vi "BAES RI Retrieval from PAS with LABVIEW.vi"() -> ()   [LabVIEW 2013]
uses:
  BaesDataTypeDefinition.ctl
  ReadBaesDataTypeDefinition.ctl
  ParticleDistributionData.ctl
  GeneralDataForRIRetrieval.ctl
  <vilib>/Native 3D Graph/xcontrol/3DPC_SurfacePlot.xctl
  <vilib>/Native 3D Graph/classes/Surface/Surface.lvclass
  RIandRIMCResults.ctl
  <vilib>/gmath/NumericalOptimization/stopping criteria.ctl
  <vilib>/Analysis/1siggen.llb/Ramp Pattern by Samples.vi
  <vilib>/gmath/NumericalOptimization/Conjugate Gradient.vi
  <vilib>/Utility/file.llb/Write To Spreadsheet File (string).vi
  <vilib>/Analysis/Matrix/Numeric/Conversions/Matrix To Array - RM.vi
  <vilib>/gmath/statdist.llb/Normal Inverse CDF.vi
  <vilib>/imath/engines/lvmath2/RunTimeEngine/ErrorHandling/NIMS_Finalize Error.vi
  <vilib>/imath/engines/lvmath2/RunTimeEngine/RangeToken/NIMS_Range_R2 - Float.vi
  <instcachedir>/0/NIMS_Range_R2 - Float_E19924E36A3948A4B33043226480F83C.lvgen/NIMS_Range_R2 - Float_E19924E36A3948A4B33043226480F83C_000.vi
  <vilib>/imath/engines/lvmath2/RunTimeEngine/NodeEndStatement/NIMS_NodeEndStatement_Output.vi
  <instcachedir>/0/NIMS_NodeEndStatement_Output_53EC0D466D134D7ABD903AC30B43404B.lvgen/NIMS_NodeEndStatement_Output_53EC0D466D134D7ABD903AC30B43404B_002.vi
  <vilib>/imath/engines/lvmath2/RunTimeEngine/CommandStatement/MC_CommandStatement_break.vi
  <vilib>/imath/engines/lvmath2/RunTimeSupport/NIMS_Error if Not Equal.vi
  <instcachedir>/0/NIMS_Error if Not Equal_902F5D2649E64F5087A1EF57C55C58AB.lvgen/NIMS_Error if Not Equal_902F5D2649E64F5087A1EF57C55C58AB_000.vi
  <vilib>/imath/engines/lvmath2/RunTimeEngine/IndexRead/NIMS M($,S).vi
  <instcachedir>/0/NIMS M($,S)_3E5749BBB62E49528D4765A77F1F6D98.lvgen/NIMS M($,S)_3E5749BBB62E49528D4765A77F1F6D98_000.vi
  <vilib>/imath/engines/lvmath2/RunTimeEngine/RowToken/NIMS_RowToken_M_CV.vi
  <instcachedir>/0/NIMS_RowToken_M_CV_4FFFB80A1A2C4A06BEF1E2564C6BAFA4.lvgen/NIMS_RowToken_M_CV_4FFFB80A1A2C4A06BEF1E2564C6BAFA4_000.vi
  <vilib>/imath/engines/lvmath2/RunTimeEngine/ErrorHandling/NIMS_Create Error From Enums.vi
  <vilib>/gmath/NI_Gmath.lvlib
  <vilib>/Analysis/Matrix/NI_Matrix.lvlib
  <vilib>/Analysis/NI_AALBase.lvlib
panel:
  out "Array":dbl[][](array[numeric])
  out "Global Min":T1
  out "GlobalMinimumStruct":T2(array[cluster])
  out "n-k matrix":cluster{dbl[], dbl[]}(graph)
  in  "k_samples":dbl=1.0 caption="Samples"
  in  "k_finish":dbl=5.0 caption="Finish"
  in  "k_start":dbl=-5.0 caption="Start"
  in  "n_samples":dbl=0.1 caption="Samples"
  in  "n_finish":dbl=1.2 caption="Finish"
  in  "n_start":dbl=0.8 caption="Start"
  in  "Find Global Minima":bool
  in  "Starting Guess - Imag":dbl=0.1
  in  "Starting Guess -Real":dbl=1.5
  in  "autoscale":bool
  in  "Correct SMPS sizes to selected Sizes":bool
  out "Peak Center":dbl[](array[numeric])=[215.23700286959917, 239.46777469280113, 266.53712087613405, 296.56972011152817, 329.9933867048781, 354.3213922159785, 380.24064147372457, 407.9273850466716, 436.86507564817134]
  in  "method":i32(ring)=3 items=["nearest", "linear", "spline", "cubic Hermite", "Lagrange"]
  out "yi out":dbl[][](array[numeric])=[[0.0, 0.0, 0.0, 0.0, 0.0, 0.0, 0.0, 0.0, 0.0], [0.0, 0.0, 0.0, 0.0, 0.0, 0.0, 0.0, 0.0, 0.0], [0.0, 0.0, 0.0, 0.0, 0.0, 0.0, 0.0, 0.0, 0.0], [0.0, 0.0, 0.0, 0.0, 0.0, 0.0, 0.0, 0.0, 0.0], [0.0, 0.0, 0.0, 0.0, 0.0, 0.0, 0.0, 0.0, 0.0], [0.0, 0.0, 0.0, 0.0, 0.0, 0.0, 0.0, 0.0, 0.0], [0.0, 0.0, 0.0, 0.0, 0.0, 0.0, 0.0, 0.0, 0.0], [0.0, 0.0, 0.0, 0.0, 0.0, 0.0, 0.0, 0.0, 0.0], [0.0, 0.0, 0.0, 0.0, 0.0, 0.0, 0.0, 0.0, 0.0], [0.0, 0.0, 0.0, 0.0, 0.0, 0.0, 0.0, 0.0, 0.0], [0.0, 0.0, 0.0, 0.0, 0.0, 0.0, 0.0, 0.0, 0.0], [0.0, 0.0, 0.0, 0.0, 0.0, 0.0, 0.0, 0.0, 0.0], [0.0, 0.0, 0.0, 0.0, 0.0, 0.0, 0.0, 0.0, 0.0], [0.0, 0.0, 0.0, 0.0, 0.0, 0.0, 0.0, 0.0, 0.0], [0.0, 0.0, 0.0, 0.0, 0.0, 0.0, 0.0, 0.0, 0.0], [0.0, 0.0, 0.0, 0.0, 0.0, 0.0, 0.0, 0.0, 0.0], [0.002995533043634161, 0.0, 0.0, 0.0, 0.0, 0.0, 0.0, 0.0, 0.0], [0.025840856539342556, 0.0, 0.0, 0.0, 0.0, 0.0, 0.0, 0.0, 0.0], [0.09627433030958367, 0.0, 0.0, 0.0, 0.0, 0.0, 0.0, 0.0, 0.0], [0.20114413818462407, 0.003679405258454903, 0.0, 0.0, 0.0, 0.0, 0.0, 0.0, 0.0], [0.24542760207823705, 0.030110785948579594, 0.0, 0.0, 0.0, 0.0, 0.0, 0.0, 0.0], [0.19935011876678227, 0.10676097365384078, 0.0, 0.0, 0.0, 0.0, 0.0, 0.0, 0.0], [0.10027077337218139, 0.21292413302969826, 0.0033748243651170722, 0.0, 0.0, 0.0, 0.0, 0.0, 0.0], [0.02900603131815543, 0.252436330373865, 0.02890039600275283, 0.0, 0.0, 0.0, 0.0, 0.0, 0.0], [0.0039798778324419744, 0.1962993842174311, 0.10425475468568692, 0.0, 0.0, 0.0, 0.0, 0.0, 0.0], [0.0, 0.09510810120556674, 0.2127509720448336, 0.003204303022032701, 0.0, 0.0, 0.0, 0.0, 0.0], [0.0, 0.026788275767934952, 0.25443516550640577, 0.028222420464123123, 0.0, 0.0, 0.0, 0.0, 0.0], [0.0, 0.0036138798422305257, 0.20572070395413536, 0.10336691645150534, 0.0, 0.0, 0.0, 0.0, 0.0], [0.0, 0.0, 0.10385751888143922, 0.21356874773842194, 0.003345015757771727, 0.0, 0.0, 0.0, 0.0], [0.0, 0.0, 0.03184137129301377, 0.25514474611865134, 0.02938228217938827, 0.0, 0.0, 0.0, 0.0], [0.0014956304497509467, 0.0, 0.005324689051489316, 0.21179320089555217, 0.10705199934528585, 0.003308736710887511, 0.0, 0.0, 0.0], [0.006181204689297098, 0.0, 0.0, 0.10947088728935564, 0.21880478513266646, 0.029404152563977024, 0.0, 0.0, 0.0], [0.014779079751943505, 0.0, 0.0, 0.0351443521735081, 0.2573967125709004, 0.10811744003531051, 0.004055473967709127, 0.0, 0.0], [0.021873123606276416, 0.0, 0.0, 0.00645421284142625, 0.21311979554910082, 0.21949012820871305, 0.03249660231234976, 0.0, 0.0], [0.020938671287516166, 0.002941447778294588, 0.0, 0.0005784696243201418, 0.11000745576713801, 0.2570127905092043, 0.11420156491259865, 0.004251138588627886, 0.0], [0.014150903231161319, 0.00918486371676828, 0.0, 0.0, 0.036185400505208645, 0.21598258772382448, 0.22683349675845424, 0.03241034304426709, 0.0], [0.005998151011193356, 0.016563944732687075, 0.0, 0.0, 0.007021566470141746, 0.11238428494392888, 0.25641274621663857, 0.11266793086437756, 0.004147715999403451], [0.0015120995486811858, 0.017797923247623602, 0.001492807625783663, 0.0, 0.0007094205616598339, 0.037396339870968194, 0.21111602466052512, 0.22428037538775147, 0.031085439808444255], [0.0, 0.01329593538708705, 0.005201029958243257, 0.0, 0.0, 0.007536234728094553, 0.10787117985635983, 0.25568882442612334, 0.11065902188610582], [0.0, 0.00635541490586478, 0.010415971194231972, 0.0, 0.0, 0.0008190951722994508, 0.03536648135652447, 0.21469636352155314, 0.2221123992215679], [0.0010729774499575713, 0.0019363898629268694, 0.01277891881575932, 0.0006807013617405569, 0.0, 0.0, 0.007025068509258474, 0.10969810395513567, 0.25508407775997943], [0.002057300309839938, 0.0, 0.010740838502774176, 0.002649342768284491, 0.0, 0.0, 0.0007440549395453882, 0.03615143628832095, 0.216785934587122], [0.002474950875894475, 0.0, 0.006120821318984597, 0.006052131853820764, 0.0, 0.0, 0.0, 0.007394514918229318, 0.11122539130067338], [0.002060729815382503, 0.0, 0.002286068305636173, 0.008519468407529212, 0.0, 0.0, 0.0, 0.0008550654797584019, 0.03853326504170029], [0.0011159165281229126, 0.0009250356514019637, 0.0005031484937129974, 0.007827186354841077, 0.0010483084611445424, 0.0, 0.0, 0.0, 0.008221211137071305], [0.0, 0.0013182032160797494, 0.0, 0.0048751624944381525, 0.002846930380238516, 0.0, 0.0, 0.0, 0.0009934611660537788], [0.0, 0.0011832812074649155, 0.0, 0.0019419202748162476, 0.004454066932151218, 0.0, 0.0, 0.0, 0.0], [0.0, 0.0007762909961994142, 0.0, 0.0005058298656327597, 0.004488441198541657, 0.001576949269729668, 0.0, 0.0, 0.0], [0.0, 0.0, 0.0, 0.0, 0.0029347814148206284, 0.002346089545272472, 0.0, 0.0, 0.0], [0.0, 0.0, 0.0, 0.0, 0.0012030377738417415, 0.00231674366991226, 0.0007291026037730795, 0.0, 0.0], [0.0, 0.0, 0.0, 0.0, 0.0, 0.0015886617028698508, 0.0011333656105798114, 0.0, 0.0], [0.0, 0.0, 0.0, 0.0, 0.0, 0.0007197653450079487, 0.0011589853888717718, 0.0, 0.0], [0.0, 0.0, 0.0, 0.0, 0.0, 0.0, 0.0008558529068117928, 0.0005237679257223164, 0.0], [0.0, 0.0, 0.0, 0.0, 0.0, 0.0, 0.0, 0.0007042968505584731, 0.0], [0.0, 0.0, 0.0, 0.0, 0.0, 0.0, 0.0, 0.000677838749574469, 0.0], [0.0, 0.0, 0.0, 0.0, 0.0, 0.0, 0.0, 0.0, 0.000518938219565122], [0.0, 0.0, 0.0, 0.0, 0.0, 0.0, 0.0, 0.0, 0.0006331438723132111]]
  out "SMPS":T3(graph)=[{"Ramp Pattern"=[105.5, 109.4, 113.4, 117.6, 121.9, 126.3, 131.0, 135.8, 140.7, 145.9, 151.2, 156.8, 162.5, 168.5, 174.7, 181.1, 187.7, 194.6, 201.7, 209.1, 216.7, 224.7, 232.9, 241.4, 250.3, 259.5, 269.0, 278.8, 289.0, 299.6, 310.6, 322.0, 333.8, 346.0, 358.7, 371.8, 385.4, 399.5, 414.2, 429.4, 445.1, 461.4, 478.3, 495.8, 514.0, 532.8, 552.3, 572.5, 593.5, 615.3, 637.8, 661.2, 685.4, 710.5, 736.5, 763.5, 791.5], "Extinction"=[0.0, 0.0, 0.0, 0.0, 0.0, 0.0, 0.0, 0.0, 0.0, 0.0, 0.0, 0.0, 0.0, 0.0, 0.0, 0.0, 0.0, 0.0, 0.0, 0.0, 0.0, 0.0, 0.0, 0.0, 0.0, 0.0, 0.0, 0.0, 0.0, 0.0, 0.0, 0.0, 0.0, 0.0, 0.0, 0.0, 0.004147715999403451, 0.031085439808444255, 0.11065902188610582, 0.2221123992215679, 0.25508407775997943, 0.216785934587122, 0.11122539130067338, 0.03853326504170029, 0.008221211137071305, 0.0009934611660537788, 0.0, 0.0, 0.0, 0.0, 0.0, 0.0, 0.0, 0.0, 0.0, 0.000518938219565122, 0.0006331438723132111]}, {"Ramp Pattern"=[105.5, 109.4, 113.4, 117.6, 121.9, 126.3, 131.0, 135.8, 140.7, 145.9, 151.2, 156.8, 162.5, 168.5, 174.7, 181.1, 187.7, 194.6, 201.7, 209.1, 216.7, 224.7, 232.9, 241.4, 250.3, 259.5, 269.0, 278.8, 289.0, 299.6, 310.6, 322.0, 333.8, 346.0, 358.7, 371.8, 385.4, 399.5, 414.2, 429.4, 445.1, 461.4, 478.3, 495.8, 514.0, 532.8, 552.3, 572.5, 593.5, 615.3, 637.8, 661.2, 685.4, 710.5, 736.5, 763.5, 791.5], "Extinction"=[0.0, 0.0, 0.0, 0.0, 0.0, 0.0, 0.0, 0.0, 0.0, 0.0, 0.0, 0.0, 0.0, 0.0, 0.0, 0.0, 0.0, 0.0, 0.0, 0.0, 0.0, 0.0, 0.0, 0.0, 0.0, 0.0, 0.0, 0.0, 0.0, 0.0, 0.0, 0.0, 0.0, 0.0, 0.0, 0.000717254, 0.0123831, 0.0638696, 0.166954, 0.256206, 0.250783, 0.158589, 0.0675111, 0.0180047, 0.00271755, 0.000182617, 0.0, 0.0, 0.0, 0.0, 0.0, 1.197e-05, 6.86901e-05, 0.000249565, 0.000468067, 0.00056712, 0.000716313]}]
  in  "ShiftSMPStoSizes":bool
  out "Size Distribution":T3(graph)=[{"Ramp Pattern"=[105.5, 109.4, 113.4, 117.6, 121.9, 126.3, 131.0, 135.8, 140.7, 145.9, 151.2, 156.8, 162.5, 168.5, 174.7, 181.1, 187.7, 194.6, 201.7, 209.1, 216.7, 224.7, 232.9, 241.4, 250.3, 259.5, 269.0, 278.8, 289.0, 299.6, 310.6, 322.0, 333.8, 346.0, 358.7, 371.8, 385.4, 399.5, 414.2, 429.4, 445.1, 461.4, 478.3, 495.8, 514.0, 532.8, 552.3, 572.5, 593.5, 615.3, 637.8, 661.2, 685.4, 710.5, 736.5, 763.5, 791.5], "Extinction"=[0.0, 0.0, 0.0, 0.0, 0.0, 0.0, 0.0, 0.0, 0.0, 0.0, 0.00602144, 0.0440621, 0.137641, 0.242033, 0.26037, 0.1769, 0.0750014, 0.0175727, 0.00179137, 0.0, 0.0, 0.0, 0.0, 0.000380957, 0.00237282, 0.00642719, 0.0101183, 0.00943116, 0.0057312, 0.00222174, 0.000458212, 6.03629e-05, 0.000103363, 0.000252222, 0.000379412, 0.000345309, 0.000218451, 8.10505e-05, 2.25477e-05, 2.37179e-06, 2.10622e-07, 0.0, 0.0, 0.0, 0.0, 0.0, 0.0, 0.0, 0.0, 0.0, 0.0, 0.0, 0.0, 0.0, 0.0, 0.0, 0.0]}, {"Ramp Pattern"=[105.5, 109.4, 113.4, 117.6, 121.9, 126.3, 131.0, 135.8, 140.7, 145.9, 151.2, 156.8, 162.5, 168.5, 174.7, 181.1, 187.7, 194.6, 201.7, 209.1, 216.7, 224.7, 232.9, 241.4, 250.3, 259.5, 269.0, 278.8, 289.0, 299.6, 310.6, 322.0, 333.8, 346.0, 358.7, 371.8, 385.4, 399.5, 414.2, 429.4, 445.1, 461.4, 478.3, 495.8, 514.0, 532.8, 552.3, 572.5, 593.5, 615.3, 637.8, 661.2, 685.4, 710.5, 736.5, 763.5, 791.5], "Extinction"=[0.0, 0.0, 0.0, 0.0, 0.0, 0.0, 0.0, 0.0, 0.0, 0.0, 0.0, 0.0, 0.0, 0.0, 0.00687402, 0.0480765, 0.147169, 0.249643, 0.264176, 0.173705, 0.0710016, 0.0162594, 0.00162783, 0.0, 0.0, 0.0, 0.0, 0.000166187, 0.00111154, 0.00332619, 0.00527313, 0.0051977, 0.00371407, 0.00163836, 0.000493174, 8.35816e-05, 1.90248e-05, 4.61745e-05, 0.000101968, 8.69849e-05, 8.92941e-05, 7.65637e-05, 3.07908e-05, 1.04858e-05, 1.81277e-06, 1.23923e-07, 0.0, 0.0, 0.0, 0.0, 0.0, 0.0, 0.0, 0.0, 0.0, 0.0, 0.0]}, {"Ramp Pattern"=[105.5, 109.4, 113.4, 117.6, 121.9, 126.3, 131.0, 135.8, 140.7, 145.9, 151.2, 156.8, 162.5, 168.5, 174.7, 181.1, 187.7, 194.6, 201.7, 209.1, 216.7, 224.7, 232.9, 241.4, 250.3, 259.5, 269.0, 278.8, 289.0, 299.6, 310.6, 322.0, 333.8, 346.0, 358.7, 371.8, 385.4, 399.5, 414.2, 429.4, 445.1, 461.4, 478.3, 495.8, 514.0, 532.8, 552.3, 572.5, 593.5, 615.3, 637.8, 661.2, 685.4, 710.5, 736.5, 763.5, 791.5], "Extinction"=[0.0, 0.0, 0.0, 0.0, 0.0, 0.0, 0.0, 0.0, 0.0, 0.0, 0.0, 0.0, 0.0, 0.0, 0.0, 0.0, 0.0, 0.00757534, 0.0522276, 0.153098, 0.255401, 0.261513, 0.171607, 0.06944, 0.0155384, 0.00150183, 0.0, 0.0, 0.0, 0.0, 5.24662e-05, 0.000401124, 0.00141094, 0.00259007, 0.00315663, 0.00238755, 0.00124251, 0.000361362, 7.04175e-05, 5.42399e-06, 1.1079e-05, 4.48726e-05, 7.59732e-05, 0.000110823, 9.47056e-05, 4.77246e-05, 2.73822e-05, 6.3375e-06, 7.95987e-07, 0.0, 0.0, 0.0, 0.0, 0.0, 0.0, 0.0, 0.0]}, {"Ramp Pattern"=[105.5, 109.4, 113.4, 117.6, 121.9, 126.3, 131.0, 135.8, 140.7, 145.9, 151.2, 156.8, 162.5, 168.5, 174.7, 181.1, 187.7, 194.6, 201.7, 209.1, 216.7, 224.7, 232.9, 241.4, 250.3, 259.5, 269.0, 278.8, 289.0, 299.6, 310.6, 322.0, 333.8, 346.0, 358.7, 371.8, 385.4, 399.5, 414.2, 429.4, 445.1, 461.4, 478.3, 495.8, 514.0, 532.8, 552.3, 572.5, 593.5, 615.3, 637.8, 661.2, 685.4, 710.5, 736.5, 763.5, 791.5], "Extinction"=[0.0, 0.0, 0.0, 0.0, 0.0, 0.0, 0.0, 0.0, 0.0, 0.0, 0.0, 0.0, 0.0, 0.0, 0.0, 0.0, 0.0, 0.0, 0.0, 0.0, 0.00835948, 0.0552173, 0.160029, 0.262073, 0.260519, 0.164631, 0.0664069, 0.0147714, 0.0015952, 3.75221e-05, 0.0, 0.0, 0.0, 0.0, 9.40175e-05, 0.00050349, 0.0012377, 0.00154137, 0.00141565, 0.000550918, 0.000265905, 0.000104568, 1.73682e-05, 5.50028e-06, 2.23782e-05, 5.44419e-05, 0.000136903, 0.00015264, 0.000138959, 7.38674e-05, 3.82305e-05, 5.70634e-06, 3.65588e-07, 0.0, 0.0, 0.0, 0.0]}, {"Ramp Pattern"=[105.5, 109.4, 113.4, 117.6, 121.9, 126.3, 131.0, 135.8, 140.7, 145.9, 151.2, 156.8, 162.5, 168.5, 174.7, 181.1, 187.7, 194.6, 201.7, 209.1, 216.7, 224.7, 232.9, 241.4, 250.3, 259.5, 269.0, 278.8, 289.0, 299.6, 310.6, 322.0, 333.8, 346.0, 358.7, 371.8, 385.4, 399.5, 414.2, 429.4, 445.1, 461.4, 478.3, 495.8, 514.0, 532.8, 552.3, 572.5, 593.5, 615.3, 637.8, 661.2, 685.4, 710.5, 736.5, 763.5, 791.5], "Extinction"=[0.0, 0.0, 0.0, 0.0, 0.0, 0.0, 0.0, 0.0, 0.0, 0.0, 0.0, 0.0, 0.0, 0.0, 0.0, 0.0, 0.0, 0.0, 0.0, 0.0, 0.0, 0.0, 0.0, 0.00767848, 0.0517681, 0.150308, 0.253087, 0.259137, 0.171174, 0.0730947, 0.018553, 0.00239402, 0.00010448, 0.0, 0.0, 0.0, 0.0, 0.000119673, 0.000697988, 0.00199477, 0.0030044, 0.00318935, 0.00203459, 0.000774649, 0.000254696, 4.51771e-05, 6.98448e-06, 1.47059e-05, 4.08995e-05, 9.96706e-05, 0.000130666, 0.000118646, 0.000112016, 4.31269e-05, 1.63916e-05, 2.2522e-06, 5.24186e-07]}, {"Ramp Pattern"=[105.5, 109.4, 113.4, 117.6, 121.9, 126.3, 131.0, 135.8, 140.7, 145.9, 151.2, 156.8, 162.5, 168.5, 174.7, 181.1, 187.7, 194.6, 201.7, 209.1, 216.7, 224.7, 232.9, 241.4, 250.3, 259.5, 269.0, 278.8, 289.0, 299.6, 310.6, 322.0, 333.8, 346.0, 358.7, 371.8, 385.4, 399.5, 414.2, 429.4, 445.1, 461.4, 478.3, 495.8, 514.0, 532.8, 552.3, 572.5, 593.5, 615.3, 637.8, 661.2, 685.4, 710.5, 736.5, 763.5, 791.5], "Extinction"=[0.0, 0.0, 0.0, 0.0, 0.0, 0.0, 0.0, 0.0, 0.0, 0.0, 0.0, 0.0, 0.0, 0.0, 0.0, 0.0, 0.0, 0.0, 0.0, 0.0, 0.0, 0.0, 0.0, 0.0, 0.0, 0.00802862, 0.0539198, 0.153628, 0.250466, 0.260125, 0.172954, 0.0721136, 0.0180011, 0.00240611, 0.000123353, 0.0, 0.0, 0.0, 0.0, 6.04674e-05, 0.000376547, 0.00114026, 0.00180722, 0.00163893, 0.00132501, 0.00066091, 0.000279576, 6.083e-05, 7.52492e-06, 8.24359e-06, 3.3625e-05, 8.24983e-05, 0.000193618, 0.000183914, 0.000186577, 8.98053e-05, 9.87749e-05]}, {"Ramp Pattern"=[105.5, 109.4, 113.4, 117.6, 121.9, 126.3, 131.0, 135.8, 140.7, 145.9, 151.2, 156.8, 162.5, 168.5, 174.7, 181.1, 187.7, 194.6, 201.7, 209.1, 216.7, 224.7, 232.9, 241.4, 250.3, 259.5, 269.0, 278.8, 289.0, 299.6, 310.6, 322.0, 333.8, 346.0, 358.7, 371.8, 385.4, 399.5, 414.2, 429.4, 445.1, 461.4, 478.3, 495.8, 514.0, 532.8, 552.3, 572.5, 593.5, 615.3, 637.8, 661.2, 685.4, 710.5, 736.5, 763.5, 791.5], "Extinction"=[0.0, 0.0, 0.0, 0.0, 0.0, 0.0, 0.0, 0.0, 0.0, 0.0, 0.0, 0.0, 0.0, 0.0, 0.0, 0.0, 0.0, 0.0, 0.0, 0.0, 0.0, 0.0, 0.0, 0.0, 0.0, 0.0, 0.0, 0.00848305, 0.0549652, 0.15814, 0.257902, 0.258945, 0.166212, 0.0688298, 0.0176995, 0.00246799, 0.000136758, 0.0, 0.0, 0.0, 0.0, 2.1648e-05, 0.000163604, 0.00046293, 0.000978937, 0.00118969, 0.00123218, 0.000718642, 0.000276316, 0.000101712, 1.82822e-05, 4.68561e-06, 3.19059e-05, 8.78095e-05, 0.000226048, 0.000257225, 0.00044707]}, {"Ramp Pattern"=[105.5, 109.4, 113.4, 117.6, 121.9, 126.3, 131.0, 135.8, 140.7, 145.9, 151.2, 156.8, 162.5, 168.5, 174.7, 181.1, 187.7, 194.6, 201.7, 209.1, 216.7, 224.7, 232.9, 241.4, 250.3, 259.5, 269.0, 278.8, 289.0, 299.6, 310.6, 322.0, 333.8, 346.0, 358.7, 371.8, 385.4, 399.5, 414.2, 429.4, 445.1, 461.4, 478.3, 495.8, 514.0, 532.8, 552.3, 572.5, 593.5, 615.3, 637.8, 661.2, 685.4, 710.5, 736.5, 763.5, 791.5], "Extinction"=[0.0, 0.0, 0.0, 0.0, 0.0, 0.0, 0.0, 0.0, 0.0, 0.0, 0.0, 0.0, 0.0, 0.0, 0.0, 0.0, 0.0, 0.0, 0.0, 0.0, 0.0, 0.0, 0.0, 0.0, 0.0, 0.0, 0.0, 0.0, 0.0, 0.0092548, 0.0597518, 0.165281, 0.258006, 0.253644, 0.163443, 0.0670374, 0.0164945, 0.00236907, 0.000132584, 0.0, 0.0, 0.0, 0.0, 0.0, 4.48073e-05, 0.000235896, 0.00070573, 0.00102449, 0.000940377, 0.000855458, 0.000432721, 0.000146615, 4.53709e-05, 7.09402e-06, 2.21239e-05, 4.11624e-05, 8.35608e-05]}, {"Ramp Pattern"=[105.5, 109.4, 113.4, 117.6, 121.9, 126.3, 131.0, 135.8, 140.7, 145.9, 151.2, 156.8, 162.5, 168.5, 174.7, 181.1, 187.7, 194.6, 201.7, 209.1, 216.7, 224.7, 232.9, 241.4, 250.3, 259.5, 269.0, 278.8, 289.0, 299.6, 310.6, 322.0, 333.8, 346.0, 358.7, 371.8, 385.4, 399.5, 414.2, 429.4, 445.1, 461.4, 478.3, 495.8, 514.0, 532.8, 552.3, 572.5, 593.5, 615.3, 637.8, 661.2, 685.4, 710.5, 736.5, 763.5, 791.5], "Extinction"=[0.0, 0.0, 0.0, 0.0, 0.0, 0.0, 0.0, 0.0, 0.0, 0.0, 0.0, 0.0, 0.0, 0.0, 0.0, 0.0, 0.0, 0.0, 0.0, 0.0, 0.0, 0.0, 0.0, 0.0, 0.0, 0.0, 0.0, 0.0, 0.0, 0.0, 0.0, 0.00772542, 0.0512686, 0.147448, 0.246257, 0.259558, 0.17471, 0.077618, 0.0214873, 0.00339646, 0.000233358, 0.0, 0.0, 0.0, 0.0, 0.0, 0.000122868, 0.000666115, 0.00177206, 0.00283796, 0.00236991, 0.00152854, 0.000757217, 0.000197087, 4.12075e-05, 3.97597e-06, 0.0]}, {"Ramp Pattern"=[105.5, 109.4, 113.4, 117.6, 121.9, 126.3, 131.0, 135.8, 140.7, 145.9, 151.2, 156.8, 162.5, 168.5, 174.7, 181.1, 187.7, 194.6, 201.7, 209.1, 216.7, 224.7, 232.9, 241.4, 250.3, 259.5, 269.0, 278.8, 289.0, 299.6, 310.6, 322.0, 333.8, 346.0, 358.7, 371.8, 385.4, 399.5, 414.2, 429.4, 445.1, 461.4, 478.3, 495.8, 514.0, 532.8, 552.3, 572.5, 593.5, 615.3, 637.8, 661.2, 685.4, 710.5, 736.5, 763.5, 791.5], "Extinction"=[0.0, 0.0, 0.0, 0.0, 0.0, 0.0, 0.0, 0.0, 0.0, 0.0, 0.0, 0.0, 0.0, 0.0, 0.0, 0.0, 0.0, 0.0, 0.0, 0.0, 0.0, 0.0, 0.0, 0.0, 0.0, 0.0, 0.0, 0.0, 0.0, 0.0, 0.0, 0.0, 0.000249452, 0.0092546, 0.0554075, 0.155262, 0.248347, 0.255494, 0.170831, 0.0745962, 0.0203161, 0.00332439, 0.00023658, 0.0, 0.0, 0.0, 0.0, 0.0, 6.91964e-05, 0.000434111, 0.000981635, 0.00149811, 0.00169063, 0.00103972, 0.000591012, 0.000238787, 0.00013861]}, {"Ramp Pattern"=[105.5, 109.4, 113.4, 117.6, 121.9, 126.3, 131.0, 135.8, 140.7, 145.9, 151.2, 156.8, 162.5, 168.5, 174.7, 181.1, 187.7, 194.6, 201.7, 209.1, 216.7, 224.7, 232.9, 241.4, 250.3, 259.5, 269.0, 278.8, 289.0, 299.6, 310.6, 322.0, 333.8, 346.0, 358.7, 371.8, 385.4, 399.5, 414.2, 429.4, 445.1, 461.4, 478.3, 495.8, 514.0, 532.8, 552.3, 572.5, 593.5, 615.3, 637.8, 661.2, 685.4, 710.5, 736.5, 763.5, 791.5], "Extinction"=[0.0, 0.0, 0.0, 0.0, 0.0, 0.0, 0.0, 0.0, 0.0, 0.0, 0.0, 0.0, 0.0, 0.0, 0.0, 0.0, 0.0, 0.0, 0.0, 0.0, 0.0, 0.0, 0.0, 0.0, 0.0, 0.0, 0.0, 0.0, 0.0, 0.0, 0.0, 0.0, 0.0, 0.0, 0.00047746, 0.0109443, 0.0594236, 0.159472, 0.250859, 0.251764, 0.164306, 0.0735026, 0.0204329, 0.00317896, 0.000231652, 0.0, 0.0, 0.0, 0.0, 0.0, 3.3009e-05, 0.000198918, 0.000613343, 0.00089841, 0.00119029, 0.00119749, 0.00127579]}, {"Ramp Pattern"=[105.5, 109.4, 113.4, 117.6, 121.9, 126.3, 131.0, 135.8, 140.7, 145.9, 151.2, 156.8, 162.5, 168.5, 174.7, 181.1, 187.7, 194.6, 201.7, 209.1, 216.7, 224.7, 232.9, 241.4, 250.3, 259.5, 269.0, 278.8, 289.0, 299.6, 310.6, 322.0, 333.8, 346.0, 358.7, 371.8, 385.4, 399.5, 414.2, 429.4, 445.1, 461.4, 478.3, 495.8, 514.0, 532.8, 552.3, 572.5, 593.5, 615.3, 637.8, 661.2, 685.4, 710.5, 736.5, 763.5, 791.5], "Extinction"=[0.0, 0.0, 0.0, 0.0, 0.0, 0.0, 0.0, 0.0, 0.0, 0.0, 0.0, 0.0, 0.0, 0.0, 0.0, 0.0, 0.0, 0.0, 0.0, 0.0, 0.0, 0.0, 0.0, 0.0, 0.0, 0.0, 0.0, 0.0, 0.0, 0.0, 0.0, 0.0, 0.0, 0.0, 0.0, 0.0, 0.000894806, 0.0133626, 0.0654787, 0.165378, 0.248596, 0.251094, 0.163896, 0.0678348, 0.0186113, 0.00296553, 0.000216825, 0.0, 0.0, 0.0, 0.0, 0.0, 1.64374e-05, 9.91911e-05, 0.000315671, 0.000542635, 0.000697866]}, {"Ramp Pattern"=[105.5, 109.4, 113.4, 117.6, 121.9, 126.3, 131.0, 135.8, 140.7, 145.9, 151.2, 156.8, 162.5, 168.5, 174.7, 181.1, 187.7, 194.6, 201.7, 209.1, 216.7, 224.7, 232.9, 241.4, 250.3, 259.5, 269.0, 278.8, 289.0, 299.6, 310.6, 322.0, 333.8, 346.0, 358.7, 371.8, 385.4, 399.5, 414.2, 429.4, 445.1, 461.4, 478.3, 495.8, 514.0, 532.8, 552.3, 572.5, 593.5, 615.3, 637.8, 661.2, 685.4, 710.5, 736.5, 763.5, 791.5], "Extinction"=[0.0, 0.0, 0.0, 0.0, 0.0, 0.0, 0.0, 0.0, 0.0, 0.0, 0.0, 0.0, 0.0, 0.0, 0.0, 0.0, 0.0, 0.0, 0.0, 0.0, 0.0, 0.0, 0.0, 0.0, 0.0, 0.0, 0.0, 0.0, 0.0, 0.0, 0.0, 0.0, 0.0, 0.0, 0.0, 0.0, 0.0, 0.0, 0.00125744, 0.0155736, 0.0701833, 0.175204, 0.260282, 0.240605, 0.153081, 0.0638767, 0.017253, 0.00250006, 0.000183834, 0.0, 0.0, 0.0, 0.0, 0.0, 0.0, 0.0, 0.0]}]
  out "Extinction Data per size":T3(graph)=[{"Ramp Pattern"=[404.0], "Extinction"=[0.0002939]}, {"Ramp Pattern"=[404.0, 404.0, 404.0], "Extinction"=[nan, 0.00029775799999999996, 0.000290042]}, {"Ramp Pattern"=[404.0], "Extinction"=[0.0002526]}, {"Ramp Pattern"=[404.0, 404.0, 404.0], "Extinction"=[nan, 0.00025647100000000003, 0.000248729]}, {"Ramp Pattern"=[404.0], "Extinction"=[0.000213]}, {"Ramp Pattern"=[404.0, 404.0, 404.0], "Extinction"=[nan, 0.000216884, 0.000209116]}, {"Ramp Pattern"=[404.0], "Extinction"=[0.0001739]}, {"Ramp Pattern"=[404.0, 404.0, 404.0], "Extinction"=[nan, 0.00017775699999999999, 0.000170043]}, {"Ramp Pattern"=[404.0], "Extinction"=[0.0003827]}, {"Ramp Pattern"=[404.0, 404.0, 404.0], "Extinction"=[nan, 0.00038661999999999995, 0.00037878]}, {"Ramp Pattern"=[404.0], "Extinction"=[0.0003375]}, {"Ramp Pattern"=[404.0, 404.0, 404.0], "Extinction"=[nan, 0.000341367, 0.000333633]}, {"Ramp Pattern"=[404.0], "Extinction"=[0.0002773]}, {"Ramp Pattern"=[404.0, 404.0, 404.0], "Extinction"=[nan, 0.00028117100000000004, 0.000273429]}, {"Ramp Pattern"=[404.0], "Extinction"=[0.0002286]}, {"Ramp Pattern"=[404.0, 404.0, 404.0], "Extinction"=[nan, 0.000232492, 0.000224708]}, {"Ramp Pattern"=[404.0], "Extinction"=[0.0007247]}, {"Ramp Pattern"=[404.0, 404.0, 404.0], "Extinction"=[nan, 0.000728578, 0.000720822]}, {"Ramp Pattern"=[404.0], "Extinction"=[0.0006]}, {"Ramp Pattern"=[404.0, 404.0, 404.0], "Extinction"=[nan, 0.0006038599999999999, 0.00059614]}, {"Ramp Pattern"=[404.0], "Extinction"=[0.0004691]}, {"Ramp Pattern"=[404.0, 404.0, 404.0], "Extinction"=[nan, 0.000472931, 0.00046526900000000003]}, {"Ramp Pattern"=[404.0], "Extinction"=[0.0003841]}, {"Ramp Pattern"=[404.0, 404.0, 404.0], "Extinction"=[nan, 0.000387956, 0.000380244]}, {"Ramp Pattern"=[404.0], "Extinction"=[0.000303]}, {"Ramp Pattern"=[404.0, 404.0, 404.0], "Extinction"=[nan, 0.00030685099999999997, 0.000299149]}]
  out "Wavelength":string="WL=404.000nm"
  out "Imaginary Part":string="k=0.048±0.003"
  out "Real Part":string="n=1.612±0.017"
  in  "Quick Fit":bool=TRUE
  in  "Diameters to fit":i32[](listbox)=[11]
  out "Residue":dbl=nan
  in  "ExtinctionOrAbsorptionOrScattering":i8(knob)=1 scale=0.0..2.0
  in  "Plot RI":bool
  in  "k":dbl=0.042
  in  "n":dbl=1.668
  out "Residue (CDMRI)":dbl=8.570278477447328
  out "Wavelength":dbl=404.0 format="%.3g"
  out "Imaginary Uncertainty":dbl=0.0031250000000000028 caption="±" format="%.3g"
  out "Imaginary Part":dbl=0.047890347587708715 format="%.3g"
  out "Real Uncertainty":dbl=0.01718749999999991 caption="±" format="%.3g"
  out "Real part":dbl=1.6120396036585403 format="%.3g"
  out "Diameter Offset":dbl
  out "Diameter Factor":dbl=1.0
  out "Extinction Factor":dbl=1.0
  out "Residue (MDBF)":dbl=6.760282502809872
  out "Time Left (min)":dbl=22.74556666666667 format="%#.1f"
  out "Progress bar for Extinction search":u8(slide)=12 max=5 scale=-1.0..55.0
  in  "Diameter Factor Radio Button":bool
  in  "Diamter Offset Radio Button":bool=TRUE
  in  "Diameter FO Interval":dbl=1.0 caption="Interval"
  in  "Diameter FO Finish":dbl=5.0 caption="Finish"
  in  "Diameter FO start":dbl=-5.0 caption="Start"
  in  "Diameter Offset":dbl
  in  "Diameter Factor":dbl=1.0
  in  "Extinction Factor":dbl=1.2
  in  "Extinction Factor Interval":dbl=0.1 caption="Interval"
  in  "Extinction Factor Finish":dbl=1.2 caption="Finish"
  in  "Extinction Factor Start":dbl=0.8 caption="Start"
  in  "Find Extinction Factor Graph":bool
  out "3D Graph":refnum<class "Base Datatype.lvclass">[](xcontrol)
  in  "Use Factors":bool
  in  "Min Wavelength":string(combo)="0"
  in  "Max Wavelength":string(combo)="0"
  in  "Restrict to Positive Imaginary Part":bool
  in  "Calculate Errors":bool=TRUE
  in  "Approximate Errors":bool
  in  "Save RI":bool
  in  "Retrieve RI":bool
  in  "Mutiple Charge Data File":path=path "20141007 MCD Catechol+HNO3 CRD&PAS.txt"
  in  "Extinction Cross Section File":path=path "20141007 Catechol+HNO3 PAS data file without zero.txt"
  in  "Diameter Factor or Offset 2":bool=TRUE caption="Offset - True, Factor - OFF"
  out "Simplex":T4(graph)=[{"Size parameters"=[1.6120089713403827, 1.6118316452568249, 1.6120396036585403, 1.6120089713403827], "Normalized Residuals"=[0.04786302549244287, 0.04780448724122838, 0.047890347587708715, 0.04786302549244287]}]
  in  "Diameter Factor or Offset":bool=TRUE caption="Offset - True, Factor - OFF"
  in  "Minimization method":u16(ring)=1 items=["LM method", "Simplex Method"]
  in  "Extinction Factor in Data":dbl=1.0
  out "Residue Graph Matrix":dbl[][](array[numeric])=[[0.8817748876641518, 0.7943260267120898, 0.7221799384952265, 0.6683504995926692, 0.6311277469517097, 0.6088767086158524], [0.7307518731289654, 0.673042958848353, 0.6345421279928648, 0.6122901406297341, 0.6040701363961388, 0.6079500250191767], [0.6456146353159482, 0.6217239264490524, 0.6132715417472164, 0.6175167400813633, 0.6328117960393451, 0.6563665043893292], [0.6273068413741216, 0.6311010869376654, 0.6464620791865137, 0.671082182122829, 0.7034305368703453, 0.741845745993439], [0.6631237737749567, 0.6880232407171314, 0.7208560286150587, 0.7602689432195936, 0.8046376766720158, 0.8530494481747876]]
  out "Extinction Factor Results":cluster{dbl[], dbl[]}[](graph)=[{[0.8, 0.9, 1.0, 1.1, 1.2], [1.539671374334097, 1.5976213646223005, 1.5606320545412844, 1.5516397914476685, 1.5319499648100456]}, {[0.8, 0.9, 1.0, 1.1, 1.2], [-0.11096660801067405, -0.0653657766346238, -0.05966999471633491, -0.017727862931787984, 0.01906205546692944]}, {[0.8, 0.9, 1.0, 1.1, 1.2], [13.260187371616055, 8.444315776530917, 1.2615157523101117, 0.7276563123626676, 0.6329059597830448]}]
  in  "General Data for RI Retrieval VI":T5={"Min WaveLength Index"=0, "Max WaveLength Index"=0, "Extinction Factor"=FALSE, "Size Parameter Factor"=FALSE, "Size Paramter Offset"=FALSE, "Extinction Factor"=1.0, "Diameter Factor"=1.0, "Diameter Offset"=0.0, "ExtinctionOrAbsorptionOrScattering"=0} {"ExtinctionOrAbsorptionOrScattering" scale=0.0..2.0; "Max WaveLength Index" max=200 step=1; "Min WaveLength Index" max=200 step=1}
  in  "Graph Refs 2":T6
  in  "Size Parameter Offset":bool
  in  "Size Parameter Factor":bool
  in  "Extinction Factor":bool
  out "Minimized Size Parameter Factor":dbl
  out "Minimized Extinction Factor":dbl
  in  "Data for RIRetrieval VI":T9={"Approximate Errors"=FALSE, "Extinction ExtinctionUncertainity Size parameter and Number ofS sizes"={"Extinction"=[], "Extinction Uncertainty"=[], "Size parameters"=[], "Number ofSizes"=0.0, "GeometricCrossSection"=[], "WaveLength"=[], "Sizes"=[], "Concentration (#/cc)"=[]}, "Minimization method"=0, "Graph Ref"={"Real Part vs wavelength"=refnum, "Imaginary Part vs wavelength"=refnum, "Normalized Residuals vs Size parameter"=refnum, "Not Corrected for Multiple charge particles"=refnum, "Simplex 2"=refnum}, "Particle Distribution Data"={"SMPS Sizes"=[], "Concentration"=[], "Double Charge Correction Flag"=FALSE}, "Calculate Errors"=FALSE, "Restrict to Positive Imaginary Part"=FALSE, "MinMaxWavelength"={0, 0, "Extinction Factor"=FALSE, "Size Parameter Factor"=FALSE, "Size Parameter Offset"=TRUE, "Extinction Factor"=1.0, "Diameter Factor"=1.0, "Diameter Offset"=0.0, "ExtinctionOrAbsorptionOrScattering"=0}} {"MinMaxWavelength"."ExtinctionOrAbsorptionOrScattering" scale=0.0..2.0}
  in  "Graph Refs":T6
  in  "Factor Ext Uncertainty in Data":dbl=1.0
  in  "Save RI expanded Edition":bool
  out "Saved RI to this filename and path 2":path=path "Z:/Dropbox/Lior Segev/Lior Segev Projects/RI retrieval in Labview/Data/Ammonium Sulfate/20130724ForMatlabRetrival-RIresult.xls"
  out "index of element":i32
  out "Corrected for multiple charge particles":cluster{"Size parameters":dbl[], dbl[]}[](graph)=[{"Size parameters"=[1.3608384019262716, 1.5707963267948966, 1.7496493739052066, 1.9440548598946739, 2.169565223642456, 2.3328658318736086, 2.50394265954434, 2.6905719260942287, 2.8927536315232745, 3.1104877758314786, 3.3359981395792606, 3.584837161645779, 3.8570048420310328], [5.3875310220428614e-11, 9.625312389074256e-11, 1.4035340951398373e-10, 1.8444247381091288e-10, 2.5132005122927893e-10, 3.2845815503971793e-10, 4.2283407505353175e-10, 5.091912677743789e-10, 6.155250099337052e-10, 7.743388049575035e-10, 9.61353009684407e-10, 1.140559497937602e-09, 1.3954255339616367e-09]}, {"Size parameters"=[1.3608384019262716, 1.5707963267948966, 1.7496493739052066, 1.9440548598946739, 2.169565223642456, 2.3328658318736086, 2.50394265954434, 2.6905719260942287, 2.8927536315232745, 3.1104877758314786, 3.3359981395792606, 3.584837161645779, 3.8570048420310328], [6.178792893996032e-11, 1.0360347996174468e-10, 1.4599048359098532e-10, 1.894070733587938e-10, 2.6375374106990535e-10, 3.3972105684121345e-10, 4.3435802177249627e-10, 5.178882878098534e-10, 6.3749344691999e-10, 7.915454958151713e-10, 9.785475763024465e-10, 1.1461003257551283e-09, 1.3954254418635514e-09]}, {"Size parameters"=[1.0886707215410174, 1.1240680724299796, 1.1594654233189419, 1.194862774207904, 1.2302601250968663, 1.2656574759858286, 1.3010548268747906, 1.3364521777637528, 1.371849528652715, 1.4072468795416773, 1.4426442304306395, 1.4780415813196017, 1.513438932208564, 1.5488362830975262, 1.5842336339864884, 1.6196309848754507, 1.6550283357644129, 1.690425686653375, 1.7258230375423371, 1.7612203884312994, 1.7966177393202616, 1.8320150902092238, 1.867412441098186, 1.9028097919871483, 1.9382071428761105, 1.9736044937650727, 2.0090018446540348, 2.044399195542997, 2.079796546431959, 2.1151938973209217, 2.1505912482098837, 2.185988599098846, 2.221385949987808, 2.25678330087677, 2.2921806517657326, 2.3275780026546946, 2.362975353543657, 2.398372704432619, 2.4337700553215815, 2.4691674062105435, 2.504564757099506, 2.539962107988468, 2.5753594588774305, 2.6107568097663925, 2.6461541606553545, 2.681551511544317, 2.716948862433279, 2.7523462133222414, 2.7877435642112034, 2.823140915100166, 2.858538265989128, 2.8939356168780903, 2.9293329677670523, 2.9647303186560148, 3.000127669544977, 3.035525020433939, 3.0709223713229012, 3.1063197222118633, 3.1417170731008257, 3.1771144239897877, 3.21251177487875, 3.247909125767712, 3.2833064766566746, 3.3187038275456366, 3.3541011784345987, 3.389498529323561, 3.424895880212523, 3.4602932311014856, 3.4956905819904476, 3.53108793287941, 3.566485283768372, 3.6018826346573345, 3.6372799855462965, 3.672677336435259, 3.708074687324221, 3.743472038213183, 3.7788693891021454, 3.8142667399911074, 3.84966409088007, 3.885061441769032, 3.9204587926579944, 3.9558561435469564, 3.991253494435919, 4.026650845324881, 4.062048196213843, 4.097445547102805, 4.132842897991767, 4.168240248880729, 4.203637599769692, 4.239034950658654, 4.274432301547616, 4.309829652436578, 4.345227003325541, 4.380624354214503, 4.416021705103465, 4.451419055992427, 4.48681640688139, 4.522213757770352, 4.557611108659314, 4.593008459548276, 4.628405810437238], [2.3913425740088315e-11, 2.6829886031579392e-11, 3.002503712184464e-11, 3.352952089568505e-11, 3.737981549253529e-11, 4.1618583994047587e-11, 4.629364063704539e-11, 5.145714692392898e-11, 5.716147447491567e-11, 6.345463044980462e-11, 7.037277148988969e-11, 7.793096858404069e-11, 8.611192012634598e-11, 9.485584723206434e-11, 1.0405291719248494e-10, 1.1354389327199639e-10, 1.2312942694612925e-10, 1.3259445286045676e-10, 1.4173823215893589e-10, 1.5041170038549943e-10, 1.585441018301519e-10, 1.6616003951448163e-10, 1.7337786092253459e-10, 1.8039192269920282e-10, 1.874538112384035e-10, 1.9484366981105459e-10, 2.0285266382853755e-10, 2.117669093938486e-10, 2.218563345496154e-10, 2.3336791295262294e-10, 2.4651398435328815e-10, 2.6145978275022897e-10, 2.7829983722113706e-10, 2.970307495656506e-10, 3.175158671533888e-10, 3.3945442818949136e-10, 3.623686457154453e-10, 3.856151759668091e-10, 4.08455151173622e-10, 4.3015460482731994e-10, 4.5011282408151977e-10, 4.679789244938326e-10, 4.837029780247578e-10, 4.975344464073288e-10, 5.099522832388844e-10, 5.215802252771343e-10, 5.331004122496418e-10, 5.451984898213091e-10, 5.585272512076205e-10, 5.736962610366084e-10, 5.912661433459611e-10, 6.117409004912502e-10, 6.355496608745013e-10, 6.629970164027755e-10, 6.942008429850157e-10, 7.289971532821784e-10, 7.668404568534155e-10, 8.067331297673133e-10, 8.4723743038103e-10, 8.866180376330135e-10, 9.231310519238935e-10, 9.553801956826387e-10, 9.82641038118135e-10, 1.0049872946046262e-09, 1.0232116869882117e-09, 1.0385877205993815e-09, 1.0525947787943596e-09, 1.0666974818016422e-09, 1.0822158203577552e-09, 1.1002904426480051e-09, 1.1218824803147914e-09, 1.1478145917479424e-09, 1.178796036859687e-09, 1.215411782529824e-09, 1.258083519100677e-09, 1.3069437186887538e-09, 1.361661472758671e-09, 1.4212163938157042e-09, 1.483712349587316e-09, 1.5463411487231663e-09, 1.6056901842347923e-09, 1.6583847400158457e-09, 1.7019450500730398e-09, 1.7354157004228695e-09, 1.7595366894274368e-09, 1.776363265313721e-09, 1.7886191248371576e-09, 1.7991110155311867e-09, 1.8103511506147908e-09, 1.8244404671949277e-09, 1.843088280656811e-09, 1.8677148580552306e-09, 1.8995507604588807e-09, 1.9396910783592796e-09, 1.989093007310216e-09, 2.048476690249633e-09, 2.1181010007912023e-09, 2.1974232808531464e-09, 2.2846512102746423e-09, 2.376368871004218e-09, 2.4675201105853585e-09]}, {"Size parameters"=[1.3608384019262716, 1.3608384019262716, 1.3608384019262716, 1.5707963267948966, 1.5707963267948966, 1.5707963267948966, 1.7496493739052066, 1.7496493739052066, 1.7496493739052066, 1.9440548598946739, 1.9440548598946739, 1.9440548598946739, 2.169565223642456, 2.169565223642456, 2.169565223642456, 2.3328658318736086, 2.3328658318736086, 2.3328658318736086, 2.50394265954434, 2.50394265954434, 2.50394265954434, 2.6905719260942287, 2.6905719260942287, 2.6905719260942287, 2.8927536315232745, 2.8927536315232745, 2.8927536315232745, 3.1104877758314786, 3.1104877758314786, 3.1104877758314786, 3.3359981395792606, 3.3359981395792606, 3.3359981395792606, 3.584837161645779, 3.584837161645779, 3.584837161645779, 3.8570048420310328, 3.8570048420310328, 3.8570048420310328], [nan, 5.5024259055033474e-11, 5.2726361385823754e-11, nan, 9.87142010581738e-11, 9.379204672331131e-11, nan, 1.449801770345698e-10, 1.3572664199339764e-10, nan, 1.9357400915738067e-10, 1.7531093846444508e-10, nan, 2.5505420062025844e-10, 2.475859018382994e-10, nan, 3.3384755239745214e-10, 3.230687576819837e-10, nan, 4.318851439750764e-10, 4.137830061319871e-10, nan, 5.231295036973271e-10, 4.952530318514307e-10, nan, 6.194294931091818e-10, 6.116205267582287e-10, nan, 7.804227449620609e-10, 7.682548649529461e-10, nan, 9.709447139378434e-10, 9.517613054309706e-10, nan, 1.15721500259304e-09, 1.1239039932821642e-09, nan, 1.4199919592169381e-09, 1.3708591087063354e-09]}, {"Size parameters"=[1.3608384019262716, 1.5707963267948966, 1.7496493739052066, 1.9440548598946739, 2.169565223642456, 2.3328658318736086, 2.50394265954434, 2.6905719260942287, 2.8927536315232745, 3.1104877758314786, 3.3359981395792606, 3.584837161645779, 3.8570048420310328], [5.229386931230306e-11, 9.502694327010901e-11, 1.3904614563822324e-10, 1.9008289779595017e-10, 2.651062953023996e-10, 3.315677916154744e-10, 4.228373184045294e-10, 4.820590204280071e-10, 6.155250099337052e-10, 7.84284060522772e-10, 9.279484202646198e-10, 1.2583729882380478e-09, 1.3490131265208746e-09]}]
  out "Multiple charge correction term":cluster{"Size parameters":dbl[], dbl[]}(graph)={"Size parameters"=[1.3608384019262716, 1.5707963267948966, 1.7496493739052066, 1.9440548598946739, 2.169565223642456, 2.3328658318736086, 2.50394265954434, 2.6905719260942287, 2.8927536315232745, 3.1104877758314786, 3.3359981395792606, 3.584837161645779, 3.8570048420310328], [9.992581969119865e-12, 9.41668406349618e-12, 7.33504600450774e-12, 6.137690315289009e-12, 1.562576072992927e-11, 1.3967562889835254e-11, 1.415342569160354e-11, 1.1032092342172384e-11, 2.830702862739528e-11, 2.2380186802793915e-11, 2.2393109654854668e-11, 7.44720309477825e-12, 0.0]}
  in  "Baes data type definition":T10={"PAS amplitude"=[], "PAS amp Uncertainty"=[], "Size parameters"=[], "Number ofSizes"=0.0, "GeometricCrossSection"=[], "Wave Length"=0.0, "SMPS Sizes"=[], "Concentration"=[], "Double Charge Correction"=FALSE, "Extincation Factor"=1.0, "Diameter Factor"=1.0, "Diameter Offset"=0.0, "Extinction Factor Flag"=FALSE, "Diameter Factor Flag"=FALSE, "Diameter Offset Flag"=FALSE, "Sizes"=[], "ExtinctionOrAbsorptionOrScattering"=0, "Concentration(#/cc)"=[]} {"ExtinctionOrAbsorptionOrScattering" scale=0.0..2.0}
  in  "Retrieve RI without taking the mean (MC)":bool
  out "Loop index (MC) 2":i32=4
  in  "Retrieve RI Calculate lines seperately":bool
  out "MC progress":u8(slide)=5 max=5 scale=-1.0..5.0
  in  "Save RI MC":bool
  out "Saved RI (MC) to this filename and path":path=path "Z:/Dropbox/Lior Segev/Lior Segev Projects/RI retrieval in Labview/Data/SyntheticData/SRFA_Spectrafit1-RI-MC-result.xls"
  out "Saved RI to this filename and path":path=path "Z:/Dropbox/Lior Segev/Lior Segev Projects/RI retrieval in Labview/Data/SyntheticData/PahokeeSynthetic/data/PahokeeFake4nd-ApproxError-Error-Restricted_RIresult.txt"
  out "Time Left (min) (MC)":dbl=0.0242 format="%#.1f"
  out "Loop index (MC)":i32=4
  out "Imaginary Part MC":cluster{dbl[], dbl[]}[](graph)=[{[414.59], [0.0008685207556328173]}, {[414.59, 414.59, 414.59], [nan, 0.004360832212642005, -0.0026237907013763706]}]
  out "Real Part MC":cluster{dbl[], dbl[]}[](graph)=[{[414.59], [1.5002369861550031]}, {[414.59, 414.59, 414.59], [nan, 1.5023737313826764, 1.4981002409273299]}]
  in  "Size of statistics":i32=5 min=0 max=150 step=1
  in  "Retrieve RI (MC)":bool
  out "Not Corrected for Multiple charge Best fit result":T3(graph)=[{"Ramp Pattern"=[1.3608384019262716, 1.5707963267948966, 1.7496493739052066, 1.9440548598946739, 2.169565223642456, 2.3328658318736086, 2.50394265954434, 2.6905719260942287, 2.8927536315232745, 3.1104877758314786, 3.3359981395792606, 3.584837161645779, 3.8570048420310328], "Extinction"=[6.178792893996032e-11, 1.0360347996174468e-10, 1.4599048359098532e-10, 1.894070733587938e-10, 2.6375374106990535e-10, 3.3972105684121345e-10, 4.3435802177249627e-10, 5.178882878098534e-10, 6.3749344691999e-10, 7.915454958151713e-10, 9.785475763024465e-10, 1.1461003257551283e-09, 1.3954254418635514e-09]}, {"Ramp Pattern"=[1.3608384019262716, 1.3608384019262716, 1.3608384019262716, 1.5707963267948966, 1.5707963267948966, 1.5707963267948966, 1.7496493739052066, 1.7496493739052066, 1.7496493739052066, 1.9440548598946739, 1.9440548598946739, 1.9440548598946739, 2.169565223642456, 2.169565223642456, 2.169565223642456, 2.3328658318736086, 2.3328658318736086, 2.3328658318736086, 2.50394265954434, 2.50394265954434, 2.50394265954434, 2.6905719260942287, 2.6905719260942287, 2.6905719260942287, 2.8927536315232745, 2.8927536315232745, 2.8927536315232745, 3.1104877758314786, 3.1104877758314786, 3.1104877758314786, 3.3359981395792606, 3.3359981395792606, 3.3359981395792606, 3.584837161645779, 3.584837161645779, 3.584837161645779, 3.8570048420310328, 3.8570048420310328, 3.8570048420310328], "Extinction"=[nan, 6.293687777456518e-11, 6.063898010535546e-11, nan, 1.0606455712917593e-10, 1.0114240279431343e-10, nan, 1.506172511115714e-10, 1.4136371607039924e-10, nan, 1.985386087052616e-10, 1.8027553801232602e-10, nan, 2.6748789046088486e-10, 2.6001959167892583e-10, nan, 3.4511045419894767e-10, 3.3433165948347924e-10, nan, 4.4340909069404093e-10, 4.253069528509516e-10, nan, 5.318265237328016e-10, 5.039500518869052e-10, nan, 6.413979300954665e-10, 6.335889637445135e-10, nan, 7.976294358197287e-10, 7.854615558106139e-10, nan, 9.88139280555883e-10, 9.6895587204901e-10, nan, 1.1627558304105662e-09, 1.1294448210996905e-09, nan, 1.4199918671188528e-09, 1.37085901660825e-09]}, {"Ramp Pattern"=[1.3608384019262716, 1.5707963267948966, 1.7496493739052066, 1.9440548598946739, 2.169565223642456, 2.3328658318736086, 2.50394265954434, 2.6905719260942287, 2.8927536315232745, 3.1104877758314786, 3.3359981395792606, 3.584837161645779, 3.8570048420310328], "Extinction"=[6.178792561956062e-11, 1.0360347900399653e-10, 1.4599047798203778e-10, 1.8940707759756924e-10, 2.637537530154407e-10, 3.397210621054649e-10, 4.3435802156538446e-10, 5.178883010654784e-10, 6.374934275556076e-10, 7.915454988899862e-10, 9.785475494436064e-10, 1.1461002853002994e-09, 1.395425458367e-09]}]
  out "Normalized Residuals vs Size parameter":T4(graph)=[{"Size parameters"=[1.3608384019262716, 1.5707963267948966, 1.7496493739052066, 1.9440548598946739, 2.169565223642456, 2.3328658318736086, 2.50394265954434, 2.6905719260942287, 2.8927536315232745, 3.1104877758314786, 3.3359981395792606, 3.584837161645779, 3.8570048420310328], "Normalized Residuals"=[0.11611698626140751, -0.00782281527933284, -0.39724759167122026, -0.05829577642327765, 0.5102944282210912]}]
  out "Imaginary Part vs wavelength":cluster{dbl[], dbl[]}[](graph)=[{[404.0], [0.047890347587708715]}, {[404.0, 404.0, 404.0], [nan, 0.05101534758770872, 0.04476534758770871]}, {[], []}]
  out "Real Part vs wavelength":cluster{dbl[], dbl[]}[](graph)=[{[404.0], [1.6120396036585403]}, {[404.0, 404.0, 404.0], [nan, 1.6292271036585402, 1.5948521036585404]}, {[], []}]
  in  "OK":bool
  # "Finding Factors is performed on only a single wavelength"
  # "n"
  # "k"
  # "Developed by Lior Segev\nsegev.lior@gmail.com\nYinon Rudich's Group\nDepartment of Earth and Planetary Sciences\n09 Dec 2013\nVer 1.0"
  # "Factors that minimize \nthe residue"
  # "Extinction Factor"
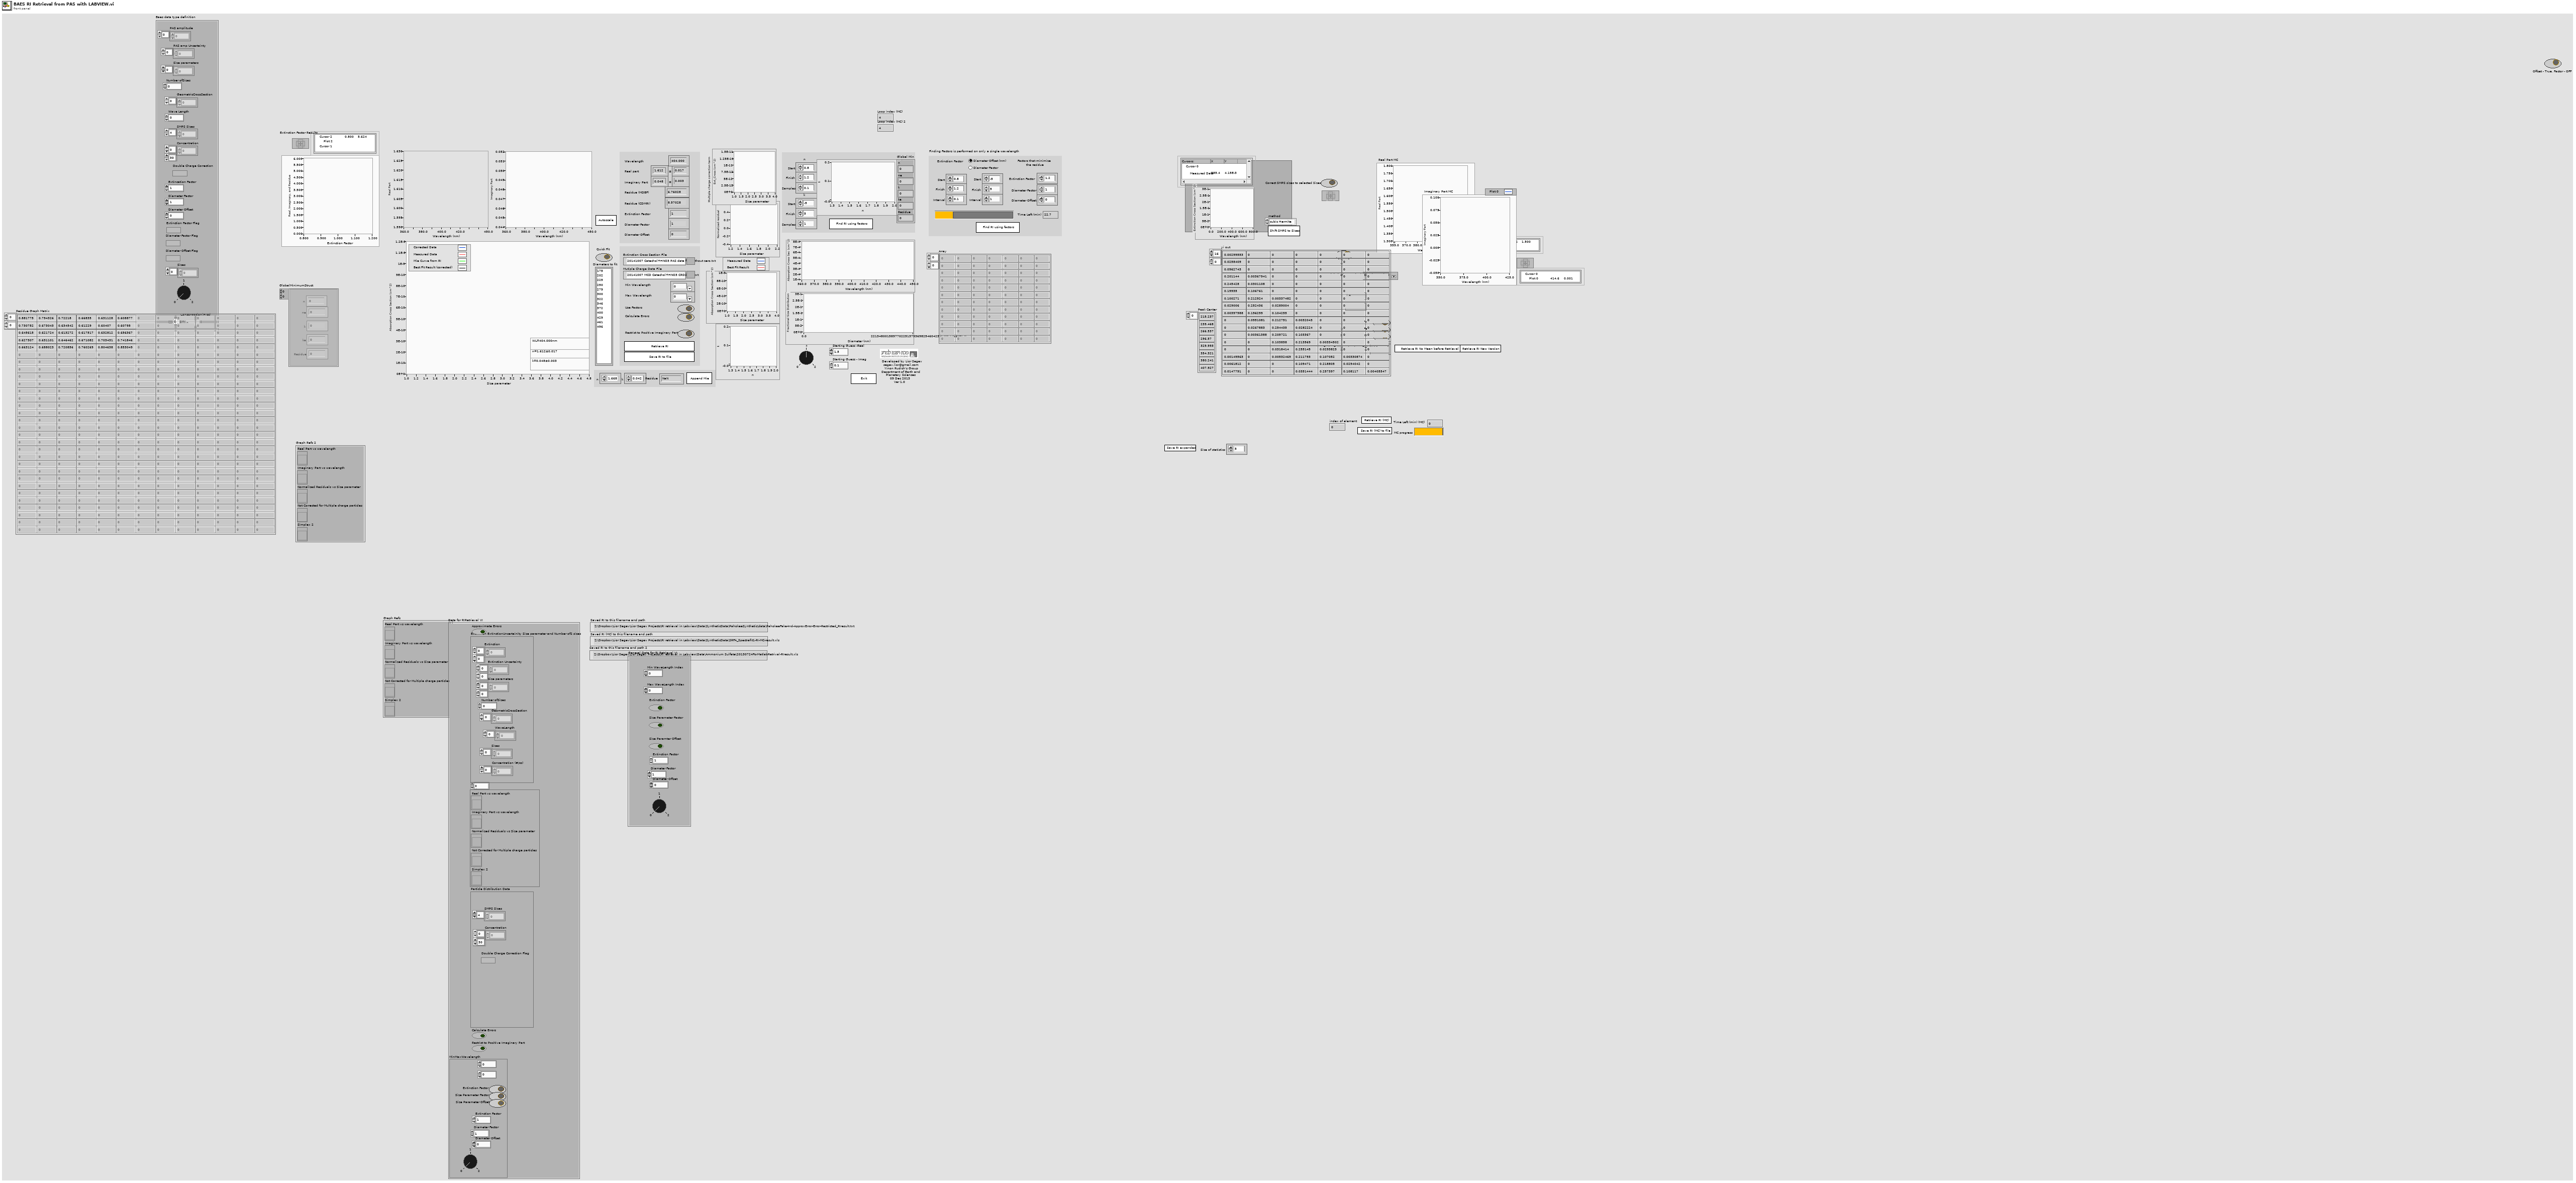
[diagram p1: front panel]
types:
  T1 = cluster{"n":dbl, "ne":dbl, "k":dbl, "ke":dbl, "Residue":dbl}
  T2 = cluster{"n":dbl, "ne":dbl, "k":dbl, "ke":dbl, "Residue":dbl}[][]
  T3 = cluster{"Ramp Pattern":dbl[], "Extinction":dbl[]}[]
  T4 = cluster{"Size parameters":dbl[], "Normalized Residuals":dbl[]}[]
  T5 = typedef "GeneralDataForRIRetrieval.ctl" = cluster{"Min WaveLength Index":u16, "Max WaveLength Index":u16, "Extinction Factor":bool, "Size Parameter Factor":bool, "Size Paramter Offset":bool, "Extinction Factor":dbl, "Diameter Factor":dbl, "Diameter Offset":dbl, "ExtinctionOrAbsorptionOrScattering":i8}
  T6 = cluster{"Real Part vs wavelength":refnum<vi>, "Imaginary Part vs wavelength":refnum<vi>, "Normalized Residuals vs Size parameter":refnum<vi>, "Not Corrected for Multiple charge particles":refnum<vi>, "Simplex 2":refnum<vi>}
  T7 = typedef "ReadBaesDataTypeDefinition.ctl" = cluster{"Extinction":dbl[][], "Extinction Uncertainty":dbl[][], "Size parameters":dbl[][], "Number ofSizes":dbl, "GeometricCrossSection":dbl[], "WaveLength":dbl[], "Sizes":dbl[], "Concentration (#/cc)":dbl[]}
  T8 = typedef "ParticleDistributionData.ctl" = cluster{"SMPS Sizes":dbl[], "Concentration":dbl[][], "Double Charge Correction Flag":bool}
  T9 = cluster{"Approximate Errors":bool, "Extinction ExtinctionUncertainity Size parameter and Number ofS sizes":T7, "Minimization method":u16, "Graph Ref":cluster{"Real Part vs wavelength":refnum<vi>, "Imaginary Part vs wavelength":refnum<vi>, "Normalized Residuals vs Size parameter":refnum<vi>, "Not Corrected for Multiple charge particles":refnum<vi>, "Simplex 2":refnum<vi>}, "Particle Distribution Data":T8, "Calculate Errors":bool, "Restrict to Positive Imaginary Part":bool, "MinMaxWavelength":cluster{i32, i32, "Extinction Factor":bool, "Size Parameter Factor":bool, "Size Parameter Offset":bool, "Extinction Factor":dbl, "Diameter Factor":dbl, "Diameter Offset":dbl, "ExtinctionOrAbsorptionOrScattering":i8}}
  T10 = typedef "BaesDataTypeDefinition.ctl" = cluster{"PAS amplitude":dbl[], "PAS amp Uncertainty":dbl[], "Size parameters":dbl[], "Number ofSizes":dbl, "GeometricCrossSection":dbl[], "Wave Length":dbl, "SMPS Sizes":dbl[], "Concentration":dbl[][], "Double Charge Correction":bool, "Extincation Factor":dbl, "Diameter Factor":dbl, "Diameter Offset":dbl, "Extinction Factor Flag":bool, "Diameter Factor Flag":bool, "Diameter Offset Flag":bool, "Sizes":dbl[], "ExtinctionOrAbsorptionOrScattering":i8, "Concentration(#/cc)":dbl[]}
  T11 = enum32{"invalid app kind", "Development System", "Run Time System", "Student Edition", "Embedded LabVIEW", "Evaluation", "Custom"}
  T12 = enum32{"Invalid", "Standard", "Closed", "Hidden", "Minimized", "Maximized"}
  T13 = cluster{"SMPS Sizes":dbl[], "Concentration":dbl[]}[]
  T14 = typedef "NI_Gmath.lvlib/stopping criteria.ctl" = cluster{"function tolerance":dbl, "parameter tolerance":dbl, "max iterations":i32, "max function calls":i32, "gradient tolerance":dbl, "max time (sec)":dbl}
  T15 = typedef "LVPoint32TypeDef.ctl" = cluster{"Horizontal":i32, "Vertical":i32}
  T16 = typedef "RIandRIMCResults.ctl" = cluster{"Real RI":dbl[], "Imaginary RI":dbl[], "Std Imaginary RI":dbl[], "Std Real RI":dbl[], "Wavelength":dbl[], "Residue":dbl[], "Extinction Factor":dbl[], "Diameter Factor":dbl[], "Diameter Offset":dbl[], "Best fit result":dbl[][], "Normalized Residuals":dbl[][]}
  T17 = cluster{"Core":cluster{"Current VI Reference":refnum<vi>, "Close Panel on Exit?":bool}, "Extinction ExtinctionUncertainity Size parameter and Number ofS sizes":T7, "Particle Distribution Data":T8, "RI results":T16, "RI MC results":T16, "Extinction Cross section Path":path, "Multiple charge correction file Path":path, "FullExtinctionData":dbl[][], "NumberOfMeasurementsperSize":i32, "Baes data type definition":T10}
  T18 = cluster{"Current VI Reference":refnum<vi>, "Close Panel on Exit?":bool}
  T19 = cluster{"WaveLengths":dbl[], "Extinction":dbl[]}[]
  T20 = cluster{"SMPS Sizes":dbl[], "Concentration":dbl[]}
  T21 = cluster{"\nSMPS sizes":dbl[], "Shifted Concentration":dbl[]}
  T22 = cluster{"Size parameters":dbl[], "Extinction Crosssections":dbl[]}
  T23 = cluster{"Size parameters":dbl[], "Extinction Crosssections":dbl[]}[]
  T24 = cluster{"Real Part vs wavelength":refnum<vi>, "Imaginary Part vs wavelength":refnum<vi>, "Normalized Residuals vs Size parameter":refnum<vi>, "Not Corrected for Multiple charge Best fit result":refnum<vi>, "Simplex":refnum<vi>}
  T25 = typedef "NI_Matrix.lvlib/RealMatrix.ctl" = dbl[][]
  T26 = cluster{"Size parameters":dbl[], "Expected Extinction/Absorption Cross Section":dbl[]}
  T27 = cluster{"Size parameters":dbl[], "Normalized Residuals":dbl[]}
  T28 = cluster{"Size parameters":dbl[], "Best fit result":dbl[]}
  T29 = cluster{"Size parameters":dbl[], "Best fit result":dbl[]}[]
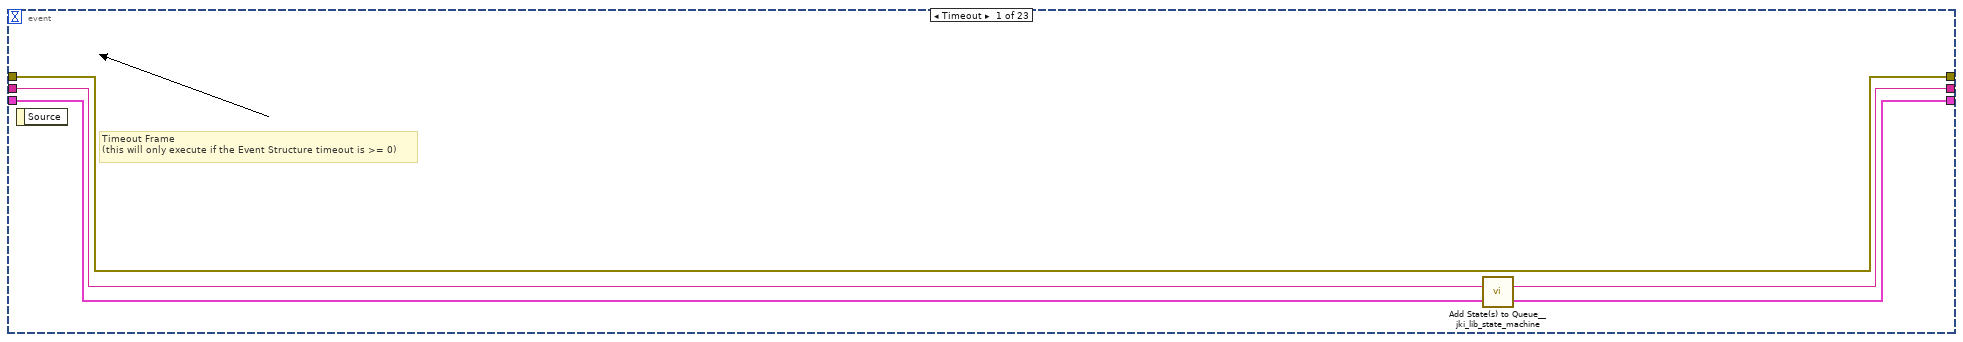
[diagram p3: hidden frame]
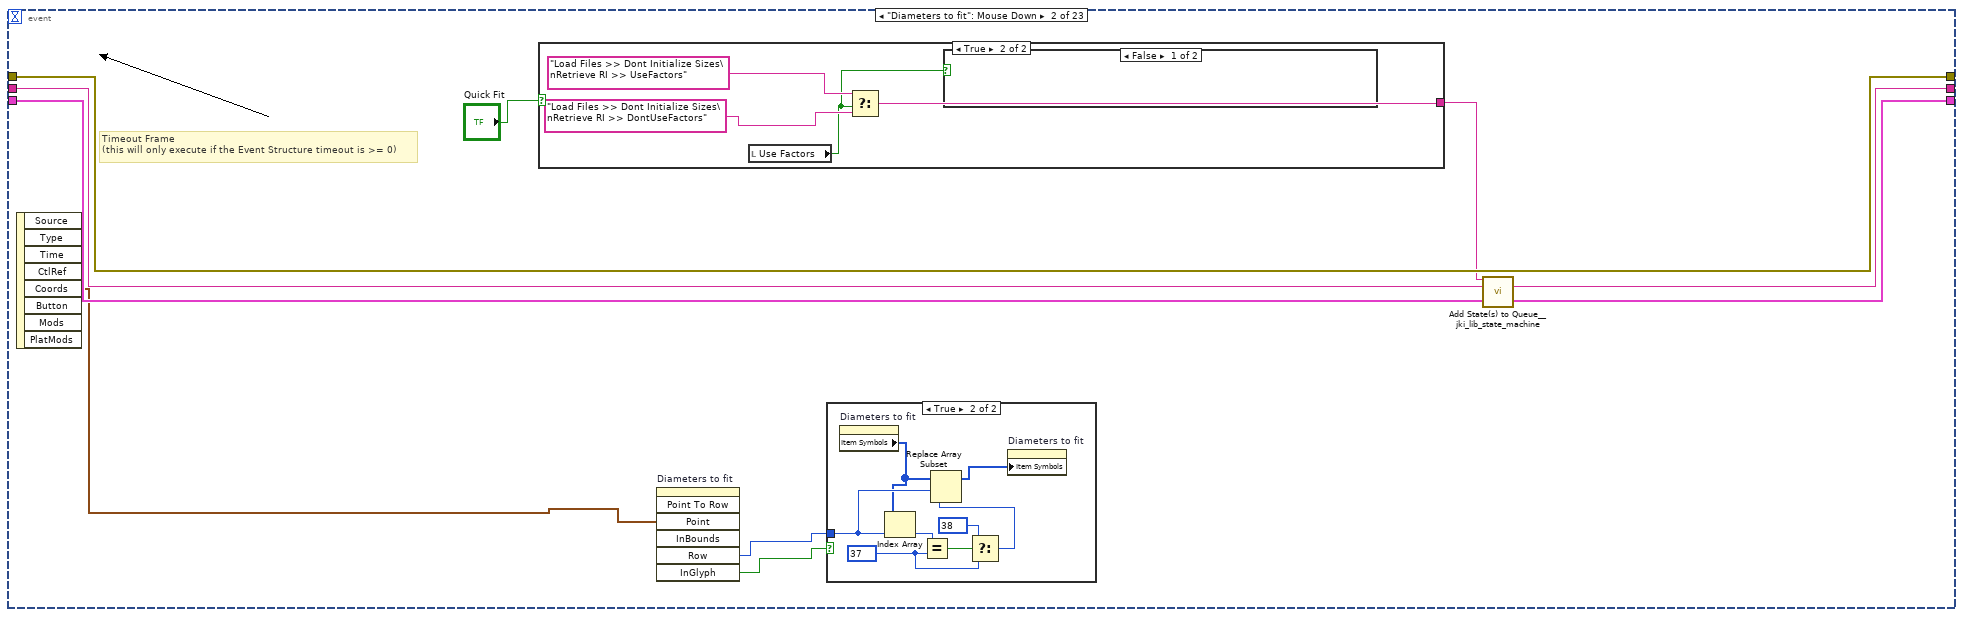
[diagram p4: hidden frame]
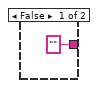
[diagram p5: hidden frame]
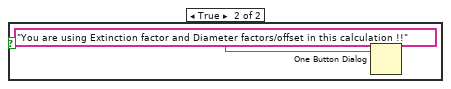
[diagram p6: hidden frame]
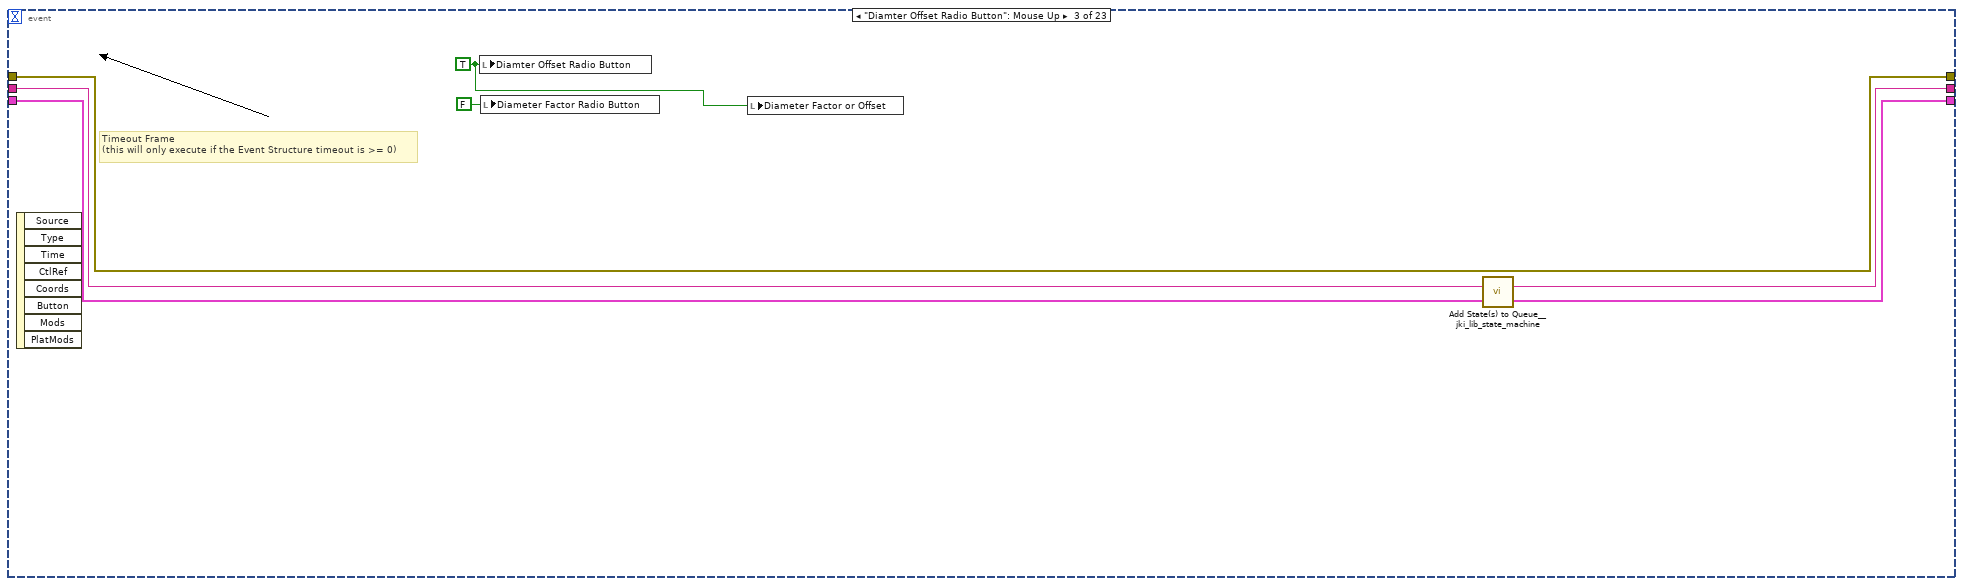
[diagram p8: hidden frame]
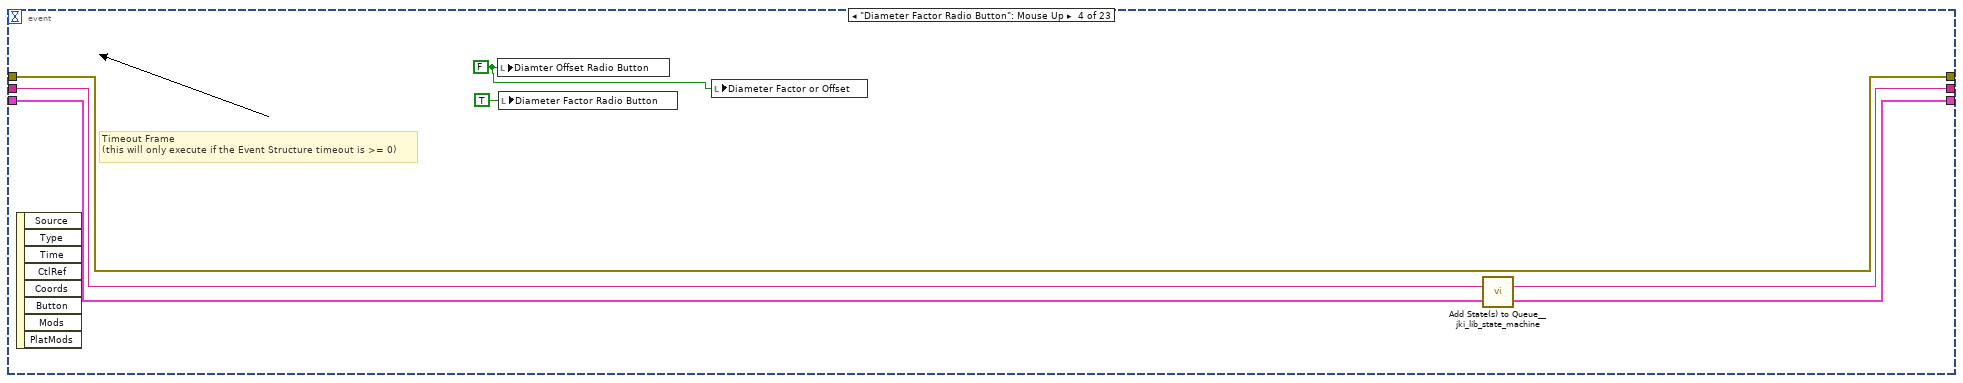
[diagram p9: hidden frame]
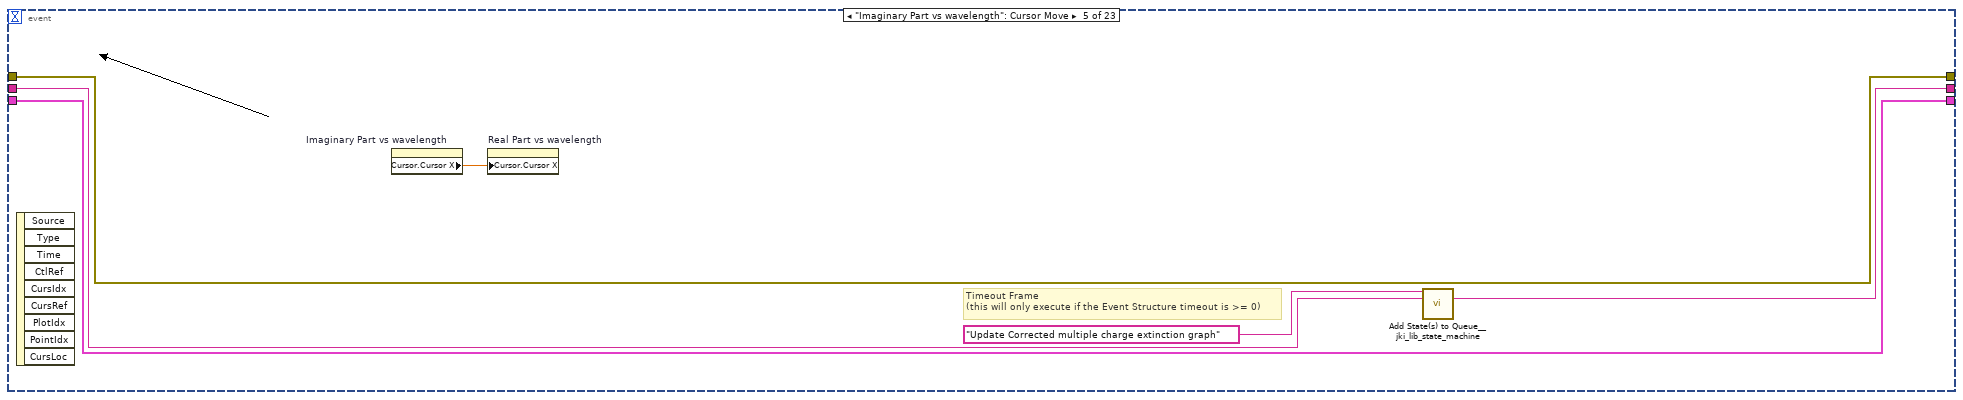
[diagram p10: hidden frame]
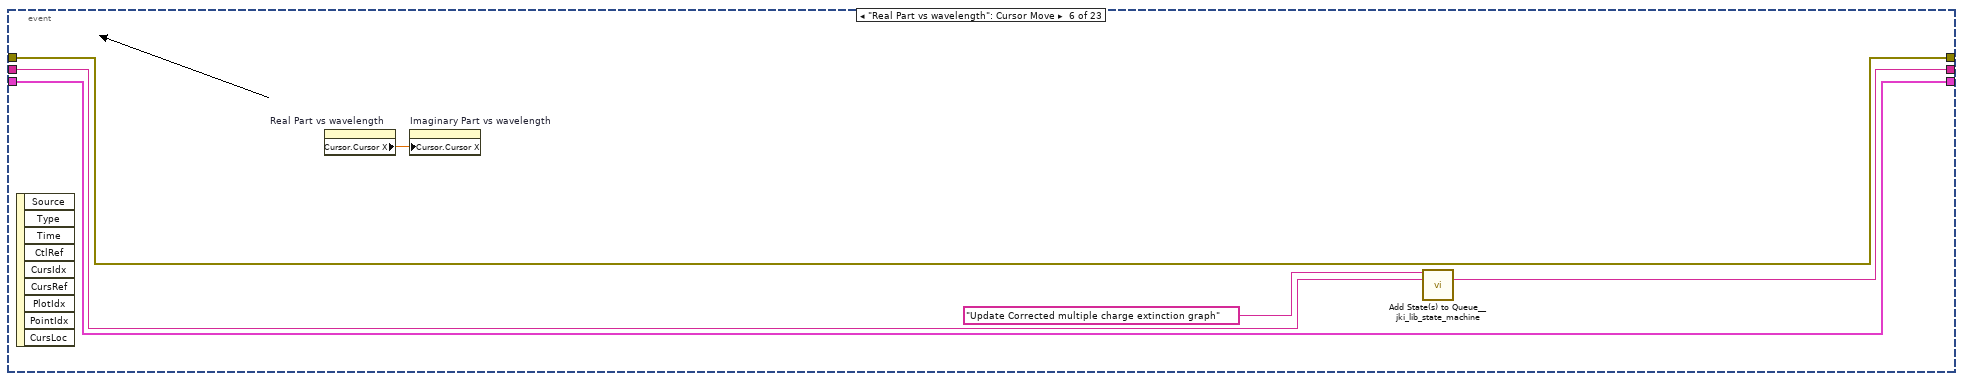
[diagram p11: hidden frame]
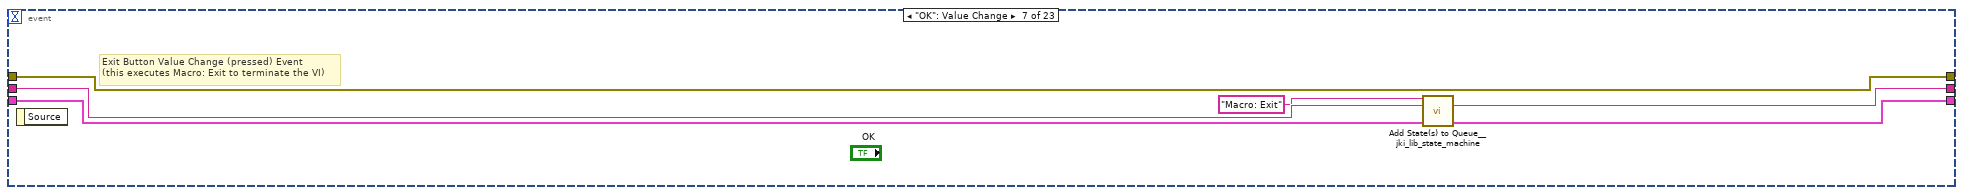
[diagram p12: hidden frame]
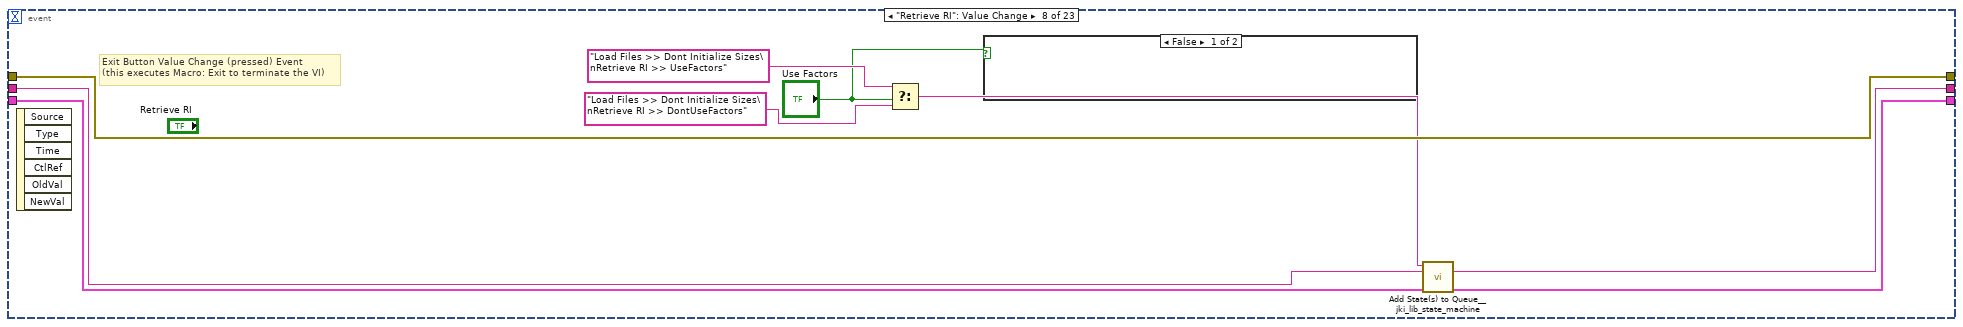
[diagram p13: hidden frame]
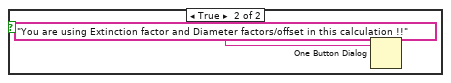
[diagram p14: hidden frame]
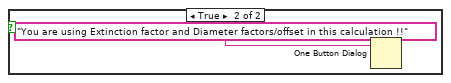
[diagram p15: hidden frame]
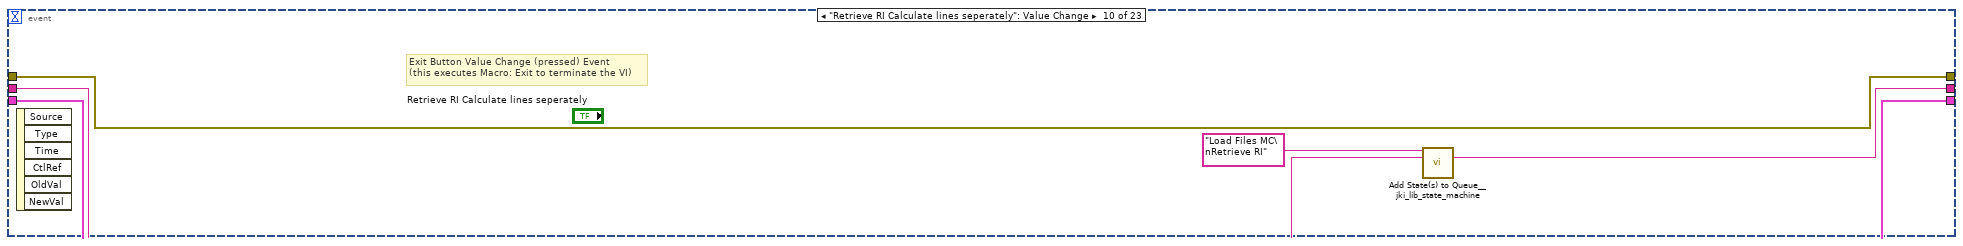
[diagram p16: hidden frame]
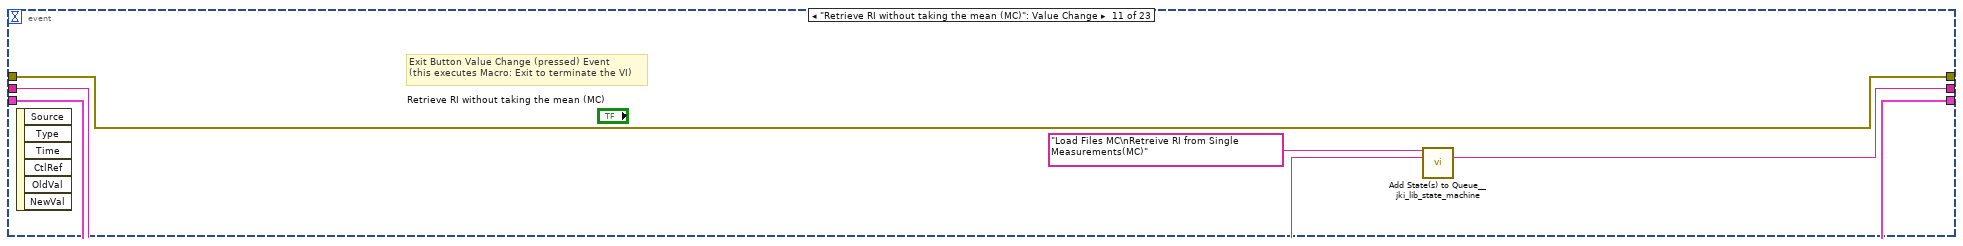
[diagram p17: hidden frame]
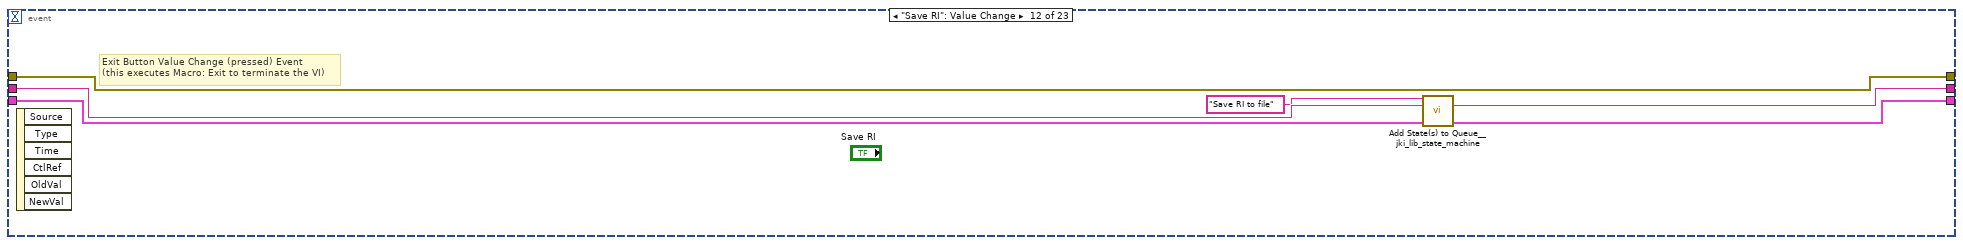
[diagram p18: hidden frame]
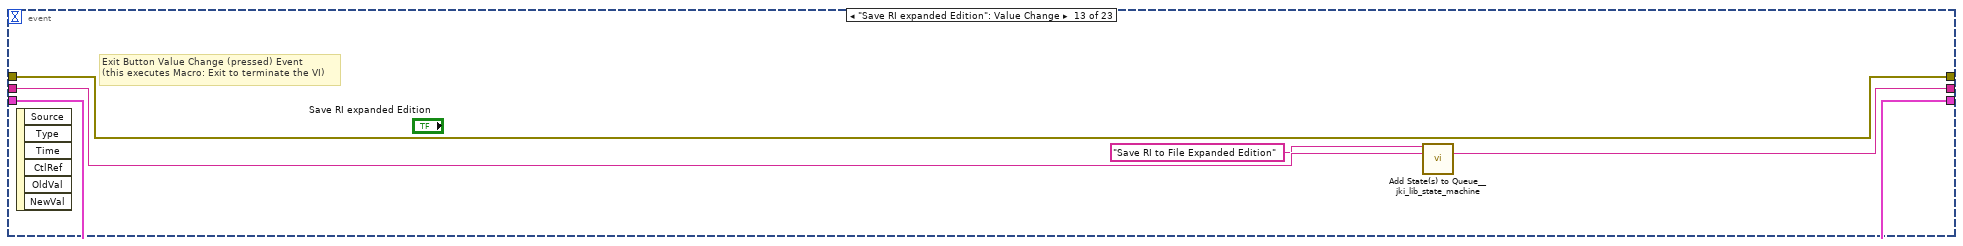
[diagram p19: hidden frame]
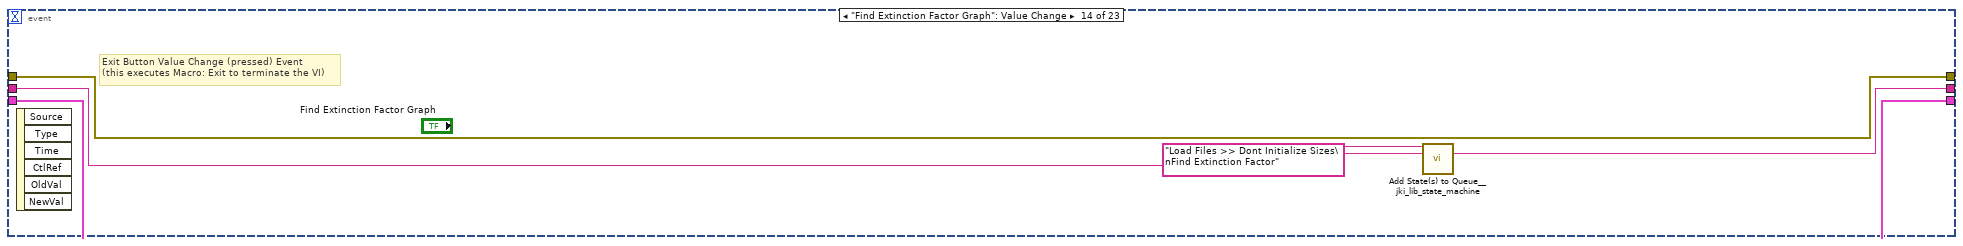
[diagram p20: hidden frame]
diagram:
  (unwired) cluster{dbl[], dbl[]}[] [{[353.79999, 354.37, 354.94, 355.51001, 356.07999, 356.64999, 357.22, 357.78, 358.35001, 358.91, 359.47, 360.03, 360.59, 361.14999, 361.70001, 362.26001, 362.81, 363.35999, 363.91, 364.45999, 365.01001, 365.56, 366.10001, 366.64999, 367.19, 367.73001, 368.26999, 368.81, 369.35001, 369.89001, 370.42001, 370.95999, 371.48999, 372.03, 372.56, 373.09, 373.62, 374.14999, 374.67999, 375.20999, 375.73001, 376.26001, 376.78, 377.31, 377.82999, 378.35001, 378.87, 379.39001, 379.91, 380.42999, 380.95001, 381.47, 381.98001, 382.5, 383.01001, 383.53, 384.04001, 384.54999, 385.07001, 385.57999, 386.09, 386.60001, 387.10999, 387.62, 388.13, 388.63, 389.14001, 389.64999, 390.14999, 388.63, 389.14001, 389.64999, 390.14999, 390.66, 391.16, 391.67001, 392.17001, 392.67999, 393.17999, 393.67999, 394.17999, 394.67999, 395.19, 395.69, 396.19, 396.69, 397.19, 397.69, 398.19, 398.69, 399.19, 399.67999, 400.17999, 400.67999, 401.17999, 401.67999, 402.17001, 402.67001, 403.17001, 403.66, 404.16, 404.66, 405.14999, 405.64999, 406.14999, 406.64001, 407.14001, 407.64001, 408.13, 408.63, 409.13, 409.62, 410.12, 410.62, 411.10999, 411.60999, 412.10001, 412.60001, 413.10001, 413.60001, 414.09, 414.59, 415.09, 415.59, 416.07999, 416.57999, 417.07999, 417.57999, 418.07999, 418.57999], [-0.006880589406937364, -0.005591015240643177, -0.0008128900086740067, 0.0059132125129690355, 0.004727233671001155, 0.005285323022981176, 0.012079702376504426, 0.013295932917972094, 0.009723681324539938, 0.01340675951578305, 0.014300736755976685, 0.017412400216708195, 0.016082847953221062, 0.019541949361009746, 0.016681812204333245, 0.021839119627984467, 0.01917857630542129, 0.01659316249089897, 0.017920546232635386, 0.02331211752971285, 0.018736628440528875, 0.02278859303667559, 0.020160162589600072, 0.01944517701034782, 0.01722059774576336, 0.014545686876081154, 0.017064244530774875, 0.014871257634513302, 0.015814167710632307, 0.012323804928601011, 0.017001137568295226, 0.01761462364709586, 0.011094176200131175, 0.013484050217230092, 0.015463713328499572, 0.017445979654003158, 0.017890194826904918, 0.012171772373985729, 0.0090971027467458, 0.010861800449201833, 0.009486644105636509, 0.009660218265489668, 0.011543706295196892, 0.009241826302022669, 0.0043825353242573275, 0.006012733183160885, 0.016684276899031823, 0.004574877464619924, 0.004680287507653695, 0.005436664247245053, 0.005769621008366801, 0.007016844481986471, 0.005292591657780566, 0.0023362286578048827, 0.001404106784902966, 0.006018627453886426, 0.005868676603131451, 0.004574542292684771, 0.00013407550315604303, 0.005111191491887428, 0.006244050999230227, 0.008470422941900313, 0.0019502929036388976, 0.00693045579799217, 0.00729891092487377, 0.006591697414114595, -0.00464719874347794, -0.0028833235584898023, 0.0030601034901337606, -0.019172722466464624, 0.00349415319418767, -0.019612863241454764, 0.006230360324734642, -0.007644525136092856, -0.0024464061374237676, -0.015743142364772214, -0.01362771525815333, 0.0023827303007783484, 0.004434076127836306, 0.0015447059453072153, -0.0012530544220862782, 0.013970670419985256, 0.005734164261953947, 0.008763635301725982, 0.006956973905904259, 0.0058963200240359104, 0.004165371933482626, 0.009600835719607804, 0.0037134970421865933, 0.01607998543651406, 0.007081749858913052, 0.014576117182728877, 0.010330077196118458, 0.013431346724388227, 0.009247446675431951, 0.013068538923394903, 0.009279456157815679, 0.013932752616816237, 0.013225407198184207, 0.014934507206195071, 0.017106424708032086, 0.01564773346122451, 0.017710188001506998, 0.011882676676028447, 0.014042275741809086, 0.014230648119115306, 0.011795090172377915, 0.01414643231400618, 0.01678394258342081, 0.006007592633110041, 0.012137073369673021, 0.015868997327494014, 0.008004974625515329, 0.012176508619891986, 0.011391254549822344, 0.01562344561258754, 0.005349593450524416, 0.012534566898108031, 0.015731735948216675, 0.012454435731493445, 0.016355219901748506, 0.007853560039517043, 0.0044201289692190875, 0.009950585420452563, 0.0011992242078176175, -0.0040610702724316675, 0.005166605821146673, 0.00788498225462348, -0.004714349788695529, 0.007145714404910847]}, ...(3 in all)] ("Imaginary Part vs wavelength")
  (unwired) cluster{dbl[], dbl[]}[] [{[353.79999, 354.37, 354.94, 355.51001, 356.07999, 356.64999, 357.22, 357.78, 358.35001, 358.91, 359.47, 360.03, 360.59, 361.14999, 361.70001, 362.26001, 362.81, 363.35999, 363.91, 364.45999, 365.01001, 365.56, 366.10001, 366.64999, 367.19, 367.73001, 368.26999, 368.81, 369.35001, 369.89001, 370.42001, 370.95999, 371.48999, 372.03, 372.56, 373.09, 373.62, 374.14999, 374.67999, 375.20999, 375.73001, 376.26001, 376.78, 377.31, 377.82999, 378.35001, 378.87, 379.39001, 379.91, 380.42999, 380.95001, 381.47, 381.98001, 382.5, 383.01001, 383.53, 384.04001, 384.54999, 385.07001, 385.57999, 386.09, 386.60001, 387.10999, 387.62, 388.13, 388.63, 389.14001, 389.64999, 390.14999, 388.63, 389.14001, 389.64999, 390.14999, 390.66, 391.16, 391.67001, 392.17001, 392.67999, 393.17999, 393.67999, 394.17999, 394.67999, 395.19, 395.69, 396.19, 396.69, 397.19, 397.69, 398.19, 398.69, 399.19, 399.67999, 400.17999, 400.67999, 401.17999, 401.67999, 402.17001, 402.67001, 403.17001, 403.66, 404.16, 404.66, 405.14999, 405.64999, 406.14999, 406.64001, 407.14001, 407.64001, 408.13, 408.63, 409.13, 409.62, 410.12, 410.62, 411.10999, 411.60999, 412.10001, 412.60001, 413.10001, 413.60001, 414.09, 414.59, 415.09, 415.59, 416.07999, 416.57999, 417.07999, 417.57999, 418.07999, 418.57999], [1.6483722836524246, 1.6546363395359365, 1.647298907653894, 1.6533287796168583, 1.6513909602141936, 1.6441728100483295, 1.6485630092327472, 1.6465913680498476, 1.644326968253007, 1.6458723273169005, 1.6423749873362237, 1.6435071871004756, 1.6412154858600103, 1.6396834087598822, 1.6391132715105765, 1.6382846511661762, 1.6358307684719318, 1.6354408519662669, 1.6334428509272396, 1.6328074965992703, 1.630211530333035, 1.629597879928187, 1.6276773015694914, 1.6248549924331006, 1.6221911228582016, 1.619860370624227, 1.6186660879658288, 1.6177483954461045, 1.618059125989092, 1.616294733806861, 1.6164932554209357, 1.6163255198620012, 1.615138021497404, 1.6164105257665495, 1.617235077199874, 1.6147912416880703, 1.6164196882297972, 1.6150368907017385, 1.6144850551191468, 1.6133228562399728, 1.6128153905854543, 1.6139403869979996, 1.6131967111234533, 1.6143159173824806, 1.6121220874076225, 1.6114366661699004, 1.6094507790415067, 1.6108839833096118, 1.6122492163476982, 1.6122322997299472, 1.6077321043459216, 1.6138723793940135, 1.6118005408009028, 1.6157486465235684, 1.6147077896853421, 1.6142964675684908, 1.614804272990439, 1.6117647309822476, 1.6161328124848642, 1.6101356911507883, 1.612094662439775, 1.6118531546799915, 1.614236269971587, 1.6062328837497617, 1.6105586500151539, 1.6108228692284308, 1.6178782024106462, 1.6087987962691102, 1.6074587087659151, 1.6187364188290658, 1.6209092605148896, 1.6151493452793495, 1.6182798966697, 1.6109338276299237, 1.6085077651242317, 1.613655399235577, 1.612511934789509, 1.607851046633587, 1.6057532268507935, 1.6024870719133475, 1.6038884748636346, 1.605523559015856, 1.5960101592112506, 1.5997312604952778, 1.598377877440321, 1.597392154092918, 1.600589807386528, 1.5995684913350448, 1.5979434008328421, 1.5961998900762004, 1.5970150338732805, 1.5939307380342091, 1.596156816544494, 1.5962182334684933, 1.597512896681686, 1.595101996088882, 1.5933960300930927, 1.592688229676817, 1.5913322143224218, 1.5917530088094214, 1.591614538502429, 1.5914637114820218, 1.5878221602705458, 1.5928834293750267, 1.5915729711917386, 1.587309104722474, 1.5918112038963161, 1.5881066262119135, 1.584965267353939, 1.5914289179893895, 1.586911737372422, 1.581731065142223, 1.5886590769172397, 1.5849680475176062, 1.586099454232746, 1.581195601241917, 1.5854707251659343, 1.5865012245981702, 1.5838978086861526, 1.584800751487047, 1.5848505559733816, 1.5857486239152707, 1.585591816537336, 1.5810404634087085, 1.5851743649291072, 1.5859104770394237, 1.5823664432736304, 1.5792071958230995, 1.590530467368216, 1.5870072549949592]}, {[353.79999, 353.79999, 353.79999, 354.37, 354.37, 354.37, 354.94, 354.94, 354.94, 355.51001, 355.51001, 355.51001, 356.07999, 356.07999, 356.07999, 356.64999, 356.64999, 356.64999, 357.22, 357.22, 357.22, 357.78, 357.78, 357.78, 358.35001, 358.35001, 358.35001, 358.91, 358.91, 358.91, 359.47, 359.47, 359.47, 360.03, 360.03, 360.03, 360.59, 360.59, 360.59, 361.14999, 361.14999, 361.14999, 361.70001, 361.70001, 361.70001, 362.26001, 362.26001, 362.26001, 362.81, 362.81, 362.81, 363.35999, 363.35999, 363.35999, 363.91, 363.91, 363.91, 364.45999, 364.45999, 364.45999, 365.01001, 365.01001, 365.01001, 365.56, 365.56, 365.56, 366.10001, 366.10001, 366.10001, 366.64999, 366.64999, 366.64999, 367.19, 367.19, 367.19, 367.73001, 367.73001, 367.73001, 368.26999, 368.26999, 368.26999, 368.81, 368.81, 368.81, 369.35001, 369.35001, 369.35001, 369.89001, 369.89001, 369.89001, 370.42001, 370.42001, 370.42001, 370.95999, 370.95999, 370.95999, 371.48999, 371.48999, 371.48999, 372.03, 372.03, 372.03, 372.56, 372.56, 372.56, 373.09, 373.09, 373.09, 373.62, 373.62, 373.62, 374.14999, 374.14999, 374.14999, 374.67999, 374.67999, 374.67999, 375.20999, 375.20999, 375.20999, 375.73001, 375.73001, 375.73001, 376.26001, 376.26001, 376.26001, 376.78, 376.78, 376.78, 377.31, 377.31, 377.31, 377.82999, 377.82999, 377.82999, 378.35001, 378.35001, 378.35001, 378.87, 378.87, 378.87, 379.39001, 379.39001, 379.39001, 379.91, 379.91, 379.91, 380.42999, 380.42999, 380.42999, 380.95001, 380.95001, 380.95001, 381.47, 381.47, 381.47, 381.98001, 381.98001, 381.98001, 382.5, 382.5, 382.5, 383.01001, 383.01001, 383.01001, 383.53, 383.53, 383.53, 384.04001, 384.04001, 384.04001, 384.54999, 384.54999, 384.54999, 385.07001, 385.07001, 385.07001, 385.57999, 385.57999, 385.57999, 386.09, 386.09, 386.09, 386.60001, 386.60001, 386.60001, 387.10999, 387.10999, 387.10999, 387.62, 387.62, 387.62, 388.13, 388.13, 388.13, 388.63, 388.63, 388.63, 389.14001, 389.14001, 389.14001, 389.64999, 389.64999, 389.64999, 390.14999, 390.14999, 390.14999, 388.63, 388.63, 388.63, 389.14001, 389.14001, 389.14001, 389.64999, 389.64999, 389.64999, 390.14999, 390.14999, 390.14999, 390.66, 390.66, 390.66, 391.16, 391.16, 391.16, 391.67001, 391.67001, 391.67001, 392.17001, 392.17001, 392.17001, 392.67999, 392.67999, 392.67999, 393.17999, 393.17999, 393.17999, 393.67999, 393.67999, 393.67999, 394.17999, 394.17999, 394.17999, 394.67999, 394.67999, 394.67999, 395.19, 395.19, 395.19, 395.69, 395.69, 395.69, 396.19, 396.19, 396.19, 396.69, 396.69, 396.69, 397.19, 397.19, 397.19, 397.69, 397.69, 397.69, 398.19, 398.19, 398.19, 398.69, 398.69, 398.69, 399.19, 399.19, 399.19, 399.67999, 399.67999, 399.67999, 400.17999, 400.17999, 400.17999, 400.67999, 400.67999, 400.67999, 401.17999, 401.17999, 401.17999, 401.67999, 401.67999, 401.67999, 402.17001, 402.17001, 402.17001, 402.67001, 402.67001, 402.67001, 403.17001, 403.17001, 403.17001, 403.66, 403.66, 403.66, 404.16, 404.16, 404.16, 404.66, 404.66, 404.66, 405.14999, 405.14999, 405.14999, 405.64999, 405.64999, 405.64999, 406.14999, 406.14999, 406.14999, 406.64001, 406.64001, 406.64001, 407.14001, 407.14001, 407.14001, 407.64001, 407.64001, 407.64001, 408.13, 408.13, 408.13, 408.63, 408.63, 408.63, 409.13, 409.13, 409.13, 409.62, 409.62, 409.62, 410.12, 410.12, 410.12, 410.62, 410.62, 410.62, 411.10999, 411.10999, 411.10999, 411.60999, 411.60999, 411.60999, 412.10001, 412.10001, 412.10001, 412.60001, 412.60001, 412.60001, 413.10001, 413.10001, 413.10001, 413.60001, 413.60001, 413.60001, 414.09, 414.09, 414.09, 414.59, 414.59, 414.59, 415.09, 415.09, 415.09, 415.59, 415.59, 415.59, 416.07999, 416.07999, 416.07999, 416.57999, 416.57999, 416.57999, 417.07999, 417.07999, 417.07999, 417.57999, 417.57999, 417.57999, 418.07999, 418.07999, 418.07999, 418.57999, 418.57999, 418.57999], [nan, 1.6563722836524246, 1.6403722836524246, nan, 1.6616363395359364, 1.6476363395359366, nan, 1.6542989076538939, 1.640298907653894, nan, 1.6603287796168582, 1.6463287796168584, nan, 1.6573909602141936, 1.6453909602141936, nan, 1.6501728100483295, 1.6381728100483295, nan, 1.6535630092327471, 1.6435630092327473, nan, 1.6515913680498475, 1.6415913680498477, nan, 1.649326968253007, 1.6393269682530072, nan, 1.6508723273169004, 1.6408723273169006, nan, 1.6473749873362236, 1.6373749873362238, nan, 1.6485071871004755, 1.6385071871004757, nan, 1.6462154858600102, 1.6362154858600104, nan, 1.6436834087598822, 1.6356834087598822, nan, 1.6431132715105765, 1.6351132715105765, nan, 1.6422846511661762, 1.6342846511661762, nan, 1.6398307684719318, 1.6318307684719318, nan, 1.6394408519662669, 1.6314408519662669, nan, 1.6374428509272396, 1.6294428509272396, nan, 1.6368074965992703, 1.6288074965992703, nan, 1.634211530333035, 1.626211530333035, nan, 1.633597879928187, 1.625597879928187, nan, 1.6316773015694914, 1.6236773015694914, nan, 1.6288549924331006, 1.6208549924331006, nan, 1.6261911228582016, 1.6181911228582015, nan, 1.623860370624227, 1.615860370624227, nan, 1.6226660879658288, 1.6146660879658288, nan, 1.6217483954461045, 1.6137483954461045, nan, 1.622059125989092, 1.614059125989092, nan, 1.620294733806861, 1.612294733806861, nan, 1.6204932554209357, 1.6124932554209357, nan, 1.6203255198620012, 1.6123255198620012, nan, 1.619138021497404, 1.611138021497404, nan, 1.6204105257665495, 1.6124105257665495, nan, 1.621235077199874, 1.613235077199874, nan, 1.6187912416880703, 1.6107912416880703, nan, 1.6204196882297972, 1.6124196882297972, nan, 1.6190368907017385, 1.6110368907017385, nan, 1.6184850551191468, 1.6104850551191467, nan, 1.6173228562399729, 1.6093228562399728, nan, 1.6168153905854543, 1.6088153905854543, nan, 1.6179403869979996, 1.6099403869979996, nan, 1.6171967111234533, 1.6091967111234533, nan, 1.6183159173824806, 1.6103159173824806, nan, 1.6161220874076225, 1.6081220874076225, nan, 1.6154366661699004, 1.6074366661699004, nan, 1.6134507790415067, 1.6054507790415067, nan, 1.6148839833096118, 1.6068839833096118, nan, 1.6172492163476981, 1.6072492163476984, nan, 1.617232299729947, 1.6072322997299473, nan, 1.6127321043459215, 1.6027321043459217, nan, 1.6188723793940134, 1.6088723793940136, nan, 1.6168005408009027, 1.606800540800903, nan, 1.6207486465235683, 1.6107486465235685, nan, 1.619707789685342, 1.6097077896853422, nan, 1.6192964675684907, 1.6092964675684909, nan, 1.619804272990439, 1.6098042729904392, nan, 1.6167647309822475, 1.6067647309822477, nan, 1.621132812484864, 1.6111328124848643, nan, 1.6161356911507883, 1.6041356911507882, nan, 1.618094662439775, 1.606094662439775, nan, 1.6178531546799915, 1.6058531546799915, nan, 1.620236269971587, 1.608236269971587, nan, 1.6122328837497617, 1.6002328837497617, nan, 1.6175586500151538, 1.603558650015154, nan, 1.6168228692284308, 1.6048228692284308, nan, 1.624878202410646, 1.6108782024106463, nan, 1.61579879626911, 1.6017987962691103, nan, 1.614458708765915, 1.6004587087659152, nan, 1.6347364188290658, 1.6027364188290658, nan, 1.6349092605148896, 1.6069092605148896, nan, 1.6281493452793494, 1.6021493452793496, nan, 1.6302798966697, 1.6062798966697, nan, 1.6219338276299236, 1.5999338276299238, nan, 1.6185077651242317, 1.5985077651242316, nan, 1.622655399235577, 1.6046553992355772, nan, 1.6215119347895088, 1.603511934789509, nan, 1.6168510466335868, 1.598851046633587, nan, 1.6137532268507935, 1.5977532268507935, nan, 1.6104870719133475, 1.5944870719133475, nan, 1.6108884748636345, 1.5968884748636347, nan, 1.613523559015856, 1.597523559015856, nan, 1.6030101592112505, 1.5890101592112507, nan, 1.6067312604952777, 1.592731260495278, nan, 1.605377877440321, 1.591377877440321, nan, 1.6043921540929178, 1.590392154092918, nan, 1.606589807386528, 1.594589807386528, nan, 1.6055684913350448, 1.5935684913350447, nan, 1.604943400832842, 1.5909434008328422, nan, 1.6031998900762003, 1.5891998900762005, nan, 1.6030150338732805, 1.5910150338732805, nan, 1.598930738034209, 1.5889307380342093, nan, 1.602156816544494, 1.590156816544494, nan, 1.6022182334684933, 1.5902182334684933, nan, 1.603512896681686, 1.591512896681686, nan, 1.601101996088882, 1.589101996088882, nan, 1.5993960300930927, 1.5873960300930927, nan, 1.598688229676817, 1.586688229676817, nan, 1.5963322143224217, 1.5863322143224219, nan, 1.5967530088094213, 1.5867530088094215, nan, 1.5966145385024288, 1.586614538502429, nan, 1.5964637114820217, 1.586463711482022, nan, 1.5928221602705457, 1.582822160270546, nan, 1.5978834293750266, 1.5878834293750268, nan, 1.5965729711917385, 1.5865729711917387, nan, 1.592309104722474, 1.5823091047224742, nan, 1.596811203896316, 1.5868112038963162, nan, 1.5931066262119133, 1.5831066262119136, nan, 1.590965267353939, 1.578965267353939, nan, 1.5964289179893894, 1.5864289179893896, nan, 1.5919117373724219, 1.581911737372422, nan, 1.5867310651422228, 1.576731065142223, nan, 1.5946590769172397, 1.5826590769172397, nan, 1.5899680475176061, 1.5799680475176063, nan, 1.592099454232746, 1.580099454232746, nan, 1.587195601241917, 1.575195601241917, nan, 1.5914707251659344, 1.5794707251659343, nan, 1.5925012245981702, 1.5805012245981702, nan, 1.5898978086861526, 1.5778978086861526, nan, 1.591800751487047, 1.5778007514870471, nan, 1.5918505559733815, 1.5778505559733818, nan, 1.5927486239152706, 1.5787486239152708, nan, 1.5925918165373358, 1.578591816537336, nan, 1.5880404634087084, 1.5740404634087086, nan, 1.5931743649291072, 1.5771743649291072, nan, 1.5939104770394237, 1.5779104770394237, nan, 1.5903664432736304, 1.5743664432736304, nan, 1.5882071958230994, 1.5702071958230996, nan, 1.5995304673682158, 1.581530467368216, nan, 1.5970072549949592, 1.5770072549949592]}, {[353.79999, 354.37, 354.94, 355.51001, 356.07999, 356.64999, 357.22, 357.78, 358.35001, 358.91, 359.47, 360.03, 360.59, 361.14999, 361.70001, 362.26001, 362.81, 363.35999, 363.91, 364.45999, 365.01001, 365.56, 366.10001, 366.64999, 367.19, 376.78, 378.87, 379.39001, 379.91, 380.42999, 380.95001, 381.47, 381.98001, 382.5, 383.01001, 383.53, 384.04001, 384.54999, 385.07001, 385.57999, 386.09, 386.60001, 387.10999, 387.62, 388.13, 388.63, 389.14001, 389.64999, 390.14999, 388.63, 389.14001, 389.64999, 390.14999, 390.66, 391.16, 391.67001, 392.17001, 392.67999, 393.17999, 393.67999, 394.17999, 394.67999, 395.19, 395.69, 396.19, 396.69, 397.19, 397.69, 398.19, 398.69, 399.19, 399.67999, 400.17999, 400.67999, 401.17999, 401.67999, 402.17001, 402.67001, 403.17001, 403.66, 404.16, 404.66, 405.14999, 405.64999, 406.14999, 406.64001, 407.14001, 407.64001, 408.13, 408.63, 409.13, 409.62, 410.12, 410.62, 411.10999, 411.60999, 412.10001, 412.60001, 413.10001, 413.60001, 414.09, 414.59, 415.09, 415.59, 416.07999, 416.57999, 417.07999, 417.57999, 418.07999, 418.57999], [1.6483722836524246, 1.6546363395359365, 1.647298907653894, 1.6533287796168583, 1.6513909602141936, 1.6441728100483295, 1.6485630092327472, 1.6465913680498476, 1.644326968253007, 1.6458723273169005, 1.6423749873362237, 1.6435071871004756, 1.6412154858600103, 1.6396834087598822, 1.6391132715105765, 1.6382846511661762, 1.6358307684719318, 1.6354408519662669, 1.6334428509272396, 1.6328074965992703, 1.630211530333035, 1.629597879928187, 1.6276773015694914, 1.6248549924331006, 1.6221911228582016, 1.6131967111234533, 1.6094507790415067, 1.6108839833096118, 1.6122492163476982, 1.6122322997299472, 1.6077321043459216, 1.6138723793940135, 1.6118005408009028, 1.6157486465235684, 1.6147077896853421, 1.6142964675684908, 1.614804272990439, 1.6117647309822476, 1.6161328124848642, 1.6101356911507883, 1.612094662439775, 1.6118531546799915, 1.614236269971587, 1.6062328837497617, 1.6105586500151539, 1.6108228692284308, 1.6178782024106462, 1.6087987962691102, 1.6074587087659151, 1.6187364188290658, 1.6209092605148896, 1.6151493452793495, 1.6182798966697, 1.6109338276299237, 1.6085077651242317, 1.613655399235577, 1.612511934789509, 1.607851046633587, 1.6057532268507935, 1.6024870719133475, 1.6038884748636346, 1.605523559015856, 1.5960101592112506, 1.5997312604952778, 1.598377877440321, 1.597392154092918, 1.600589807386528, 1.5995684913350448, 1.5979434008328421, 1.5961998900762004, 1.5970150338732805, 1.5939307380342091, 1.596156816544494, 1.5962182334684933, 1.597512896681686, 1.595101996088882, 1.5933960300930927, 1.592688229676817, 1.5913322143224218, 1.5917530088094214, 1.591614538502429, 1.5914637114820218, 1.5878221602705458, 1.5928834293750267, 1.5915729711917386, 1.587309104722474, 1.5918112038963161, 1.5881066262119135, 1.584965267353939, 1.5914289179893895, 1.586911737372422, 1.581731065142223, 1.5886590769172397, 1.5849680475176062, 1.586099454232746, 1.581195601241917, 1.5854707251659343, 1.5865012245981702, 1.5838978086861526, 1.584800751487047, 1.5848505559733816, 1.5857486239152707, 1.585591816537336, 1.5810404634087085, 1.5851743649291072, 1.5859104770394237, 1.5823664432736304, 1.5792071958230995, 1.590530467368216, 1.5870072549949592]}] ("Real Part vs wavelength")
  n1 = call <vilib>:"Add State(s) to Queue__jki_lib_state_machine.vi"("State(s) in (\"\")"="Macro: Initialize") -> ("States Out"=w2:string)  [unwired: 14 in]
  n2 = while "JKI - String-Based Queued State Machine (Basic) v1.0" {
    shift-right: [w6] -> _
    shift-left: _ -> [w5]
    shift-right: [w9] -> _
    shift-left: _ -> [w3]
    shift-right: [w8] -> _
    shift-left: w2 -> [w10]
    stop <- w7 stop-if-true
    w4 = -1  # Timeout
    # "Template Copyright © 2008 JKI - http://jkisoft.com/state-machine"
    n3 = call <vilib>:"Parse State Queue__jki_lib_state_machine.vi"("State Queue"=w10, "Error In (no error)"=w3) -> ("Remaining States"=w12:string, "Current State"=w13:string, "Arguments"=w11:string)  [unwired: 11 in]
    n4 = case shown="\"Find Global Minimum\"" w13 {
      selector: w13 -> [_ _ w180 _ _ _ _ _ _ _ _ _ _ _ _ _ _ _ _ _ _ _ _ _ _ _ _ _ _ _ _ _]
      tunnel: w12 -> [w20 w179 w184 w202 w208 w213 w217 w231 w237 w241 w246 w252 w263 w289 w294 w304 w308 w335 w371 w408 w422 w429 w508 w642 w689 w815 w883 w962 w1032 w1134 w1286 w1364]
      tunnel: w11 -> [_ _ _ _ _ _ _ _ _ _ _ w247 w257 _ _ _ _ w318 _ _ _ w423 w502 _ _ _ _ _ _ _ _ _]
      tunnel: w5 -> [w18 w176 w182 w193 w205 w211 w214 _ w232 w238 w244 w250 w259 w286 w291 w301 w305 w321 w368 w405 w419 w426 w505 w639 w686 w813 w881 w960 w1004 w1109 w1283 w1322]
      tunnel: [w17 w177 w186 w199 errorcluster {"status"=FALSE, "code"=0, "source"=""} ("error out") w210 w215 w228 w233 w239 w243 w248 w260 w287 w292 w302 w306 w333 w369 w406 w420 w427 w506 w640 w687 w812 w880 w959 w1030 w1132 w1284 w1362] -> w9
      tunnel: w3 -> [w16 w177 w185 w199 w204 w210 w215 w228 w234 w239 w243 w249 w261 w287 w292 w302 w306 w333 w369 w406 w420 w427 w506 w640 w687 w812 w880 w959 w1030 w1132 w1284 w1362]
      tunnel: [w19 w178 w183 w201 w207 w212 w216 w230 w236 w240 w245 w251 w262 w288 w293 w303 w307 w334 w370 w407 w421 w428 w507 w641 w688 w814 w882 w961 w1031 w1133 w1285 w1363] -> w8
      tunnel: [_ _ _ _ _ TRUE _ _ _ _ _ _ _ _ _ _ _ _ _ _ _ _ _ _ _ _ _ _ _ _ _ _] -> w7
      tunnel: [w15 w176 w182 w200 w205 w211 w214 w229 w232 w238 w244 w250 w259 w286 w291 w301 w305 w332 w367 w405 w418 w425 w504 w638 w685 w813 w881 w960 w1003 w1108 w1283 w1321] -> w6
      tunnel: w4 -> [w14 _ _ _ _ _ _ _ _ _ _ _ _ _ _ _ _ _ _ _ _ _ _ _ _ _ _ _ _ _ _ _]
      frame "", "Idle" {
        # "executes when the state queue is empty"
        n5 = event shown="[8] \"Find Global Minima\": Value Change" {
          selector: _ -> [_ _ _ _ _ _ _ _ _ _ _ _ _ _ _ _ _ _ _ _ _ _ _]
          dyn-events: _ -> [_ _ _ _ _ _ _ _ _ _ _ _ _ _ _ _ _ _ _ _ _ _ _]
          timeout: w14 -> [_ _ _ _ _ _ _ _ _ _ _ _ _ _ _ _ _ _ _ _ _ _ _]
          tunnel: w20 -> [w24 w33 w53 w59 w65 w71 w76 w84 w93 w99 w104 w109 w114 w119 w124 w129 w134 w141 w148 w156 w161 w169 w175]
          tunnel: [w23 w32 w52 w58 w64 w70 w75 w83 w92 w98 w103 w108 w113 w118 w123 w128 w133 w140 w147 w155 w160 w168 w174] -> w19
          tunnel: w18 -> [w21 w30 w50 w56 w62 w68 w73 w81 w90 w96 w101 w106 w111 w116 w121 w126 w131 w136 w143 w153 w158 w166 w172]
          tunnel: [w22 w31 w51 w57 w63 w69 w74 w82 w91 w97 w102 w107 w112 w117 w122 w127 w132 w139 w146 w154 w159 w167 w173] -> w17
          tunnel: w16 -> [w22 w31 w51 w57 w63 w69 w74 w82 w91 w97 w102 w107 w112 w117 w122 w127 w132 w139 w146 w154 w159 w167 w173]
          tunnel: [w21 w30 w50 w56 w62 w68 w73 w81 w90 w96 w101 w106 w111 w116 w121 w126 w131 w135 w142 w153 w158 w166 w172] -> w15
          event Timeout {
            # "Timeout Frame\n(this will only execute if the Event Structure timeout is >= 0)"
            n6 = event-data() -> ()  [unwired: 1 in, 1 out]
            n7 = call <vilib>:"Add State(s) to Queue__jki_lib_state_machine.vi"("State(s) in (\"\")"=w24) -> ("States Out"=w23:string)  [unwired: 14 in]
          }
          event "Diameters to fit": Mouse Down {
            # "Timeout Frame\n(this will only execute if the Event Structure timeout is >= 0)"
            n8 = event-data() -> ("Coords"=w29:T15)  [unwired: 1 in, 7 out]
            n9 = case shown="True" "Quick Fit" {
              tunnel: ["" w36] -> w25
              frame False {
              }
              frame True {
                n10 = local read "Use Factors"() -> (w35:bool)
                n11 = Select(t="Load Files >> Dont Initialize Sizes\nRetrieve RI >> UseFactors", s=w35, f="Load Files >> Dont Initialize Sizes\nRetrieve RI >> DontUseFactors") -> (s? t:f=w36:string)
                n12 = case shown="False" w35 {
                  frame False {
                  }
                  frame True {
                    n13 = One Button Dialog(message="You are using Extinction factor and Diameter factors/offset in this calculation !!") -> ()  [unwired: 1 in, 1 out]
                  }
                }
              }
            }
            n14 = invoke on="Diameters to fit" class="LstBox (strict)" method="Point To Row"("Point"=w29) -> ("Row"=w28:i32, "InGlyph"=w27:bool)  [unwired: 6 in, 5 out]
            n15 = case shown="True" w27 {
              tunnel: w28 -> [_ w47]
              frame False {
              }
              frame True {
                w43 = 37 ("Item Symbols")
                n16 = property on="Diameters to fit" class="LstBox (strict)"() -> ("Item Symbols"=w40:i32[])  [unwired: 2 in, 2 out]
                n17 = Index Array(array=w40, index=w47) -> (element=w46:i32)
                n18 = Equal?(x=w46, y=w43) -> (x = y?=w45:bool)
                n19 = Select(t=38 ("Item Symbols"), s=w45, f=w43) -> (s? t:f=w44:i32)
                n20 = Replace Array Subset(array=w40, new element=w44, index=w47) -> (w41:i32[])
                n21 = property on="Diameters to fit" class="LstBox (strict)"("Item Symbols"=w41) -> ()  [unwired: 2 in, 2 out]
              }
            }
            n22 = call <vilib>:"Add State(s) to Queue__jki_lib_state_machine.vi"("State(s) in Front (\"\")"=w25, "State(s) in (\"\")"=w33) -> ("States Out"=w32:string)  [unwired: 13 in]
          }
          event "Diamter Offset Radio Button": Mouse Up {
            w48 = TRUE ("Diamter Offset Radio Button")
            # "Timeout Frame\n(this will only execute if the Event Structure timeout is >= 0)"
            n23 = event-data() -> ()  [unwired: 1 in, 8 out]
            n24 = local write "Diamter Offset Radio Button"(w48) -> ()
            n25 = local write "Diameter Factor Radio Button"(FALSE ("Diameter Factor Radio Button")) -> ()
            n26 = local write "Diameter Factor or Offset"(w48) -> ()
            n27 = call <vilib>:"Add State(s) to Queue__jki_lib_state_machine.vi"("State(s) in (\"\")"=w53) -> ("States Out"=w52:string)  [unwired: 14 in]
          }
          event "Diameter Factor Radio Button": Mouse Up {
            w54 = FALSE ("Diamter Offset Radio Button")
            # "Timeout Frame\n(this will only execute if the Event Structure timeout is >= 0)"
            n28 = event-data() -> ()  [unwired: 1 in, 8 out]
            n29 = local write "Diamter Offset Radio Button"(w54) -> ()
            n30 = local write "Diameter Factor Radio Button"(TRUE ("Diameter Factor Radio Button")) -> ()
            n31 = local write "Diameter Factor or Offset"(w54) -> ()
            n32 = call <vilib>:"Add State(s) to Queue__jki_lib_state_machine.vi"("State(s) in (\"\")"=w59) -> ("States Out"=w58:string)  [unwired: 14 in]
          }
          event "Imaginary Part vs wavelength": Cursor Move {
            # "Timeout Frame\n(this will only execute if the Event Structure timeout is >= 0)"
            n33 = event-data() -> ()  [unwired: 1 in, 9 out]
            n34 = property on="Imaginary Part vs wavelength" class="XYGraph (strict)"() -> ("Cursor.Cursor X"=w61:dbl)  [unwired: 2 in, 2 out]
            n35 = property on="Real Part vs wavelength" class="XYGraph (strict)"("Cursor.Cursor X"=w61) -> ()  [unwired: 2 in, 2 out]
            n36 = call <vilib>:"Add State(s) to Queue__jki_lib_state_machine.vi"("State(s) in Front (\"\")"="Update Corrected multiple charge extinction graph" ("State(s) in Front (\"\")"), "State(s) in (\"\")"=w65) -> ("States Out"=w64:string)  [unwired: 13 in]
          }
          event "Real Part vs wavelength": Cursor Move {
            n37 = event-data() -> ()  [unwired: 1 in, 9 out]
            n38 = property on="Real Part vs wavelength" class="XYGraph (strict)"() -> ("Cursor.Cursor X"=w67:dbl)  [unwired: 2 in, 2 out]
            n39 = property on="Imaginary Part vs wavelength" class="XYGraph (strict)"("Cursor.Cursor X"=w67) -> ()  [unwired: 2 in, 2 out]
            n40 = call <vilib>:"Add State(s) to Queue__jki_lib_state_machine.vi"("State(s) in Front (\"\")"="Update Corrected multiple charge extinction graph" ("State(s) in Front (\"\")"), "State(s) in (\"\")"=w71) -> ("States Out"=w70:string)  [unwired: 13 in]
          }
          event "OK": Value Change {
            # "Exit Button Value Change (pressed) Event\n(this executes Macro: Exit to terminate the VI)"
            n41 = event-data() -> ()  [unwired: 1 in, 1 out]
            n42 = call <vilib>:"Add State(s) to Queue__jki_lib_state_machine.vi"("State(s) in Front (\"\")"="Macro: Exit", "State(s) in (\"\")"=w76) -> ("States Out"=w75:string)  [unwired: 13 in]
          }
          event "Retrieve RI": Value Change {
            # "Exit Button Value Change (pressed) Event\n(this executes Macro: Exit to terminate the VI)"
            n43 = event-data() -> ()  [unwired: 1 in, 6 out]
            n44 = Select(t="Load Files >> Dont Initialize Sizes\nRetrieve RI >> UseFactors", s="Use Factors", f="Load Files >> Dont Initialize Sizes\nRetrieve RI >> DontUseFactors") -> (s? t:f=w80:string)
            n45 = case shown="False" "Use Factors" {
              frame False {
              }
              frame True {
                n46 = One Button Dialog(message="You are using Extinction factor and Diameter factors/offset in this calculation !!") -> ()  [unwired: 1 in, 1 out]
              }
            }
            n47 = call <vilib>:"Add State(s) to Queue__jki_lib_state_machine.vi"("State(s) in Front (\"\")"=w80, "State(s) in (\"\")"=w84) -> ("States Out"=w83:string)  [unwired: 13 in]
          }
          event "Find Global Minima": Value Change {
            # "Exit Button Value Change (pressed) Event\n(this executes Macro: Exit to terminate the VI)"
            n48 = event-data() -> ()  [unwired: 1 in, 6 out]
            n49 = local read "Use Factors"() -> (w86:bool)
            n50 = Select(t="Load Files >> Dont Initialize Sizes\nFind Global Minimum >> UseFactors", s=w86, f="Load Files >> Dont Initialize Sizes\nFind Global Minimum >> DontUseFactors") -> (s? t:f=w89:string)
            n51 = case shown="False" w86 {
              frame False {
              }
              frame True {
                n52 = One Button Dialog(message="You are using Extinction factor and Diameter factors/offset in this calculation !!") -> ()  [unwired: 1 in, 1 out]
              }
            }
            n53 = call <vilib>:"Add State(s) to Queue__jki_lib_state_machine.vi"("State(s) in Front (\"\")"=w89, "State(s) in (\"\")"=w93) -> ("States Out"=w92:string)  [unwired: 13 in]
          }
          event "Retrieve RI Calculate lines seperately": Value Change {
            # "Exit Button Value Change (pressed) Event\n(this executes Macro: Exit to terminate the VI)"
            n54 = event-data() -> ()  [unwired: 1 in, 6 out]
            n55 = call <vilib>:"Add State(s) to Queue__jki_lib_state_machine.vi"("State(s) in Front (\"\")"="Load Files MC\nRetrieve RI", "State(s) in (\"\")"=w99) -> ("States Out"=w98:string)  [unwired: 13 in]
          }
          event "Retrieve RI without taking the mean (MC)": Value Change {
            # "Exit Button Value Change (pressed) Event\n(this executes Macro: Exit to terminate the VI)"
            n56 = event-data() -> ()  [unwired: 1 in, 6 out]
            n57 = call <vilib>:"Add State(s) to Queue__jki_lib_state_machine.vi"("State(s) in Front (\"\")"="Load Files MC\nRetreive RI from Single Measurements(MC)", "State(s) in (\"\")"=w104) -> ("States Out"=w103:string)  [unwired: 13 in]
          }
          event "Save RI": Value Change {
            # "Exit Button Value Change (pressed) Event\n(this executes Macro: Exit to terminate the VI)"
            n58 = event-data() -> ()  [unwired: 1 in, 6 out]
            n59 = call <vilib>:"Add State(s) to Queue__jki_lib_state_machine.vi"("State(s) in Front (\"\")"="Save RI to file", "State(s) in (\"\")"=w109) -> ("States Out"=w108:string)  [unwired: 13 in]
          }
          event "Save RI expanded Edition": Value Change {
            # "Exit Button Value Change (pressed) Event\n(this executes Macro: Exit to terminate the VI)"
            n60 = event-data() -> ()  [unwired: 1 in, 6 out]
            n61 = call <vilib>:"Add State(s) to Queue__jki_lib_state_machine.vi"("State(s) in Front (\"\")"="Save RI to File Expanded Edition", "State(s) in (\"\")"=w114) -> ("States Out"=w113:string)  [unwired: 13 in]
          }
          event "Find Extinction Factor Graph": Value Change {
            # "Exit Button Value Change (pressed) Event\n(this executes Macro: Exit to terminate the VI)"
            n62 = event-data() -> ()  [unwired: 1 in, 6 out]
            n63 = call <vilib>:"Add State(s) to Queue__jki_lib_state_machine.vi"("State(s) in Front (\"\")"="Load Files >> Dont Initialize Sizes\nFind Extinction Factor", "State(s) in (\"\")"=w119) -> ("States Out"=w118:string)  [unwired: 13 in]
          }
          event "Plot RI": Value Change {
            # "Exit Button Value Change (pressed) Event\n(this executes Macro: Exit to terminate the VI)"
            n64 = event-data() -> ()  [unwired: 1 in, 6 out]
            n65 = call <vilib>:"Add State(s) to Queue__jki_lib_state_machine.vi"("State(s) in Front (\"\")"="Append Mie Curve", "State(s) in (\"\")"=w124) -> ("States Out"=w123:string)  [unwired: 13 in]
          }
          event "Save RI MC": Value Change {
            # "Exit Button Value Change (pressed) Event\n(this executes Macro: Exit to terminate the VI)"
            n66 = event-data() -> ()  [unwired: 1 in, 6 out]
            n67 = call <vilib>:"Add State(s) to Queue__jki_lib_state_machine.vi"("State(s) in Front (\"\")"="Save RI -Monte Carlo to file", "State(s) in (\"\")"=w129) -> ("States Out"=w128:string)  [unwired: 13 in]
          }
          event "Retrieve RI (MC)": Value Change {
            # "Exit Button Value Change (pressed) Event\n(this executes Macro: Exit to terminate the VI)"
            n68 = event-data() -> ()  [unwired: 1 in, 6 out]
            n69 = call <vilib>:"Add State(s) to Queue__jki_lib_state_machine.vi"("State(s) in Front (\"\")"="Load Files\nRetrieve RI Monte Carlo", "State(s) in (\"\")"=w134) -> ("States Out"=w133:string)  [unwired: 13 in]
          }
          event "Extinction Cross Section File": Value Change {
            # "Exit Button Value Change (pressed) Event\n(this executes Macro: Exit to terminate the VI)"
            n70 = event-data() -> ()  [unwired: 1 in, 6 out]
            n71 = local read "Extinction Cross Section File"() -> (w137:path)
            n72 = Bundle By Name(cluster=w136, "Extinction Cross section Path"=w137) -> (w135:T17)
            n73 = call <vilib>:"Add State(s) to Queue__jki_lib_state_machine.vi"("State(s) in Front (\"\")"="Load Files >> Initialize Sizes\nUpdate Window after Load Files", "State(s) in (\"\")"=w141) -> ("States Out"=w140:string)  [unwired: 13 in]
          }
          event "Mutiple Charge Data File": Value Change {
            # "Exit Button Value Change (pressed) Event\n(this executes Macro: Exit to terminate the VI)"
            n74 = event-data() -> ()  [unwired: 1 in, 6 out]
            n75 = local read "Mutiple Charge Data File"() -> (w144:path)
            n76 = Bundle By Name(cluster=w143, "Multiple charge correction file Path"=w144) -> (w142:T17)
            n77 = call <vilib>:"Add State(s) to Queue__jki_lib_state_machine.vi"("State(s) in Front (\"\")"="Load Files\nUpdate Window after Load Files", "State(s) in (\"\")"=w148) -> ("States Out"=w147:string)  [unwired: 13 in]
          }
          event "Calculate Errors": Value Change {
            # "Exit Button Value Change (pressed) Event\n(this executes Macro: Exit to terminate the VI)"
            n78 = event-data() -> ("NewVal"=w152:bool)  [unwired: 1 in, 5 out]
            n79 = Select(t=FALSE, s=w152, f=FALSE) -> (s? t:f=w150:bool)
            n80 = property on="Approximate Errors" class="Bool (strict)"("Visible"=w152) -> ()  [unwired: 2 in, 2 out]
            n81 = property on="Approximate Errors" class="Bool (strict)"("Value"=w150) -> ()  [unwired: 2 in, 2 out]
            n82 = call <vilib>:"Add State(s) to Queue__jki_lib_state_machine.vi"("State(s) in (\"\")"=w156) -> ("States Out"=w155:string)  [unwired: 14 in]
          }
          event "ShiftSMPStoSizes": Value Change {
            # "Exit Button Value Change (pressed) Event\n(this executes Macro: Exit to terminate the VI)"
            n83 = event-data() -> ()  [unwired: 1 in, 6 out]
            n84 = call <vilib>:"Add State(s) to Queue__jki_lib_state_machine.vi"("State(s) in Front (\"\")"="ShiftSMPStoSizes" ("State(s) in Front (\"\")"), "State(s) in (\"\")"=w161) -> ("States Out"=w160:string)  [unwired: 13 in]
          }
          event "autoscale": Value Change {
            n85 = event-data() -> ()  [unwired: 1 in, 6 out]
            n86 = property on="Imaginary Part vs wavelength" class="XYGraph (strict)"("XScale.ScaleFit"=u8 1 ("X Scale.Scale Fit"), "YScale.ScaleFit"=u8 1 ("Y Scale.Scale Fit")) -> ()  [unwired: 2 in, 2 out]
            n87 = property on="Real Part vs wavelength" class="XYGraph (strict)"("XScale.ScaleFit"=u8 1 ("X Scale.Scale Fit"), "YScale.ScaleFit"=u8 1 ("Y Scale.Scale Fit")) -> ()  [unwired: 2 in, 2 out]
            n88 = call <vilib>:"Add State(s) to Queue__jki_lib_state_machine.vi"("State(s) in (\"\")"=w169) -> ("States Out"=w168:string)  [unwired: 14 in]
          }
          event Panel Close? {
            # "Discard the event because we'll close the front panel ourselves in Macro: Exit"
            # "Close Panel button (pressed) Event\n(this executes Macro: Exit to terminate the VI)"
            n89 = event-data() -> ()  [unwired: 1 in, 1 out]
            n90 = call <vilib>:"Add State(s) to Queue__jki_lib_state_machine.vi"("State(s) in Front (\"\")"="Macro: Exit", "State(s) in (\"\")"=w175) -> ("States Out"=w174:string)  [unwired: 13 in]
            n91 = event-data("Discard?"=TRUE) -> ()  [unwired: 1 in, 1 out]
          }
        }
      }
      frame "---------- Core ----------" {
        # "Do not put any code in this frame.\n(it is a separator no-op)"
        n92 = call <vilib>:"Add State(s) to Queue__jki_lib_state_machine.vi"("State(s) in (\"\")"=w179) -> ("States Out"=w178:string)  [unwired: 14 in]
      }
      frame Default {
        w189 = 42 items=["No error", "Argument error", "Memory is full", "Out of zone", "End of file", "File already open", "Generic file I/O error", "File not found", "File permission error", "Disk is full", "Duplicate path", "Too many files open", "System feature not enabled", "Resource file not found", "Cannot add resource", "Resource not found", "Image not found", "Image memory error", "Pen does not exist", "Config type invalid", "Config token not found", "Config parse error", "Config memory error", "Bad external code format", "Bad external code offset", "External code not present", "Null window", "Destroy window error", "Null menu", "Print aborted", "Bad print record", "Print driver error", "Windows error during printing", "Memory error during printing", "Print dialog error", "Generic print error", "Invalid device refnum", "Device not found", "Device parameter error", "Device unit error", "Cannot open device", "Device call aborted", "Generic error", "Cancelled by user", "Object ID too low", "Object ID too high", "Object not in heap", "Unknown heap", "Unknown object (invalid DefProc)", "Unknown object (DefProc not in table)", "Message out of range", "Invalid (null) method", "Unknown message", "Manager call not supported", "Bad address", "Network operation in progress", "Network operation timed out", "Connection is busy", "Network attribute not supported", "Network error", "Address in use", "System out of memory", "Connection aborted", "Connection refused", "Not connected", "Already connected", "Connection closed", "Initialization error (interapplication manager)", "Bad occurrence", "Wait on unbound occurrence handler", "Occurrence queue overflow", "Datalog type conflict", "Unused", "Unrecognized type (interapplication manager)", "Memory corrupt", "Failed to make temporary DLL", "Old CIN version", "Drag socket not found", "Failed to load drop-object", "Failed to register OLE object", "Failed to release OLE object", "Format specifier type mismatch", "Unknown format specifier", "Too few format specifiers", "Too many format specifiers", "Scan failed", "Newer CIN version", "Error converting to variant", "Runtime menu error", "Password tampered", "Variant attribute not found", "Incompatible variant data type", "Event data is not available", "Event Store is not present", "Occurrence is not found", "Event Queue is not created", "Event info is not available", "Refnum passed is NULL", "Error retrieving Class GUID", "Error retrieving CoClass GUID", "Error retrieving TypeLib GUID.", "Bad built application magic bytes.", "Specific driver is different from the specific driver associated with the Logical Name.", "There is no session opened to the class driver.", "Max Error", "MAX - Error with config objects", "MAX - Error loading configuration", "MAX - Group not supported"]
        # "Current State"
        # "Do not delete, rename, or modify this frame.\n(this is used to capture unhandled states and typos)"
        # "Handle mistyped state name (developer tool)"
        n93 = call <vilib>:"Add State(s) to Queue__jki_lib_state_machine.vi"("State(s) in (\"\")"=w184) -> ("States Out"=w183:string)  [unwired: 14 in]
        n94 = Format Into String(format string="Software Exception: Unhandled State \"%s\"." ("message"), error in=w185, w180) -> (resulting string=w188:string, error out=w187:errorcluster)  [unwired: 1 in]
        n95 = call <vilib>:"Error Cluster From Error Code.vi"("show call chain? (False)"=TRUE, "error in (no error)"=w187, "error message (\"\")"=w188, "error code (0)"=w189) -> ("error out"=w186:errorcluster)  [unwired: 5 in]
      }
      frame "Initialize Core Data" {
        # "Do not delete, rename, or modify this frame.\n(this is used to determine panel behavior on exit)"
        # "originally closed?"
        # "exe?"
        # "If panel starts closed or is an EXE, then close it when we exit"
        n96 = call <vilib>:"Add State(s) to Queue__jki_lib_state_machine.vi"("State(s) in (\"\")"=w202) -> ("States Out"=w201:string)  [unwired: 14 in]
        n97 = property class="App"() -> ("App.Kind"=w197:T11)  [unwired: 2 in, 2 out]
        n98 = property class="VI"() -> ("Front Panel.Open"=w198:bool)  [unwired: 2 in, 2 out]
        n99 = Equal?(x=w197, y=T11."Run Time System" ("Application:Kind")) -> (x = y?=w194:bool)
        n100 = Not(x=w198) -> (.not. x?=w195:bool)
        n101 = Or(x=w195, y=w194) -> (x .or. y?=w192:bool)
        n102 = control-ref of="Current VI Reference"() -> (w191:refnum<vi>)
        n103 = Bundle By Name(cluster=w193, "Core.Current VI Reference"=w191, "Core.Close Panel on Exit?"=w192) -> (w200:T17)
      }
      frame "Error Handler" {
        # "Unhandled Error -- Display it"
        # "Handle any errors here.\nYou can also output any states to clean-up after errors occur"
        # "Clear error"
        n104 = call <vilib>:"General Error Handler.vi"("error in (no error)"=w204) -> ()  [unwired: 10 in, 5 out]
        n105 = call <vilib>:"Add State(s) to Queue__jki_lib_state_machine.vi"("State(s) in Front (\"\")"="/* Post Error States", "State(s) in (\"\")"=w208) -> ("States Out"=w207:string)  [unwired: 13 in]
      }
      frame "Exit" {
        # "Do not put any code in this frame.\n(No errors that occur here will be handled.)"
        n106 = call <vilib>:"Add State(s) to Queue__jki_lib_state_machine.vi"("State(s) in (\"\")"=w213) -> ("States Out"=w212:string)  [unwired: 14 in]
      }
      frame "---------- Data ----------" {
        # "Do not put any code in this frame.\n(It is a separator no-op. You can make a copy of this frame to create a new Data frame)"
        n107 = call <vilib>:"Add State(s) to Queue__jki_lib_state_machine.vi"("State(s) in (\"\")"=w217) -> ("States Out"=w216:string)  [unwired: 14 in]
      }
      frame "Data: Initialize" {
        w219 = 0  # NumberOfMeasurementsperSize
        w220 = dbl[][] []  # FullExtinctionData
        w221 = path ""  # Multiple charge correction file Path
        w222 = path ""  # Extinction Cross section Path
        w223 = T16 {"Real RI"=[], "Imaginary RI"=[], "Std Imaginary RI"=[], "Std Real RI"=[], "Wavelength"=[], "Residue"=[], "Extinction Factor"=[], "Diameter Factor"=[], "Diameter Offset"=[], "Best fit result"=[], "Normalized Residuals"=[]}  # RI MC results
        w224 = T16 {"Real RI"=[], "Imaginary RI"=[], "Std Imaginary RI"=[], "Std Real RI"=[], "Wavelength"=[], "Residue"=[], "Extinction Factor"=[], "Diameter Factor"=[], "Diameter Offset"=[], "Best fit result"=[], "Normalized Residuals"=[]}  # RI results
        w225 = T8 {"SMPS Sizes"=[], "Concentration"=[], "Double Charge Correction Flag"=FALSE}  # Particle Distribution Data
        w226 = T7 {"Extinction"=[], "Extinction Uncertainty"=[], "Size parameters"=[], "Number ofSizes"=0.0, "GeometricCrossSection"=[], "WaveLength"=[], "Sizes"=[], "Concentration (#/cc)"=[]}  # Extinction ExtinctionUncertainity Size parameter and Number ofS sizes
        w227 = T18 {"Current VI Reference"=refnum, "Close Panel on Exit?"=FALSE}  # Core
        # "do not delete - used by framework"
        # "Data names and types of shift register data are defined by this bundle."
        # "Initialize the shift-register data, here.\n(data names are defined by what you wire into the bundle function)"
        n108 = call <vilib>:"Add State(s) to Queue__jki_lib_state_machine.vi"("State(s) in (\"\")"=w231) -> ("States Out"=w230:string)  [unwired: 14 in]
        n109 = Bundle("Core"=w227, "Extinction ExtinctionUncertainity Size parameter and Number ofS sizes"=w226, "Particle Distribution Data"=w225, "RI results"=w224, "RI MC results"=w223, "Extinction Cross section Path"=w222, "Multiple charge correction file Path"=w221, "FullExtinctionData"=w220, "NumberOfMeasurementsperSize"=w219, "Baes data type definition"="Baes data type definition") -> (w229:T17)  [unwired: 1 in]
      }
      frame "Data: Cleanup" {
        # "Cleanup any data and references, here.\n(this is called automatically, by the Macro: Exit)"
        n110 = Unbundle By Name(w232) -> ("Core.Current VI Reference"=w235:refnum<vi>)
        n111 = call <vilib>:"Add State(s) to Queue__jki_lib_state_machine.vi"("State(s) in (\"\")"=w237) -> ("States Out"=w236:string)  [unwired: 14 in]
        n112 = Close Reference(reference=w235, error in (no error)=w234) -> (error out=w233:errorcluster)
      }
      frame "---------- UI ----------" {
        # "Do not put any code in this frame.\n(It is a separator no-op. You can make a copy of this frame to create a new UI frame)"
        n113 = call <vilib>:"Add State(s) to Queue__jki_lib_state_machine.vi"("State(s) in (\"\")"=w241) -> ("States Out"=w240:string)  [unwired: 14 in]
      }
      frame "UI: Initialize" {
        # "Initialize the User Interface, here.\n(this is called automatically, by the Macro: Init)"
        n114 = call <vilib>:"Add State(s) to Queue__jki_lib_state_machine.vi"("State(s) in (\"\")"=w246) -> ("States Out"=w245:string)  [unwired: 14 in]
        n115 = property on="Retrieve RI" class="Bool"("BoolText.Text"="Retrieve RI" ("Boolean Text.Text")) -> ()  [unwired: 2 in, 2 out]
      }
      frame "UI: Cursor Set" {
        # "Argument"
        # "Set and Unset Cursor Busy.\n(Usage: \"UI: Cursor Set >> Busy|Idle\")"
        n116 = call <vilib>:"Add State(s) to Queue__jki_lib_state_machine.vi"("State(s) in (\"\")"=w252) -> ("States Out"=w251:string)  [unwired: 14 in]
        n117 = case shown="\"Idle\", Default" w247 {
          tunnel: w249 -> [w254 w256]
          tunnel: [w253 w255] -> w248
          frame "Idle", Default {
            n118 = call <vilib>:"Unset Busy.vi"("error in (no error)"=w254) -> ("error out"=w253:errorcluster)  [unwired: 10 in]
          }
          frame "Busy" {
            n119 = call <vilib>:"Set Busy.vi"("error in (no error)"=w256) -> ("error out"=w255:errorcluster)  [unwired: 9 in, 1 out]
          }
        }
      }
      frame "UI: Front Panel State" {
        # "Argument"
        # "Set Front Panel Open or Closed\n(Usage: \"UI: Front Panel State >> Open|Close\")"
        n120 = Unbundle By Name(w259) -> ("Core.Current VI Reference"=w258:refnum<vi>)
        n121 = call <vilib>:"Add State(s) to Queue__jki_lib_state_machine.vi"("State(s) in (\"\")"=w263) -> ("States Out"=w262:string)  [unwired: 14 in]
        n122 = case shown="\"Open\", Default" w257 {
          tunnel: w261 -> [w267 w280]
          tunnel: [w269 w281] -> w260
          tunnel: w258 -> [w268 w278]
          frame "Open", Default {
            n123 = property class="VI"(reference=w268, error in=w267) -> (reference out=w265:refnum<vi>, error out=w266:errorcluster, "Front Panel.Open"=w264:bool)
            n124 = case shown="False" w264 {
              tunnel: [w272 w275] -> w269
              tunnel: w266 -> [w271 w275]
              tunnel: w265 -> [w270 _]
              frame False {
                n125 = invoke class="VI" method="FP.Open"(reference=w270, error in=w271, "Activate"=TRUE, "State"=T12."Standard") -> (error out=w272:errorcluster)  [unwired: 1 in, 4 out]
              }
              frame True {
              }
            }
          }
          frame "Close" {
            n126 = property class="VI"(reference=w278, error in=w280) -> (reference out=w277:refnum<vi>, error out=w279:errorcluster, "Front Panel.Open"=w276:bool)
            n127 = case shown="True" w276 {
              tunnel: [w282 w285] -> w281
              tunnel: w279 -> [w282 w284]
              tunnel: w277 -> [_ w283]
              frame False {
              }
              frame True {
                n128 = invoke class="VI" method="FP.Close"(reference=w283, error in=w284) -> (error out=w285:errorcluster)  [unwired: 1 in, 2 out]
              }
            }
          }
        }
      }
      frame "---------- Macro ----------" {
        # "Do not put any code in this frame.\n(It is a separator no-op. You can make a copy of this frame to create a new Macro frame)"
        n129 = call <vilib>:"Add State(s) to Queue__jki_lib_state_machine.vi"("State(s) in (\"\")"=w289) -> ("States Out"=w288:string)  [unwired: 14 in]
      }
      frame "Macro: Initialize" {
        w290 = "Data: Initialize\nInitialize Core Data\nUI: Initialize\nUI: Front Panel State >> Open"  # Data: Initialize Initialize Core Data UI: Initialize UI: Front Panel State >> Open
        # "Initialization Macro\n(This is called once, when the VI starts)"
        n130 = call <vilib>:"Add State(s) to Queue__jki_lib_state_machine.vi"("State(s) in Front (\"\")"=w290, "State(s) in (\"\")"=w294) -> ("States Out"=w293:string)  [unwired: 13 in]
      }
      frame "Macro: Exit" {
        # "Exit Macro\n(This is called once, when the VI exits)"
        n131 = Unbundle By Name(w301) -> ("Core.Close Panel on Exit?"=w300:bool)
        n132 = Select(t="UI: Front Panel State >> Close", s=w300, f="") -> (s? t:f=w297:string)
        n133 = call <vilib>:"Add State(s) to Queue__jki_lib_state_machine.vi"("State(s) in (\"\")"=w297, "State(s) at Back (\"\")"="Data: Cleanup\nExit") -> ("States Out"=w295:string)  [unwired: 13 in]
        n134 = call <vilib>:"Add State(s) to Queue__jki_lib_state_machine.vi"("State(s) in Front (\"\")"=w295, "State(s) in (\"\")"=w304) -> ("States Out"=w303:string)  [unwired: 13 in]
      }
      frame "---------- New Category ----------" {
        # "Template Separator\n(You can make a copy of, or modify, this frame)"
        n135 = call <vilib>:"Add State(s) to Queue__jki_lib_state_machine.vi"("State(s) in (\"\")"=w308) -> ("States Out"=w307:string)  [unwired: 14 in]
      }
      frame "Load Files" {
        n136 = call <vilib>:"Add State(s) to Queue__jki_lib_state_machine.vi"("State(s) in (\"\")"=w335) -> ("States Out"=w334:string)  [unwired: 14 in]
        n137 = Unbundle By Name(w321) -> ("Extinction Cross section Path"=w320:path, "Multiple charge correction file Path"=w319:path)
        n138 = call "ReadBAESdataFromFileVer3.vi"("Factor Size Parameter"=1.0, "Factor Extinction"="Extinction Factor in Data", "Factor Ext Uncertainty"="Factor Ext Uncertainty in Data", "file path"=w320) -> ("Extinction data in graph format"=→"Extinction Data per size":T19, "Extinction ExtinctionUncertainity Size parameter and Number ofS sizes"=w314:T7)
        n139 = call "ReadParticleSizeSpectrum.vi"("file path"=w319, "Factor Size paramter"=1.0) -> ("Particle Distribution Data"=w315:T8)  [unwired: 1 out]
        n140 = Strip Path(path=w320) -> (stripped path=w323:path, name=w327:string)
        n141 = Strip Path(path=w319) -> (stripped path=w322:path, name=w325:string)
        n142 = case shown="\"Initialize Sizes\"" w318 {
          tunnel: w314 -> [_ w353 _]
          frame "False", Default {
          }
          frame "Initialize Sizes" {
            n143 = Unbundle By Name(w353) -> ("Number ofSizes"=w352:dbl, "Sizes"=w351:dbl[])
            n144 = for {
              N: w352 -> [_]
              tunnel: [w358] -> w354 mode=indexing
              tunnel: w351 -> [w357] mode=indexing
              n145 = Number To Decimal String(number=w357) -> (decimal integer string=w358:string)  [unwired: 1 in]
            }
            n146 = Initialize Array(38 ("Item Symbols"), w352) -> (w355:i32[])
            n147 = property on="Diameters to fit" class="LstBox (strict)"("Item Symbols"=w355, "Item Names"=w354) -> ()  [unwired: 2 in, 2 out]
          }
          frame "Dont Initialize Sizes" {
          }
        }
        n148 = property on="Extinction Cross Section File" class="Path"("StartPath"=w323) -> ()  [unwired: 2 in, 2 out]
        n149 = property on="Mutiple Charge Data File" class="Path"("StartPath"=w322) -> ()  [unwired: 2 in, 2 out]
        n150 = case shown="False" "Correct SMPS sizes to selected Sizes" {
          tunnel: [w341 w343] -> w313
          tunnel: w315 -> [w341 w346]
          tunnel: w314 -> [_ w348]
          frame False {
          }
          frame True {
            n151 = Unbundle By Name(w346) -> ("Concentration"=w350:dbl[][], "SMPS Sizes"=w349:dbl[])
            n152 = Unbundle By Name(w348) -> ("Sizes"=w347:dbl[])
            n153 = call "Find and Shift SMPS sizes according to selected Peak Position.vi"("Sizes"=w347, "SMPS Sizes"=w349, "Concentration"=w350, "method"=3) -> ("SMPS sizes"=w344:dbl[], "Shifted Concentration"=w345:dbl[][])  [unwired: 5 in, 1 out]
            n154 = Bundle By Name(cluster=w346, "Concentration"=w345, "SMPS Sizes"=w344) -> (w343:T8)
          }
        }
        n155 = Unbundle By Name(w313) -> ("SMPS Sizes"=w312:dbl[], "Concentration"=w311:dbl[][])
        n156 = Bundle By Name(cluster=w321, "Extinction ExtinctionUncertainity Size parameter and Number ofS sizes"=w314, "Particle Distribution Data"=w313) -> (w332:T17)
        n157 = for {
          tunnel: w312 -> [w338]
          tunnel: w311 -> [w337] mode=indexing
          shift-right: [w340] -> w309
          shift-left: T13 [] -> [w339]
          n158 = Bundle("SMPS Sizes"=w338, "Concentration"=w337) -> (w336:T20)  [unwired: 1 in]
          n159 = Build Array (concatenate)(w339, w336) -> (w340:T13)
        }
        "Size Distribution" <- w309
        n160 = String To Path(string=w327) -> (path=w326:path)
        n161 = String To Path(string=w325) -> (path=w324:path)
        n162 = local write "Extinction Cross Section File"(w326) -> ()
        n163 = local write "Mutiple Charge Data File"(w324) -> ()
      }
      frame "ShiftSMPStoSizes" {
        n164 = call <vilib>:"Add State(s) to Queue__jki_lib_state_machine.vi"("State(s) in (\"\")"=w371) -> ("States Out"=w370:string)  [unwired: 14 in]
        n165 = Unbundle By Name(w368) -> ("Particle Distribution Data.Concentration"=w364:dbl[][], "Particle Distribution Data.SMPS Sizes"=w363:dbl[], "Extinction ExtinctionUncertainity Size parameter and Number ofS sizes.Sizes"=w365:dbl[])
        n166 = call "Find and Shift SMPS sizes according to selected Peak Position.vi"("Sizes"=w365, "SMPS Sizes"=w363, "Concentration"=w364, "method"="method") -> ("Peak Position in the old data"=→"Peak Center":dbl[], "SMPS sizes"=w366:dbl[], "Shifted Concentration"=w360:dbl[][])  [unwired: 5 in]
        n167 = Transpose Matrix(1:w360) -> (0:→"yi out":dbl[][])
        n168 = for {
          tunnel: w360 -> [w378] mode=indexing
          tunnel: w366 -> [w377]
          tunnel: w364 -> [w376] mode=indexing
          tunnel: w363 -> [w375]
          n169 = Bundle("SMPS sizes"=w377, "Shifted Concentration"=w378) -> (w374:T21)  [unwired: 1 in]
          n170 = Bundle("SMPS Sizes"=w375, "Concentration"=w376) -> (w373:T20)  [unwired: 1 in]
          n171 = Build Array(w374, w373) -> (→"SMPS":T13)
        }
        n172 = Bundle By Name(cluster=w368, "Particle Distribution Data.Concentration"=w360, "Particle Distribution Data.SMPS Sizes"=w366) -> (w367:T17)
      }
      frame "Append Mie Curve" {
        # "Calculate\nThe correction\nfor tested n and k"
        n173 = call <vilib>:"Add State(s) to Queue__jki_lib_state_machine.vi"("State(s) in (\"\")"=w408) -> ("States Out"=w407:string)  [unwired: 14 in]
        n174 = disable-structure shown="Disabled" {
          frame Disabled {
            n175 = control-ref of="Real Part vs wavelength"() -> (w410:refnum<vi>)
            n176 = control-ref of="Imaginary Part vs wavelength"() -> (w409:refnum<vi>)
            n177 = property on="Property Node" class="XYGraph (strict)" props=["Cursor", "Cursor Y"](reference=w410) -> ()  [unwired: 1 in, 3 out]
            n178 = property on="Property Node" class="XYGraph (strict)" props=["Cursor", "Cursor Y"](reference=w409) -> ()  [unwired: 1 in, 3 out]
          }
          frame Enabled {
          }
        }
        n179 = Unbundle By Name(w405) -> ("Baes data type definition"=w381:T10, "Baes data type definition.Number ofSizes"=w391:dbl)  [unwired: 2 out]
        n180 = call "GetAbsorptionCrossSectionsFromLinearLineRegression.vi"("Extinction ExtinctionUncertainity Size parameter and Number ofS sizes 2"=w381, "refractive index, imaginary"="k", "refractive index, real"="n") -> ("Expected Extinction/Absorption Cross Section Uncer"=w379:dbl[], "Expected Extinction/Absorption Cross Section"=w380:dbl[])  [unwired: 1 out]
        n181 = property on="Corrected for multiple charge particles" class="XYGraph (strict)"() -> ("Value"=w402:cluster{"Size parameters":dbl[], dbl[]}[])  [unwired: 2 in, 2 out]
        n182 = call "CalculateExtinctionCorrectionsToDoublyChargeParticleContribution.vi"("refractive index, imaginary"="k", "refractive index, real"="n", "Extinction ExtinctionUncertainity Size parameter and Number ofS sizes"=w381) -> ("Expected Extinction Cross Section"=w390:sgl[])  [unwired: 1 out]
        n183 = call "CalculateAreaOfFirstPeakofSizeDistribution.vi"("Extinction ExtinctionUncertainity Size parameter and Number ofS sizes"=w381) -> ("Area of First peak"=w388:dbl[])
        n184 = Subtract(x=w380, y=w390) -> (x-y=w389:dbl[])
        n185 = call "PlotMieCurve.vi"("refractive index, imaginary"="k", "refractive index, real"="n", "Use Extinction Factor"=FALSE, "Extinction ExtinctionUncertainity Size parameter and Number ofS sizes"=w381) -> ("Mie Results In Size Parameters"=w392:sgl[], "Size parameters"=w404:dbl[], "Extinction Crosssections"=w403:dbl[])
        n186 = Divide(x=w389, y=w388) -> (x/y=w387:dbl[])
        n187 = Subtract(x=w387, y=w392) -> (x-y=w394:dbl[])
        n188 = Bundle("Size parameters"=w404, "Extinction Crosssections"=w403) -> (w401:T22)  [unwired: 1 in]
        n189 = Divide(x=w394, y=w379) -> (x/y=w393:dbl[])
        n190 = Build Array (concatenate)(w402, w401) -> (w399:T23)
        n191 = Square(x=w393) -> (x^2=w386:dbl[])
        n192 = Array Size(array=w399) -> (size(s)=w398:i32)
        n193 = Add Array Elements(numeric array=w386) -> (sum=w385:dbl)
        n194 = Subtract(x=w398, y=1) -> (x-y=w396:i32)
        n195 = Divide(x=w385, y=w391) -> (x/y=→"Residue":dbl)
        n196 = property on="Corrected for multiple charge particles" class="XYGraph (strict)"("Value"=w399, "Active Plot"=w396, "Plot.Plot Color"=u32 0) -> ()  [unwired: 2 in, 2 out]
      }
      frame "Load Files MC" {
        # "Loading files for Monte Carlo simulation for the purpoese of error analysis"
        n197 = call <vilib>:"Add State(s) to Queue__jki_lib_state_machine.vi"("State(s) in (\"\")"=w422) -> ("States Out"=w421:string)  [unwired: 14 in]
        n198 = local read "Extinction Cross Section File"() -> (w415:path)
        n199 = local read "Mutiple Charge Data File"() -> (w414:path)
        n200 = local read "Diameter Factor"() -> (w411:dbl)
        n201 = call "ReadParticleSizeSpectrum.vi"("file path"=w414, "Factor Size paramter"=w411) -> ("Particle Distribution Data"=w416:T8)  [unwired: 1 out]
        n202 = call "ReadBAESdataFromFileMCVersion.vi"("file path"=w415) -> ("Extinction ExtinctionUncertainity Size parameter and Number ofS sizes"=w417:T7, "FullExtinctionData"=w413:dbl[][], "NumberOfMeasurementsperSize"=w412:i32)
        n203 = Bundle By Name(cluster=w419, "Extinction ExtinctionUncertainity Size parameter and Number ofS sizes"=w417, "Particle Distribution Data"=w416, "Extinction Cross section Path"=w415, "Multiple charge correction file Path"=w414, "FullExtinctionData"=w413, "NumberOfMeasurementsperSize"=w412) -> (w418:T17)
      }
      frame "Retrieve RI" {
        n204 = stacked-sequence {
          tunnel: w426 -> [w459 _]
          tunnel: [w461 _] -> w425
          tunnel: w423 -> [w441 _]
          frame #0 {
            n205 = case shown="\"UseFactors\"" w441 {
              tunnel: [1.0 ("Extinction Factor") "Extinction Factor"] -> w444
              tunnel: [1.0 ("Diameter Factor") "Diameter Factor"] -> w443
              tunnel: [0.0 ("Diameter Offset") "Diameter Offset"] -> w442
              frame "DontUseFactors", Default {
              }
              frame "UseFactors" {
              }
            }
            n206 = property on="Diameters to fit" class="LstBox (strict)"() -> ("Item Symbols"=w440:i32[])  [unwired: 2 in, 2 out]
            n207 = for {
              tunnel: w440 -> [w470] mode=indexing
              tunnel: 38 ("Item Symbols") -> [w469]
              tunnel: [w468] -> w438 mode=indexing
              n208 = Equal?(x=w470, y=w469) -> (x = y?=w468:bool)
            }
            n209 = property on="Max Wavelength" class="CmbBox"() -> ("Value"=w452:string)  [unwired: 2 in, 2 out]
            n210 = property on="Min Wavelength" class="CmbBox"() -> ("Value"=w453:string)  [unwired: 2 in, 2 out]
            n211 = property on="Retrieve RI" class="Bool"("BoolText.Text"="Running...." ("Boolean Text.Text")) -> ()  [unwired: 2 in, 2 out]
            n212 = Unbundle By Name(w459) -> ("Extinction ExtinctionUncertainity Size parameter and Number ofS sizes"=w436:T7, "Particle Distribution Data"=w437:T8)
            n213 = Decimal String To Number(string=w453) -> (number=w451:i32)  [unwired: 2 in, 1 out]
            n214 = Decimal String To Number(string=w452) -> (number=w450:i32)  [unwired: 2 in, 1 out]
            n215 = local read "General Data for RI Retrieval VI"() -> (w446:T5)
            n216 = local read "ExtinctionOrAbsorptionOrScattering"() -> (w433:i8)
            n217 = control-ref of="Real Part vs wavelength"() -> (w467:refnum<vi>)
            n218 = control-ref of="Not Corrected for Multiple charge Best fit result"() -> (w465:refnum<vi>)
            n219 = control-ref of="Imaginary Part vs wavelength"() -> (w466:refnum<vi>)
            n220 = control-ref of="Normalized Residuals vs Size parameter"() -> (w464:refnum<vi>)
            n221 = control-ref of="Simplex"() -> (w445:refnum<vi>)
            n222 = local read "Approximate Errors"() -> (w457:bool)
            n223 = Bundle("Real Part vs wavelength"=w467, "Imaginary Part vs wavelength"=w466, "Normalized Residuals vs Size parameter"=w464, "Not Corrected for Multiple charge Best fit result"=w465, "Simplex"=w445) -> (w463:T24)  [unwired: 1 in]
            n224 = Bundle By Name(cluster=w446, "Min WaveLength Index"=w451, "Max WaveLength Index"=w450, "Extinction Factor"="Extinction Factor", "Size Parameter Factor"="Size Parameter Factor", "Size Paramter Offset"="Size Parameter Offset", "Extinction Factor"=w444, "Diameter Factor"=w443, "Diameter Offset"=w442, "ExtinctionOrAbsorptionOrScattering"=w433) -> (w462:T5)
            n225 = call "RestructureDataAccordingToSelectedSizes.vi"("Extinction Data input"=w436, "Particle Distribution input"=w437, "Sizes to Fit"=w438) -> ("Extinciton Data ouput"=w435:T7, "Particle Distribution output"=w434:T8)
            n226 = call "RIRetrieval.vi"("Minimization method"="Minimization method", "Extinction Measured Data"=w435, "Starting Guess -Real"="Starting Guess -Real", "Approximate Errors"=w457, "Graph Refs"=w463, "Particle Distribution Data"=w434, "Calculate Errors"="Calculate Errors", "Restrict to Positive Imaginary Part"="Restrict to Positive Imaginary Part", "Starting Guess - Imag"="Starting Guess - Imag", "General Data for RI Retrieval VI"=w462) -> ("RI results"=w460:T16, "All Input data in one Cluster"=w454:T10)  [unwired: 2 in, 2 out]
            n227 = Bundle By Name(cluster=w459, "RI results"=w460, "Baes data type definition"=w454, "Extinction ExtinctionUncertainity Size parameter and Number ofS sizes"=w435, "Particle Distribution Data"=w434) -> (w461:T17)
          }
          frame #1 {
            n228 = disable-structure shown="Disabled" {
              frame Disabled {
                n229 = One Button Dialog(message="RI retrieval finished successfully") -> ()  [unwired: 1 in, 1 out]
              }
              frame Enabled {
              }
            }
            n230 = property on="Retrieve RI" class="Bool"("BoolText.Text"="Retrieve RI" ("Boolean Text.Text")) -> ()  [unwired: 2 in, 2 out]
          }
        }
        n231 = call <vilib>:"Add State(s) to Queue__jki_lib_state_machine.vi"("State(s) in Front (\"\")"="Update Corrected multiple charge extinction graph" ("State(s) in Front (\"\")"), "State(s) in (\"\")"=w429) -> ("States Out"=w428:string)  [unwired: 13 in]
      }
      frame "Find Global Minimum" {
        w490 = 0 ("index (row)")
        n232 = local read "GlobalMinimumStruct"() -> (w492:T2)
        n233 = call-poly <vilib>:"Ramp Pattern.vi"("start"="k_start", "end"="k_finish", "samples"="k_samples") -> ("Ramp Pattern"=w494:dbl[])  [unwired: 7 in, 1 out]
        n234 = call-poly <vilib>:"Ramp Pattern.vi"("start"="n_start", "end"="n_finish", "samples"="n_samples") -> ("Ramp Pattern"=w495:dbl[])  [unwired: 7 in, 1 out]
        n235 = Index Array(array=w492, index (row)=w490, index (col)=w490) -> (element=w491:T1)
        n236 = for {
          tunnel: w495 -> [w519] mode=indexing
          tunnel: w494 -> [w520]
          shift-right: [w517] -> w480
          shift-left: T2 [] -> [w516]
          tunnel: w491 -> [w515]
          n237 = for {
            tunnel: w520 -> [w526] mode=indexing
            tunnel: w519 -> [w527]
            tunnel: [w523] -> w518 mode=indexing
            tunnel: w515 -> [w521]
            n238 = Bundle By Name(cluster=w521, "n"=w527, "ne"=0.0, "k"=w526, "ke"=0.0, "Residue"=0.0) -> (w523:T1)
          }
          n239 = Build Array (concatenate)(w516, w518) -> (w517:T2)
        }
        "GlobalMinimumStruct" <- w480
        n240 = for {
          tunnel: w505 -> [w535]
          tunnel: [w534] -> w504
          tunnel: w502 -> [w533]
          tunnel: w495 -> [w532] mode=indexing
          tunnel: w494 -> [w531]
          tunnel: [w529] -> w489
          tunnel: w480 -> [_]
          tunnel: [w528] -> w479
          i -> [w530]
          n241 = for {
            tunnel: w535 -> [w544]
            tunnel: [w543] -> w534
            tunnel: w533 -> [w542]
            tunnel: w532 -> [w541]
            tunnel: w531 -> [w540] mode=indexing
            tunnel: w530 -> [w539]
            tunnel: [w537] -> w529
            tunnel: [w536] -> w528
            i -> [w538]
            n242 = stacked-sequence {
              tunnel: w544 -> [w601 _]
              tunnel: [w602 _] -> w543
              tunnel: w542 -> [w589 _]
              tunnel: w541 -> [w573 _]
              tunnel: w540 -> [w572 _]
              tunnel: w539 -> [w570 _]
              tunnel: w538 -> [w571 _]
              tunnel: [w546 _] -> w537
              tunnel: [w545 _] -> w536
              frame #0 {
                w551 = dbl[] []
                n243 = property on="Diameters to fit" class="LstBox (strict)"() -> ("Item Symbols"=w588:i32[])  [unwired: 2 in, 2 out]
                n244 = case shown="\"UseFactors\"" w589 {
                  tunnel: [1.0 ("Extinction Factor") w634] -> w592
                  tunnel: [1.0 ("Diameter Factor") w633] -> w591
                  tunnel: [0.0 ("Diameter Offset") w632] -> w590
                  frame "DontUseFactors", Default {
                  }
                  frame "UseFactors" {
                    n245 = local read "Extinction Factor"() -> (w634:dbl)
                    n246 = local read "Diameter Factor"() -> (w633:dbl)
                    n247 = local read "Diameter Offset"() -> (w632:dbl)
                  }
                }
                n248 = for {
                  tunnel: w588 -> [w628] mode=indexing
                  tunnel: 38 ("Item Symbols") -> [w627]
                  tunnel: [w626] -> w586 mode=indexing
                  n249 = Equal?(x=w628, y=w627) -> (x = y?=w626:bool)
                }
                n250 = property on="Max Wavelength" class="CmbBox"() -> ("Value"=w597:string)  [unwired: 2 in, 2 out]
                n251 = property on="Min Wavelength" class="CmbBox"() -> ("Value"=w598:string)  [unwired: 2 in, 2 out]
                n252 = property on="Retrieve RI" class="Bool"("BoolText.Text"="Running...." ("Boolean Text.Text")) -> ()  [unwired: 2 in, 2 out]
                n253 = Unbundle By Name(w601) -> ("Extinction ExtinctionUncertainity Size parameter and Number ofS sizes"=w584:T7, "Particle Distribution Data"=w585:T8)
                n254 = Decimal String To Number(string=w598) -> (number=w596:i32)  [unwired: 2 in, 1 out]
                n255 = Decimal String To Number(string=w597) -> (number=w595:i32)  [unwired: 2 in, 1 out]
                n256 = local read "Size Parameter Factor"() -> (w575:bool)
                n257 = local read "Size Parameter Offset"() -> (w574:bool)
                n258 = local read "ExtinctionOrAbsorptionOrScattering"() -> (w581:i8)
                n259 = local read "Extinction Factor"() -> (w576:bool)
                n260 = local read "General Data for RI Retrieval VI"() -> (w594:T5)
                n261 = local read "Restrict to Positive Imaginary Part"() -> (w577:bool)
                n262 = control-ref of="Real Part vs wavelength"() -> (w608:refnum<vi>)
                n263 = control-ref of="Not Corrected for Multiple charge Best fit result"() -> (w606:refnum<vi>)
                n264 = control-ref of="Imaginary Part vs wavelength"() -> (w607:refnum<vi>)
                n265 = control-ref of="Normalized Residuals vs Size parameter"() -> (w605:refnum<vi>)
                n266 = control-ref of="Simplex"() -> (w593:refnum<vi>)
                n267 = local read "Minimization method"() -> (w579:u16)
                n268 = local read "Calculate Errors"() -> (w578:bool)
                n269 = local read "Approximate Errors"() -> (w600:bool)
                n270 = Bundle("Real Part vs wavelength"=w608, "Imaginary Part vs wavelength"=w607, "Normalized Residuals vs Size parameter"=w605, "Not Corrected for Multiple charge Best fit result"=w606, "Simplex"=w593) -> (w604:T24)  [unwired: 1 in]
                n271 = Bundle By Name(cluster=w594, "Min WaveLength Index"=w596, "Max WaveLength Index"=w595, "Extinction Factor"=w576, "Size Parameter Factor"=w575, "Size Paramter Offset"=w574, "Extinction Factor"=w592, "Diameter Factor"=w591, "Diameter Offset"=w590, "ExtinctionOrAbsorptionOrScattering"=w581) -> (w603:T5)
                n272 = call "RestructureDataAccordingToSelectedSizes.vi"("Extinction Data input"=w584, "Particle Distribution input"=w585, "Sizes to Fit"=w586) -> ("Extinciton Data ouput"=w583:T7, "Particle Distribution output"=w582:T8)
                n273 = call "RIRetrieval.vi"("Minimization method"=w579, "Extinction Measured Data"=w583, "Starting Guess -Real"=w573, "Approximate Errors"=w600, "Graph Refs"=w604, "Particle Distribution Data"=w582, "Calculate Errors"=w578, "Restrict to Positive Imaginary Part"=w577, "Starting Guess - Imag"=w572, "General Data for RI Retrieval VI"=w603) -> ("RI results"=w569:T16, "All Input data in one Cluster"=w599:T10)  [unwired: 2 in, 2 out]
                n274 = Bundle By Name(cluster=w601, "RI results"=w569, "Baes data type definition"=w599, "Extinction ExtinctionUncertainity Size parameter and Number ofS sizes"=w583, "Particle Distribution Data"=w582) -> (w602:T17)
                n275 = local read "GlobalMinimumStruct"() -> (w550:T2)
                n276 = Unbundle By Name(w569) -> ("Real RI"=w568:dbl[], "Std Real RI"=w562:dbl[], "Imaginary RI"=w561:dbl[], "Std Imaginary RI"=w560:dbl[], "Residue"=w556:dbl[])
                n277 = Index Array(array=w550, index (row)=0, index (col)=0 ("disabled index (col)")) -> (element=w547:T1)
                n278 = Index Array(array=w556, index=0) -> (element=w554:dbl)
                n279 = Index Array(array=w562, index=0) -> (element=w559:dbl)
                n280 = Index Array(array=w561, index=0) -> (element=w558:dbl)
                n281 = Index Array(array=w560, index=0) -> (element=w557:dbl)
                n282 = Index Array(array=w568, index=0) -> (element=w566:dbl)
                n283 = in-place {
                  in-place-border: w566 -> [w625]
                  in-place-border: w559 -> [w624]
                  in-place-border: w558 -> [w623]
                  in-place-border: w557 -> [w622]
                  in-place-border: w554 -> [w621]
                  in-place-border: w547 -> [w619]
                  n284 = in-place-array #1(w550, w570, w571) -> ()  [unwired: 1 out]
                  n285 = Bundle By Name(cluster=w619, "n"=w625, "ne"=w624, "k"=w623, "ke"=w622, "Residue"=w621) -> (w620:T1)
                  n286 = in-place-array #1(w620) -> (w545:T2)  [unwired: 2 out]
                }
                n287 = for {
                  tunnel: w545 -> [w615] mode=indexing
                  shift-right: [w613] -> w552
                  shift-left: w551 -> [w612]
                  shift-right: [w610] -> w553
                  shift-left: w551 -> [w609]
                  n288 = for {
                    tunnel: w615 -> [w618] mode=indexing
                    tunnel: [w617] -> w614 mode=indexing
                    tunnel: [w616] -> w611 mode=indexing
                    n289 = Unbundle By Name(w618) -> ("n"=w617:dbl, "k"=w616:dbl)
                  }
                  n290 = Build Array (concatenate)(w612, w614) -> (w613:dbl[])
                  n291 = Build Array (concatenate)(w609, w611) -> (w610:dbl[])
                }
                n292 = local write "GlobalMinimumStruct"(w545) -> ()
                n293 = Bundle(w552, w553) -> (w546:cluster{dbl[], dbl[]})  [unwired: 1 in]
                "n-k matrix" <- w546
              }
              frame #1 {
                n294 = disable-structure shown="Disabled" {
                  frame Disabled {
                    n295 = One Button Dialog(message="RI retrieval finished successfully") -> ()  [unwired: 1 in, 1 out]
                  }
                  frame Enabled {
                  }
                }
                n296 = property on="Retrieve RI" class="Bool"("BoolText.Text"="Retrieve RI" ("Boolean Text.Text")) -> ()  [unwired: 2 in, 2 out]
              }
            }
          }
        }
        n297 = for {
          tunnel: w479 -> [w512] mode=indexing
          shift-right: [w509] -> w487
          shift-left: dbl[][] [] -> [w510]
          tunnel: w489 -> [_]
          n298 = for {
            tunnel: w512 -> [w514] mode=indexing
            tunnel: [w513] -> w511 mode=indexing
            n299 = Unbundle By Name(w514) -> ("Residue"=w513:dbl)
          }
          n300 = Build Array (concatenate)(w510, w511) -> (w509:dbl[][])
        }
        "Array" <- w487
        n301 = Array Max & Min(array=w487) -> (min index (indices)=w481:i32[])  [unwired: 3 out]
        n302 = Index Array(array=w481, index #1=0 ("index"), index #2=1 ("index")) -> (element #1=w484:i32, element #2=w483:i32)
        n303 = Index Array(array=w479, index (row)=w484, index (col)=w483) -> (element=→"Global Min":T1)
        n304 = call <vilib>:"Add State(s) to Queue__jki_lib_state_machine.vi"("State(s) in Front (\"\")"="Update Corrected multiple charge extinction graph" ("State(s) in Front (\"\")"), "State(s) in (\"\")"=w508) -> ("States Out"=w507:string)  [unwired: 13 in]
      }
      frame "Find Extinction and Size Parameter Factor" {
        n305 = stacked-sequence {
          tunnel: w639 -> [w676 _]
          tunnel: [w678 _] -> w638
          frame #0 {
            # "Real"
            n306 = property on="Max Wavelength" class="CmbBox"() -> ("Value"=w673:string)  [unwired: 2 in, 2 out]
            n307 = property on="Min Wavelength" class="CmbBox"() -> ("Value"=w674:string)  [unwired: 2 in, 2 out]
            n308 = local read "General Data for RI Retrieval VI"() -> (w645:T5)
            n309 = local read "Size Parameter Factor"() -> (w648:bool)
            n310 = local read "Size Parameter Offset"() -> (w647:bool)
            n311 = Decimal String To Number(string=w674) -> (number=w672:i32)  [unwired: 2 in, 1 out]
            n312 = Decimal String To Number(string=w673) -> (number=w671:i32)  [unwired: 2 in, 1 out]
            n313 = control-ref of="Simplex"() -> (w644:refnum<vi>)
            n314 = local read "Extinction Factor"() -> (w649:bool)
            n315 = control-ref of="Real Part vs wavelength"() -> (w682:refnum<vi>)
            n316 = control-ref of="Not Corrected for Multiple charge Best fit result"() -> (w680:refnum<vi>)
            n317 = control-ref of="Imaginary Part vs wavelength"() -> (w681:refnum<vi>)
            n318 = control-ref of="Normalized Residuals vs Size parameter"() -> (w679:refnum<vi>)
            n319 = Unbundle By Name(w676) -> ("Extinction ExtinctionUncertainity Size parameter and Number ofS sizes"=w669:T7, "Particle Distribution Data"=w667:T8)
            n320 = Bundle By Name(cluster=w645, "Min WaveLength Index"=w672, "Max WaveLength Index"=w671, "Extinction Factor"=w649, "Size Parameter Factor"=w648, "Size Paramter Offset"=w647, "ExtinctionOrAbsorptionOrScattering"="ExtinctionOrAbsorptionOrScattering") -> (w646:T5)
            n321 = Bundle(cluster="Graph Refs", "Real Part vs wavelength"=w682, "Imaginary Part vs wavelength"=w681, "Normalized Residuals vs Size parameter"=w679, "Not Corrected for Multiple charge particles"=w680, "Simplex 2"=w644) -> (w662:T6)
            n322 = local read "Restrict to Positive Imaginary Part"() -> (w665:bool)
            n323 = local read "Minimization method"() -> (w668:u16)
            n324 = local read "Approximate Errors"() -> (w670:bool)
            n325 = local read "Calculate Errors"() -> (w666:bool)
            n326 = Bundle(cluster="Data for RIRetrieval VI", "Approximate Errors"=w670, "Extinction ExtinctionUncertainity Size parameter and Number ofS sizes"=w669, "Minimization method"=w668, "Graph Ref"=w662, "Particle Distribution Data"=w667, "Calculate Errors"=w666, "Restrict to Positive Imaginary Part"=w665, "MinMaxWavelength"=w646) -> (w655:T9)
            n327 = call "RIRetrieval.vi"("Minimization method"=w668, "Extinction Measured Data"=w669, "Approximate Errors"=w670, "Graph Refs"=w662, "Particle Distribution Data"=w667, "Calculate Errors"=w666, "Restrict to Positive Imaginary Part"=w665, "General Data for RI Retrieval VI"=w646) -> ("RI results"=w677:T16, "All Input data in one Cluster"=w675:T10)  [unwired: 4 in, 2 out]
            n328 = Bundle By Name(cluster=w676, "RI results"=w677, "Baes data type definition"=w675) -> (w678:T17)
            n329 = To Variant(anything=w655) -> (Variant=w659:variant)
            n330 = vi-ref "FindExtinctionAndSizeParameterFactors.vi"() -> (w658:refnum<vi>)
            n331 = Build Array(5.0 ("element"), 5.0 ("element")) -> (w661:dbl[])
            n332 = call-poly <vilib>:"Unconstrained Optimization.vi"("function data"=w659, "objective function"=w658, "stopping criteria"=T14 {"function tolerance"=0.01, "parameter tolerance"=0.05, "max iterations"=10, "max function calls"=1000, "gradient tolerance"=1000000.0, "max time (sec)"=-1.0}, "start"=w661) -> ("minimum"=w651:dbl[])  [unwired: 4 in, 3 out]
            n333 = Index Array(array=w651, index=0) -> (element=→"Minimized Extinction Factor":dbl)
            n334 = Index Array(array=w651, index=0) -> (element=→"Minimized Size Parameter Factor":dbl)
          }
          frame #1 {
            n335 = One Button Dialog(message="RI retrieval finished successfully") -> ()  [unwired: 1 in, 1 out]
          }
        }
        n336 = call <vilib>:"Add State(s) to Queue__jki_lib_state_machine.vi"("State(s) in Front (\"\")"="Update Corrected multiple charge extinction graph" ("State(s) in Front (\"\")"), "State(s) in (\"\")"=w642) -> ("States Out"=w641:string)  [unwired: 13 in]
      }
      frame "Find Extinction Factor" {
        n337 = stacked-sequence {
          tunnel: w686 -> [w695 _]
          tunnel: [w724 _] -> w685
          frame #0 {
            n338 = Subtract(x="Diameter FO Finish", y="Diameter FO start") -> (x-y=w719:dbl)
            n339 = Divide(x=w719, y="Diameter FO Interval") -> (x/y=w717:dbl)
            n340 = Round To Nearest(number=w717) -> (nearest integer value=w716:dbl)
            n341 = Increment(x=w716) -> (x+1=w715:dbl)
            n342 = call-poly <vilib>:"Ramp Pattern.vi"("start"="Diameter FO start", "end"="Diameter FO Finish", "samples"=w715) -> ("Ramp Pattern"=w699:dbl[])  [unwired: 7 in, 1 out]
            n343 = Tick Count (ms)() -> (millisecond timer value=w698:u32)
            n344 = property on="Diameters to fit" class="LstBox (strict)"() -> ("Item Symbols"=w697:i32[])  [unwired: 2 in, 2 out]
            n345 = for {
              tunnel: w697 -> [w727] mode=indexing
              tunnel: 38 ("Item Symbols") -> [w726]
              tunnel: [w725] -> w692 mode=indexing
              n346 = Equal?(x=w727, y=w726) -> (x = y?=w725:bool)
            }
            n347 = Unbundle By Name(w695) -> ("Particle Distribution Data"=w694:T8, "Extinction ExtinctionUncertainity Size parameter and Number ofS sizes"=w693:T7)
            n348 = call "RestructureDataAccordingToSelectedSizes.vi"("Extinction Data input"=w693, "Particle Distribution input"=w694, "Sizes to Fit"=w692) -> ("Extinciton Data ouput"=w690:T7, "Particle Distribution output"=w691:T8)
            n349 = for {
              tunnel: [w757] -> w723
              tunnel: w695 -> [w756]
              tunnel: [w755] -> w722
              tunnel: w699 -> [w748] mode=indexing
              tunnel: [w747] -> w702 mode=indexing
              tunnel: [w745] -> _
              tunnel: ["Extinction Factor Start"] -> _
              tunnel: [w736] -> w700
              tunnel: w699 -> [w737]
              tunnel: w698 -> [w735]
              tunnel: w691 -> [w729]
              tunnel: w690 -> [w728]
              i -> [w733]
              n350 = Subtract(x="Extinction Factor Finish", y="Extinction Factor Start") -> (x-y=w742:dbl)
              n351 = Divide(x=w742, y="Extinction Factor Interval") -> (x/y=w740:dbl)
              n352 = Array Size(array=w737) -> (size(s)=w732:i32)
              n353 = Round To Nearest(number=w740) -> (nearest integer value=w739:dbl)
              n354 = Subtract(x="Extinction Factor Finish", y="Extinction Factor Start") -> (x-y=w746:dbl)
              n355 = Increment(x=w739) -> (x+1=w738:dbl)
              n356 = Divide(x=w746, y=w738) -> (x/y=w745:dbl)
              n357 = call-poly <vilib>:"Ramp Pattern.vi"("start"="Extinction Factor Start", "end"="Extinction Factor Finish", "samples"=w738) -> ("Ramp Pattern"=w736:dbl[])  [unwired: 7 in, 1 out]
              n358 = Array Size(array=w736) -> (size(s)=w730:i32)
              n359 = control-ref of="Progress bar for Extinction search"() -> (w734:refnum<vi>)
              n360 = Multiply(x=w732, y=w730) -> (x*y=w731:i32)
              n361 = for {
                tunnel: [w792] -> w757
                tunnel: w756 -> [_]
                tunnel: [w807] -> w755
                tunnel: w736 -> [w793] mode=indexing
                tunnel: [w788] -> w754 mode=indexing
                tunnel: [w787] -> w753 mode=indexing
                tunnel: [w786] -> w747 mode=indexing
                tunnel: w748 -> [w780]
                shift-right: [w764] -> _
                shift-left: w735 -> [w772]
                tunnel: w733 -> [_]
                tunnel: w734 -> [w770]
                tunnel: w733 -> [w767]
                tunnel: w731 -> [w763]
                tunnel: w730 -> [w760]
                tunnel: w729 -> [w759]
                tunnel: w728 -> [w758]
                i -> [w771]
                n362 = local read "Size Parameter Factor"() -> (w797:bool)
                n363 = local read "Size Parameter Offset"() -> (w796:bool)
                n364 = local read "Extinction Factor"() -> (w798:bool)
                n365 = property on="Max Wavelength" class="CmbBox"() -> ("Value"=w805:string)  [unwired: 2 in, 2 out]
                n366 = property on="Min Wavelength" class="CmbBox"() -> ("Value"=w806:string)  [unwired: 2 in, 2 out]
                n367 = Decimal String To Number(string=w806) -> (number=w804:i32)  [unwired: 2 in, 1 out]
                n368 = Decimal String To Number(string=w805) -> (number=w803:i32)  [unwired: 2 in, 1 out]
                n369 = Select(t=w780, s="Diameter Factor or Offset", f=0.0) -> (s? t:f=w782:dbl)
                n370 = Select(t=1.0 ("Diameter Factor"), s="Diameter Factor or Offset", f=w780) -> (s? t:f=w778:dbl)
                n371 = Tick Count (ms)() -> (millisecond timer value=w764:u32)
                n372 = Bundle By Name(cluster="General Data for RI Retrieval VI", "Min WaveLength Index"=w804, "Max WaveLength Index"=w803, "Extinction Factor"=w798, "Size Parameter Factor"=w797, "Size Paramter Offset"=w796, "Extinction Factor"=w793, "Diameter Offset"=w782, "Diameter Factor"=w778) -> (w795:T5)
                n373 = Subtract(x=w764, y=w772) -> (x-y=w773:u32)
                n374 = Multiply(x=w760, y=w767) -> (x*y=w766:i32)
                n375 = control-ref of="Real Part vs wavelength"() -> (w811:refnum<vi>)
                n376 = control-ref of="Not Corrected for Multiple charge Best fit result"() -> (w809:refnum<vi>)
                n377 = control-ref of="Imaginary Part vs wavelength"() -> (w810:refnum<vi>)
                n378 = control-ref of="Normalized Residuals vs Size parameter"() -> (w808:refnum<vi>)
                n379 = control-ref of="Simplex"() -> (w777:refnum<vi>)
                n380 = Increment(x=w771) -> (x+1=w765:i32)
                n381 = Add(x=w766, y=w765) -> (x+y=w762:i32)
                n382 = Subtract(x=w763, y=w762) -> (x-y=w761:i32)
                n383 = property class="Slide (strict)"(reference=w770, "Value"=w762) -> ()  [unwired: 1 in, 2 out]
                n384 = Bundle(cluster="Graph Refs 2", "Real Part vs wavelength"=w811, "Imaginary Part vs wavelength"=w810, "Normalized Residuals vs Size parameter"=w808, "Not Corrected for Multiple charge particles"=w809, "Simplex 2"=w777) -> (w799:T6)
                n385 = local read "Restrict to Positive Imaginary Part"() -> (w801:bool)
                n386 = Divide(x=w773, y=u32 60000) -> (x/y=w769:dbl)
                n387 = Multiply(x=w769, y=w761) -> (x*y=→"Time Left (min)":dbl)
                n388 = local read "Minimization method"() -> (w802:u16)
                n389 = local read "Max Wavelength"() -> (w785:string)
                n390 = call "RIRetrieval.vi"("Minimization method"=w802, "Extinction Measured Data"=w758, "Approximate Errors"=FALSE, "Graph Refs"=w799, "Particle Distribution Data"=w759, "Calculate Errors"=FALSE, "Restrict to Positive Imaginary Part"=w801, "General Data for RI Retrieval VI"=w795) -> ("RI results"=w792:T16, "All Input data in one Cluster"=w807:T10)  [unwired: 4 in, 2 out]
                n391 = Unbundle By Name(w792) -> ("Real RI"=w791:dbl[], "Imaginary RI"=w790:dbl[], "Residue"=w789:dbl[])
                n392 = Decimal String To Number(string=w785) -> (number=w784:i32)  [unwired: 2 in, 1 out]
                n393 = Index Array(array=w791, index=w784) -> (element=w788:dbl)
                n394 = Index Array(array=w790, index=w784) -> (element=w787:dbl)
                n395 = Index Array(array=w789, index=w784) -> (element=w786:dbl)
              }
              n396 = property class="Slide (strict)"(reference=w734, "Scale.Maximum"=w731) -> ()  [unwired: 1 in, 2 out]
              n397 = Bundle("Ramp Pattern"=w736, w754) -> (w752:cluster{"Ramp Pattern":dbl[], dbl[]})  [unwired: 1 in]
              n398 = Bundle("Ramp Pattern"=w736, w753) -> (w751:cluster{"Ramp Pattern":dbl[], dbl[]})  [unwired: 1 in]
              n399 = Bundle("Ramp Pattern"=w736, w747) -> (w750:cluster{"Ramp Pattern":dbl[], dbl[]})  [unwired: 1 in]
              n400 = Build Array(w752, w751, w750) -> (→"Extinction Factor Results":cluster{"Ramp Pattern":dbl[], dbl[]}[])
            }
            "Residue Graph Matrix" <- w702
            n401 = Bundle By Name(cluster=w695, "RI results"=w723, "Baes data type definition"=w722) -> (w724:T17)
            n402 = Array Max & Min(array=w702) -> (min index (indices)=w714:i32[])  [unwired: 3 out]
            n403 = call <vilib>:"create_plot_surface.vi"("z matrix"=w702, "y vector"=w700, "x vector"=w699) -> ("plots out"=→"3D Graph":refnum<class "Base Datatype.lvclass">[])  [unwired: 2 in, 6 out]
            n404 = local read "Diameter Factor or Offset"() -> (w706:bool)
            n405 = Index Array(array=w714, index #1=0 ("index"), index #2=1 ("index")) -> (element #1=w710:i32, element #2=w711:i32)
            n406 = Index Array(array=w700, index=w711) -> (element=w709:dbl)
            n407 = Index Array(array=w699, index=w710) -> (element=w705:dbl)
            n408 = local write "Extinction Factor"(w709) -> ()
            n409 = Select(t=1.0 ("Diameter Factor"), s=w706, f=w705) -> (s? t:f=w703:dbl)
            n410 = Select(t=w705, s=w706, f=0.0) -> (s? t:f=w704:dbl)
            n411 = local write "Diameter Factor"(w703) -> ()
            n412 = local write "Diameter Offset"(w704) -> ()
          }
          frame #1 {
          }
        }
        n413 = call <vilib>:"Add State(s) to Queue__jki_lib_state_machine.vi"("State(s) in Front (\"\")"="Load Files >> Dont Initialize Sizes\nRetrieve RI >> UseFactors\nUpdate Corrected multiple charge extinction graph" ("State(s) in Front (\"\")"), "State(s) in (\"\")"=w689) -> ("States Out"=w688:string)  [unwired: 13 in]
      }
      frame "Save RI to file" {
        n414 = stacked-sequence {
          tunnel: w813 -> [w866 _]
          frame #0 {
            n415 = local read "Approximate Errors"() -> (w831:bool)
            n416 = property on="Max Wavelength" class="CmbBox"() -> ("Value"=w842:string)  [unwired: 2 in, 2 out]
            n417 = property on="Min Wavelength" class="CmbBox"() -> ("Value"=w843:string)  [unwired: 2 in, 2 out]
            n418 = Unbundle By Name(w866) -> ("Extinction Cross section Path"=w874:path, "RI results.Wavelength"=w875:dbl[], "RI results.Real RI"=w876:dbl[], "RI results.Std Real RI"=w845:dbl[], "RI results.Imaginary RI"=w846:dbl[], "RI results.Std Imaginary RI"=w844:dbl[], "RI results.Residue"=w819:dbl[], "RI results.Extinction Factor"=w818:dbl[], "RI results.Diameter Factor"=w817:dbl[], "RI results.Diameter Offset"=w816:dbl[])
            n419 = local read "Calculate Errors"() -> (w832:bool)
            n420 = Decimal String To Number(string=w842) -> (number=w841:i32)  [unwired: 2 in, 1 out]
            n421 = Decimal String To Number(string=w843) -> (number=w821:i32)  [unwired: 2 in, 1 out]
            n422 = Unbundle By Name(w866) -> ("Extinction ExtinctionUncertainity Size parameter and Number ofS sizes"=w865:T7, "Particle Distribution Data"=w864:T8, "RI results"=w863:T16)
            n423 = Build Array(w875, w876, w846, w845, w844, w819, w818, w817, w816) -> (w873:dbl[][])
            n424 = Select(t="+ApproxError" ("name or relative path"), s=w831, f="-ApproxError" ("name or relative path")) -> (s? t:f=w830:string)
            n425 = Subtract(x=w841, y=w821) -> (x-y=w871:i32)
            n426 = call <vilib>:"Get File Extension.vi"("file"=w874) -> ("filename without extension"=w824:string)  [unwired: 7 in, 3 out]
            n427 = local read "Restrict to Positive Imaginary Part"() -> (w837:bool)
            n428 = Concatenate Strings(w824, w830) -> (w829:string)
            n429 = call "PrepareExtinctionCrossSectionToFile.vi"("Extinction ExtinctionUncertainity Size parameter and Number ofS sizes"=w865, "RI results"=w863, "Particle Distribution Data"=w864, "Min Wavelength index"=w821, "Max Wavelength index"=w841) -> ("Extinction"=w861:dbl[][], "CorrectedExtinction"=w862:dbl[][], "Sigma_diameter_string"=w851:string[])
            n430 = Transpose 2D Array(2D array=w873) -> (transposed array=w872:dbl[][])
            n431 = Increment(x=w871) -> (x+1=w820:i32)
            n432 = Select(t="+Error" ("name or relative path"), s=w832, f="-Error" ("name or relative path")) -> (s? t:f=w828:string)
            n433 = Concatenate Strings(w829, w828) -> (w827:string)
            n434 = Select(t="+Restricted" ("name or relative path"), s=w837, f="-Restricted" ("name or relative path")) -> (s? t:f=w826:string)
            n435 = Array Subset(array=w872, index (row)=w821, length (row)=w820) -> (w870:dbl[][])  [unwired: 2 in]
            n436 = Array Subset(array=w861, index (row)=w821, length (row)=w820) -> (w860:dbl[][])  [unwired: 2 in]
            n437 = Array Subset(array=w862, index (row)=w821, length (row)=w820) -> (w859:dbl[][])  [unwired: 2 in]
            n438 = Concatenate Strings(w827, w826) -> (w825:string)
            n439 = Transpose 2D Array(2D array=w860) -> (transposed array=w858:dbl[][])
            n440 = Transpose 2D Array(2D array=w859) -> (transposed array=w857:dbl[][])
            n441 = Number To Fractional String(number=w870, precision (6)=i16 3) -> (F-format string=w855:string[][])  [unwired: 2 in]
            n442 = Build Array (concatenate)(w858, w857) -> (w856:dbl[][])
            n443 = Concatenate Strings(w825, "_RIresult.txt" ("name or relative path")) -> (w877:string)
            n444 = Strip Path(path=w874) -> (stripped path=w878:path)  [unwired: 1 out]
            n445 = Number To Engineering String(4:w856) -> (0:w848:string[][])  [unwired: 3 in]
            n446 = Build Path(base path=w878, name or relative path=w877) -> (appended path=w867:path)
            "Saved RI to this filename and path" <- w867
            n447 = Transpose 2D Array(2D array=w848) -> (transposed array=w847:string[][])
            n448 = Build Array (concatenate)(string[] ["Wavelength (nm)", "Real Part", "Imaginary Part", "Conf Real Part", "Conf Imaginary part", "Residue (MDBF)", "Extinction Factor", "Diameter Factor", "Diameter Offset (nm)"] ("column headers"), w855) -> (w852:string[][])
            n449 = Build Array (concatenate)(w851, w847) -> (w850:string[][])
            n450 = Transpose 2D Array(2D array=w852) -> (transposed array=w854:string[][])
            n451 = Transpose 2D Array(2D array=w850) -> (transposed array=w849:string[][])
            n452 = Build Array (concatenate)(w854, w849) -> (w823:string[][])
            n453 = Transpose 2D Array(2D array=w823) -> (transposed array=w822:string[][])
            n454 = call-poly <vilib>:"Write To Spreadsheet File.vi"("transpose? (no:F)"=FALSE, "2D data"=w822, "file path (dialog if empty)"=w867) -> ()  [unwired: 5 in, 1 out]
          }
          frame #1 {
            n455 = One Button Dialog(message="File save was completed successfully") -> ()  [unwired: 1 in, 1 out]
          }
        }
        n456 = call <vilib>:"Add State(s) to Queue__jki_lib_state_machine.vi"("State(s) in (\"\")"=w815) -> ("States Out"=w814:string)  [unwired: 14 in]
      }
      frame "Save RI to File Expanded Edition" {
        n457 = call <vilib>:"Add State(s) to Queue__jki_lib_state_machine.vi"("State(s) in (\"\")"=w883) -> ("States Out"=w882:string)  [unwired: 14 in]
        n458 = stacked-sequence {
          tunnel: w881 -> [w940 _]
          frame #0 {
            # "This inlcudes the number of sizes and the reduced chi^2 measurement for each wavelength"
            n459 = Unbundle By Name(w940) -> ("Extinction Cross section Path"=w948:path, "RI results.Wavelength"=w949:dbl[], "RI results.Real RI"=w950:dbl[], "RI results.Std Real RI"=w918:dbl[], "RI results.Imaginary RI"=w919:dbl[], "RI results.Std Imaginary RI"=w917:dbl[], "RI results.Residue"=w889:dbl[], "Extinction ExtinctionUncertainity Size parameter and Number ofS sizes.Number ofSizes"=w888:dbl)
            n460 = Build Array(w949, w950, w919, w918, w917, w889) -> (w947:dbl[][])
            n461 = Transpose 2D Array(2D array=w947) -> (transposed array=w946:dbl[][])
            n462 = property on="Min Wavelength" class="CmbBox"() -> ("Value"=w916:string)  [unwired: 2 in, 2 out]
            n463 = property on="Max Wavelength" class="CmbBox"() -> ("Value"=w915:string)  [unwired: 2 in, 2 out]
            n464 = Decimal String To Number(string=w915) -> (number=w913:i32)  [unwired: 2 in, 1 out]
            n465 = Decimal String To Number(string=w916) -> (number=w914:i32)  [unwired: 2 in, 1 out]
            n466 = Unbundle By Name(w940) -> ("Extinction ExtinctionUncertainity Size parameter and Number ofS sizes"=w939:T7, "Particle Distribution Data"=w938:T8, "RI results"=w937:T16)
            n467 = Subtract(x=w913, y=w914) -> (x-y=w945:i32)
            n468 = call "PrepareExtinctionCrossSectionToFile.vi"("Extinction ExtinctionUncertainity Size parameter and Number ofS sizes"=w939, "RI results"=w937, "Particle Distribution Data"=w938, "Min Wavelength index"=w914, "Max Wavelength index"=w913) -> ("Extinction"=w934:dbl[][], "CorrectedExtinction"=w936:dbl[][], "Sigma_diameter_string"=w924:string[])
            n469 = Increment(x=w945) -> (x+1=w935:i32)
            n470 = Array Subset(array=w946, index (row)=w914, length (row)=w935) -> (w944:dbl[][])  [unwired: 2 in]
            n471 = Array Subset(array=w934, index (row)=w914, length (row)=w935) -> (w933:dbl[][])  [unwired: 2 in]
            n472 = Array Subset(array=w936, index (row)=w914, length (row)=w935) -> (w932:dbl[][])  [unwired: 2 in]
            n473 = Transpose 2D Array(2D array=w933) -> (transposed array=w931:dbl[][])
            n474 = Transpose 2D Array(2D array=w932) -> (transposed array=w930:dbl[][])
            n475 = Number To Fractional String(number=w944, precision (6)=i16 3) -> (F-format string=w928:string[][])  [unwired: 2 in]
            n476 = Build Array (concatenate)(w931, w930) -> (w929:dbl[][])
            n477 = Number To Engineering String(4:w929) -> (0:w921:string[][])  [unwired: 3 in]
            n478 = Transpose 2D Array(2D array=w921) -> (transposed array=w920:string[][])
            n479 = local read "Calculate Errors"() -> (w904:bool)
            n480 = Build Array (concatenate)(string[] ["Wavelength (nm)", "Real Part", "Imaginary Part", "Conf Real Part", "Conf Imaginary part", "Eta (reduced Chi^2)"] ("column headers"), w928) -> (w925:string[][])
            n481 = Build Array (concatenate)(w924, w920) -> (w923:string[][])
            n482 = local read "Approximate Errors"() -> (w903:bool)
            n483 = Transpose 2D Array(2D array=w925) -> (transposed array=w927:string[][])
            n484 = Transpose 2D Array(2D array=w923) -> (transposed array=w922:string[][])
            n485 = local read "Restrict to Positive Imaginary Part"() -> (w909:bool)
            n486 = Select(t="+ApproxError" ("name or relative path"), s=w903, f="-ApproxError" ("name or relative path")) -> (s? t:f=w902:string)
            n487 = Build Array (concatenate)(w927, w922) -> (w891:string[][])
            n488 = Select(t="+Error" ("name or relative path"), s=w904, f="-Error" ("name or relative path")) -> (s? t:f=w900:string)
            n489 = call <vilib>:"Get File Extension.vi"("file"=w948) -> ("filename without extension"=w887:string)  [unwired: 7 in, 3 out]
            n490 = Number To Decimal String(number=w888) -> (decimal integer string=w886:string)  [unwired: 1 in]
            n491 = Concatenate Strings(w887, w902) -> (w901:string)
            n492 = Array Size(array=w891) -> (size(s)=w896:i32[])
            n493 = Concatenate Strings(w887, "_" ("element"), w886) -> (w884:string)
            n494 = Select(t="+Restricted" ("name or relative path"), s=w909, f="-Restricted" ("name or relative path")) -> (s? t:f=w898:string)
            n495 = Concatenate Strings(w901, w900) -> (w899:string)
            n496 = Index Array(array=w896, index=0) -> (element=w894:i32)
            n497 = for {
              N: w894 -> [_]
              tunnel: [w954] -> w893 mode=indexing
              tunnel: w884 -> [w955]
              i -> [w957]
              n498 = Equal To 0?(x=w957) -> (x = 0?=w956:bool)
              n499 = Select(t=w955, s=w956, f="") -> (s? t:f=w954:string)
            }
            n500 = Concatenate Strings(w899, w898) -> (w897:string)
            n501 = Concatenate Strings(w897, "-RIresult.txt" ("name or relative path")) -> (w951:string)
            n502 = Strip Path(path=w948) -> (stripped path=w952:path)  [unwired: 1 out]
            n503 = Build Path(base path=w952, name or relative path=w951) -> (appended path=w941:path)
            "Saved RI to this filename and path 2" <- w941
            n504 = Transpose 2D Array(2D array=w891) -> (transposed array=w890:string[][])
            n505 = Build Array (concatenate)(w893, w890) -> (w892:string[][])
            n506 = call-poly <vilib>:"Write To Spreadsheet File.vi"("transpose? (no:F)"=FALSE, "2D data"=w892, "file path (dialog if empty)"=w941) -> ()  [unwired: 5 in, 1 out]
          }
          frame #1 {
            n507 = One Button Dialog(message="File save was completed successfully") -> ()  [unwired: 1 in, 1 out]
          }
        }
      }
      frame "Save RI -Monte Carlo to file" {
        n508 = stacked-sequence {
          tunnel: w960 -> [w980 _]
          frame #0 {
            n509 = Unbundle By Name(w980) -> ("Extinction Cross section Path"=w970:path, "RI MC results.Wavelength"=w971:dbl[], "RI MC results.Real RI"=w975:dbl[], "RI MC results.Std Real RI"=w974:dbl[], "RI MC results.Imaginary RI"=w973:dbl[], "RI MC results.Std Imaginary RI"=w972:dbl[])
            n510 = Build Array(w971, w975, w974, w973, w972) -> (w969:dbl[][])
            n511 = call <vilib>:"Get File Extension.vi"("file"=w970) -> ("filename without extension"=w978:string)  [unwired: 7 in, 3 out]
            n512 = Transpose 2D Array(2D array=w969) -> (transposed array=w964:dbl[][])
            n513 = Concatenate Strings(w978, "-RI-MC-result.xls" ("name or relative path")) -> (w976:string)
            n514 = Strip Path(path=w970) -> (stripped path=w979:path)  [unwired: 1 out]
            n515 = Number To Fractional String(number=w964, precision (6)=i16 3) -> (F-format string=w965:string[][])  [unwired: 2 in]
            n516 = Build Array (concatenate)(string[] ["Wavelength (nm)", "Real Part (MC)", "Std Real Part (MC)", "Imaginary Part  (MC)", "Std Imaginary part (MC)"] ("column headers"), w965) -> (w967:string[][])
            n517 = Build Path(base path=w979, name or relative path=w976) -> (appended path=w966:path)
            "Saved RI (MC) to this filename and path" <- w966
            n518 = call-poly <vilib>:"Write To Spreadsheet File.vi"("2D data"=w967, "file path (dialog if empty)"=w966) -> ()  [unwired: 6 in, 1 out]
          }
          frame #1 {
            n519 = One Button Dialog(message="File save was completed successfully") -> ()  [unwired: 1 in, 1 out]
          }
        }
        n520 = call <vilib>:"Add State(s) to Queue__jki_lib_state_machine.vi"("State(s) in (\"\")"=w962) -> ("States Out"=w961:string)  [unwired: 14 in]
      }
      frame "Retrieve RI Monte Carlo" {
        w1005 = T16 {"Real RI"=[], "Imaginary RI"=[], "Std Imaginary RI"=[], "Std Real RI"=[], "Wavelength"=[], "Residue"=[], "Extinction Factor"=[], "Diameter Factor"=[], "Diameter Offset"=[], "Best fit result"=[], "Normalized Residuals"=[]}  # RI MC results
        n521 = call <vilib>:"Add State(s) to Queue__jki_lib_state_machine.vi"("State(s) in (\"\")"=w1032) -> ("States Out"=w1031:string)  [unwired: 14 in]
        n522 = property on="Min Wavelength" class="CmbBox"() -> ("Value"=w989:string)  [unwired: 2 in, 2 out]
        n523 = property on="Max Wavelength" class="CmbBox"() -> ("Value"=w987:string)  [unwired: 2 in, 2 out]
        n524 = Decimal String To Number(string=w989) -> (number=w988:i32)  [unwired: 2 in, 1 out]
        n525 = Decimal String To Number(string=w987) -> (number=w986:i32)  [unwired: 2 in, 1 out]
        n526 = Unbundle By Name(w1004) -> ("Extinction ExtinctionUncertainity Size parameter and Number ofS sizes"=w1026:T7, "Particle Distribution Data"=w1029:T8)
        n527 = local read "General Data for RI Retrieval VI"() -> (w982:T5)
        n528 = local read "Size Parameter Factor"() -> (w984:bool)
        n529 = local read "Size Parameter Offset"() -> (w983:bool)
        n530 = local read "Extinction Factor"() -> (w985:bool)
        n531 = Bundle(cluster=w982, "Min WaveLength Index"=w988, "Max WaveLength Index"=w986, "Extinction Factor"=w985, "Size Parameter Factor"=w984, "Size Paramter Offset"=w983) -> (w996:T5)  [unwired: 4 in]
        n532 = Unbundle By Name(w1026) -> ("Extinction"=w1028:dbl[][], "Extinction Uncertainty"=w1027:dbl[][])
        n533 = local read "Restrict to Positive Imaginary Part"() -> (w990:bool)
        n534 = local read "Size of statistics"() -> (w1006:i32)
        n535 = local read "Size of statistics"() -> (w994:i32)
        n536 = control-ref of="MC progress"() -> (w995:refnum<vi>)
        n537 = Tick Count (ms)() -> (millisecond timer value=w1007:u32)
        n538 = property class="Slide (strict)"(reference=w995, "Scale.Maximum"=w994) -> ()  [unwired: 1 in, 2 out]
        n539 = for {
          N: w1006 -> [_]
          tunnel: w1029 -> [w1067]
          tunnel: w1028 -> [w1064]
          tunnel: w1027 -> [w1063]
          tunnel: w1026 -> [w1061]
          tunnel: [w1056] -> w1025 mode=indexing
          tunnel: [w1052] -> w1014 mode=indexing
          tunnel: [w1051] -> w998
          tunnel: w1006 -> [w1046]
          shift-right: [w1043] -> _
          shift-left: w1007 -> [w1050]
          tunnel: w996 -> [w1042]
          tunnel: w995 -> [w1041]
          tunnel: [w1039] -> w993
          tunnel: w990 -> [w1035]
          i -> [w1040]
          n540 = for {
            tunnel: w1064 -> [w1073] mode=indexing
            tunnel: w1063 -> [w1072] mode=indexing
            tunnel: [w1071] -> w1062 mode=indexing
            n541 = for {
              tunnel: w1073 -> [w1081] mode=indexing
              tunnel: w1072 -> [w1079] mode=indexing
              tunnel: [w1074] -> w1071 mode=indexing
              w1078 = 1000000000.0 ("y")
              n542 = Multiply(x=w1081, y=w1078) -> (x*y=w1080:dbl)
              n543 = Multiply(x=w1079, y=w1078) -> (x*y=w1077:dbl)
              n544 = Random Number (0-1)() -> (number: 0 to 1=w1082:dbl)
              n545 = call-poly <vilib>:"Continuous Inverse CDF.vi"("std"=w1077, "mean"=w1080, "cdf(x)"=w1082) -> ("x"=w1076:dbl)  [unwired: 7 in, 1 out]
              n546 = Multiply(x=w1076, y=1e-09) -> (x*y=w1074:dbl)
            }
          }
          n547 = Tick Count (ms)() -> (millisecond timer value=w1043:u32)
          n548 = Subtract(x=w1043, y=w1050) -> (x-y=w1049:u32)
          n549 = Increment(x=w1040) -> (x+1=w1039:i32)
          n550 = property class="Slide (strict)"(reference=w1041, "Value"=w1039) -> ()  [unwired: 1 in, 2 out]
          n551 = Divide(x=w1049, y=u32 60000) -> (x/y=w1047:dbl)
          n552 = Subtract(x=w1046, y=w1040) -> (x-y=w1045:i32)
          n553 = Multiply(x=w1047, y=w1045) -> (x*y=→"Time Left (min) (MC)":dbl)
          n554 = control-ref of="Simplex"() -> (w1034:refnum<vi>)
          n555 = control-ref of="Real Part vs wavelength"() -> (w1070:refnum<vi>)
          n556 = control-ref of="Not Corrected for Multiple charge Best fit result"() -> (w1068:refnum<vi>)
          n557 = control-ref of="Imaginary Part vs wavelength"() -> (w1069:refnum<vi>)
          n558 = control-ref of="Normalized Residuals vs Size parameter"() -> (w1066:refnum<vi>)
          n559 = local read "Minimization method"() -> (w1038:u16)
          n560 = local read "Calculate Errors"() -> (w1036:bool)
          n561 = Bundle By Name(cluster=w1061, "Extinction"=w1062) -> (w1060:T7)
          n562 = Bundle("Real Part vs wavelength"=w1070, "Imaginary Part vs wavelength"=w1069, "Normalized Residuals vs Size parameter"=w1066, "Not Corrected for Multiple charge Best fit result"=w1068, "Simplex"=w1034) -> (w1065:T24)  [unwired: 1 in]
          n563 = call "RIRetrieval.vi"("Minimization method"=w1038, "Extinction Measured Data"=w1060, "Approximate Errors"="Approximate Errors", "Graph Refs"=w1065, "Particle Distribution Data"=w1067, "Calculate Errors"=w1036, "Restrict to Positive Imaginary Part"=w1035, "General Data for RI Retrieval VI"=w1042) -> ("Real Part vs wavelength"=w1059:cluster{dbl[], dbl[]}[], "Imaginary Part vs wavelength"=w1053:cluster{dbl[], dbl[]}[])  [unwired: 4 in, 2 out]
          n564 = Index Array(array=w1059, index=0) -> (element=w1057:cluster{dbl[], dbl[]})
          n565 = Index Array(array=w1053, index=0) -> (element=w1054:cluster{dbl[], dbl[]})
          n566 = Unbundle(w1054) -> (w1052:dbl[])  [unwired: 1 out]
          n567 = Unbundle(w1057) -> (w1051:dbl[], w1056:dbl[])
          "Loop index (MC)" <- w1040
        }
        n568 = call <vilib>:"Covariance Matrix.vi"("X"=w1025) -> ("mean vector"=w997:dbl[], "covariance matrix V"=w1024:T25)  [unwired: 9 in]
        n569 = call <vilib>:"Covariance Matrix.vi"("X"=w1014) -> ("mean vector"=w1001:dbl[], "covariance matrix V"=w1019:T25)  [unwired: 9 in]
        n570 = Greater?(x=w993, y=0) -> (0:w991:bool)
        n571 = case shown="True" w991 {
          frame False {
          }
          frame True {
            n572 = One Button Dialog(message="MC run finished successfully") -> ()  [unwired: 1 in, 1 out]
          }
        }
        n573 = Index Array(array=w1024) -> (element=w1023:T25)  [unwired: 2 in]
        n574 = Index Array(array=w1019) -> (element=w1018:T25)  [unwired: 2 in]
        n575 = call-poly <vilib>:"Matrix To Array.vi"("Real Matrix"=w1023) -> ("Real 2D Array"=w1022:dbl[][])
        n576 = call-poly <vilib>:"Matrix To Array.vi"("Real Matrix"=w1018) -> ("Real 2D Array"=w1017:dbl[][])
        n577 = Index Array(array=w1022, index (col)=0 ("disabled index (col)")) -> (element=w1020:dbl[])  [unwired: 1 in]
        n578 = Index Array(array=w1017, index (col)=0 ("disabled index (col)")) -> (element=w1015:dbl[])  [unwired: 1 in]
        n579 = Bundle(w998, "mean vector"=w997) -> (w1013:cluster{dbl[], "mean vector":dbl[]})  [unwired: 1 in]
        n580 = Square Root(x=w1020) -> (sqrt(x)=w999:dbl[])
        n581 = Bundle(w998, "mean vector"=w1001) -> (w1010:cluster{dbl[], "mean vector":dbl[]})  [unwired: 1 in]
        n582 = Square Root(x=w1015) -> (sqrt(x)=w1000:dbl[])
        n583 = call "XY error bars.vi"("XY plot"=w1013, "Yerror"=w999) -> ("Y error bars"=w1012:cluster{dbl[], dbl[]})  [unwired: 6 in, 2 out]
        n584 = call "XY error bars.vi"("XY plot"=w1010, "Yerror"=w1000) -> ("Y error bars"=w1009:cluster{dbl[], dbl[]})  [unwired: 6 in, 2 out]
        n585 = Bundle By Name(cluster=w1005, "Real RI"=w997, "Imaginary RI"=w1001, "Std Imaginary RI"=w1000, "Std Real RI"=w999, "Wavelength"=w998) -> (w1002:T16)
        n586 = Build Array(w1013, w1012) -> (→"Real Part MC":cluster{dbl[], "mean vector":dbl[]}[])
        n587 = Build Array(w1010, w1009) -> (→"Imaginary Part MC":cluster{dbl[], "mean vector":dbl[]}[])
        n588 = Bundle By Name(cluster=w1004, "RI MC results"=w1002) -> (w1003:T17)
      }
      frame "Retreive RI from Single Measurements(MC)" {
        w1110 = T16 {"Real RI"=[], "Imaginary RI"=[], "Std Imaginary RI"=[], "Std Real RI"=[], "Wavelength"=[], "Residue"=[], "Extinction Factor"=[], "Diameter Factor"=[], "Diameter Offset"=[], "Best fit result"=[], "Normalized Residuals"=[]}  # RI MC results
        n589 = call <vilib>:"Add State(s) to Queue__jki_lib_state_machine.vi"("State(s) in (\"\")"=w1134) -> ("States Out"=w1133:string)  [unwired: 14 in]
        n590 = property on="Min Wavelength" class="CmbBox"() -> ("Value"=w1090:string)  [unwired: 2 in, 2 out]
        n591 = property on="Max Wavelength" class="CmbBox"() -> ("Value"=w1089:string)  [unwired: 2 in, 2 out]
        n592 = Unbundle By Name(w1109) -> ("Extinction ExtinctionUncertainity Size parameter and Number ofS sizes"=w1128:T7, "Particle Distribution Data"=w1131:T8, "FullExtinctionData"=w1095:dbl[][], "NumberOfMeasurementsperSize"=w1092:i32)
        n593 = Decimal String To Number(string=w1090) -> (number=w1087:i32)  [unwired: 2 in, 1 out]
        n594 = Decimal String To Number(string=w1089) -> (number=w1088:i32)  [unwired: 2 in, 1 out]
        n595 = local write "Size of statistics"(w1092) -> ()
        n596 = local read "General Data for RI Retrieval VI"() -> (w1083:T5)
        n597 = local read "Size Parameter Factor"() -> (w1085:bool)
        n598 = local read "Size Parameter Offset"() -> (w1084:bool)
        n599 = local read "Extinction Factor"() -> (w1086:bool)
        n600 = Unbundle By Name(w1128) -> ("Number ofSizes"=w1130:dbl, "Extinction Uncertainty"=w1129:dbl[][])
        n601 = Bundle(cluster=w1083, "Min WaveLength Index"=w1087, "Max WaveLength Index"=w1088, "Extinction Factor"=w1086, "Size Parameter Factor"=w1085, "Size Paramter Offset"=w1084) -> (w1101:T5)  [unwired: 4 in]
        n602 = local read "Restrict to Positive Imaginary Part"() -> (w1091:bool)
        n603 = local read "Size of statistics"() -> (w1099:i32)
        n604 = control-ref of="MC progress"() -> (w1100:refnum<vi>)
        n605 = Tick Count (ms)() -> (millisecond timer value=w1111:u32)
        n606 = property class="Slide (strict)"(reference=w1100, "Scale.Maximum"=w1099) -> ()  [unwired: 1 in, 2 out]
        n607 = for {
          N: w1092 -> [_]
          tunnel: w1131 -> [w1171]
          tunnel: w1130 -> [w1143]
          tunnel: w1129 -> [_]
          tunnel: w1128 -> [w1168]
          tunnel: [w1163] -> w1127 mode=indexing
          tunnel: [w1159] -> w1116 mode=indexing
          tunnel: [w1158] -> w1103
          tunnel: w1092 -> [w1153]
          shift-right: [w1151] -> _
          shift-left: w1111 -> [w1157]
          tunnel: w1101 -> [w1137]
          tunnel: w1100 -> [w1150]
          tunnel: [w1149] -> w1098
          tunnel: w1095 -> [w1144]
          tunnel: w1092 -> [w1139]
          tunnel: w1091 -> [w1138]
          i -> [w1142]
          n608 = Tick Count (ms)() -> (millisecond timer value=w1151:u32)
          n609 = Subtract(x=w1151, y=w1157) -> (x-y=w1156:u32)
          n610 = Increment(x=w1142) -> (x+1=w1141:i32)
          n611 = Increment(x=w1142) -> (x+1=w1149:i32)
          n612 = mathscript code="Extinction=[];\nfor j=0:(NumOfSizes-1)\nExtinction=[Extinction FullExt(:,j*NumOfMeas+i)];\ntemp=j*NumOfMeas+i;\nend\n%Extinction=Extinction';"("FullExt"=w1144, "i"=w1141, "NumOfSizes"=w1143, "NumOfMeas"=w1139) -> ("Extinction"=w1140:dbl[][])  [unwired: 1 in, 1 out]
          n613 = property class="Slide (strict)"(reference=w1150, "Value"=w1149) -> ()  [unwired: 1 in, 2 out]
          n614 = Divide(x=w1156, y=u32 60000) -> (x/y=w1154:dbl)
          n615 = Bundle By Name(cluster=w1168, "Extinction"=w1140) -> (w1167:T7)
          n616 = Subtract(x=w1153, y=w1142) -> (x-y=w1152:i32)
          n617 = control-ref of="Simplex"() -> (w1136:refnum<vi>)
          n618 = Multiply(x=w1154, y=w1152) -> (x*y=w1146:dbl)
          n619 = control-ref of="Real Part vs wavelength"() -> (w1174:refnum<vi>)
          n620 = control-ref of="Not Corrected for Multiple charge Best fit result"() -> (w1172:refnum<vi>)
          n621 = control-ref of="Imaginary Part vs wavelength"() -> (w1173:refnum<vi>)
          n622 = control-ref of="Normalized Residuals vs Size parameter"() -> (w1170:refnum<vi>)
          n623 = local write "Time Left (min) (MC)"(w1146) -> ()
          n624 = local read "Minimization method"() -> (w1148:u16)
          n625 = local read "Approximate Errors"() -> (w1145:bool)
          n626 = local read "Calculate Errors"() -> (w1147:bool)
          n627 = Bundle("Real Part vs wavelength"=w1174, "Imaginary Part vs wavelength"=w1173, "Normalized Residuals vs Size parameter"=w1170, "Not Corrected for Multiple charge Best fit result"=w1172, "Simplex"=w1136) -> (w1169:T24)  [unwired: 1 in]
          n628 = call "RIRetrieval.vi"("Minimization method"=w1148, "Extinction Measured Data"=w1167, "Approximate Errors"=w1145, "Graph Refs"=w1169, "Particle Distribution Data"=w1171, "Calculate Errors"=w1147, "Restrict to Positive Imaginary Part"=w1138, "General Data for RI Retrieval VI"=w1137) -> ("Real Part vs wavelength"=w1166:cluster{dbl[], dbl[]}[], "Imaginary Part vs wavelength"=w1160:cluster{dbl[], dbl[]}[])  [unwired: 4 in, 2 out]
          n629 = Index Array(array=w1166, index=0) -> (element=w1164:cluster{dbl[], dbl[]})
          n630 = Index Array(array=w1160, index=0) -> (element=w1161:cluster{dbl[], dbl[]})
          n631 = Unbundle(w1164) -> (w1158:dbl[], w1163:dbl[])
          n632 = Unbundle(w1161) -> (w1159:dbl[])  [unwired: 1 out]
          "Loop index (MC) 2" <- w1142
        }
        n633 = call <vilib>:"Covariance Matrix.vi"("X"=w1127) -> ("mean vector"=w1102:dbl[], "covariance matrix V"=w1126:T25)  [unwired: 9 in]
        n634 = call <vilib>:"Covariance Matrix.vi"("X"=w1116) -> ("mean vector"=w1106:dbl[], "covariance matrix V"=w1121:T25)  [unwired: 9 in]
        n635 = Greater?(x=w1098, y=0) -> (0:w1096:bool)
        n636 = case shown="True" w1096 {
          frame False {
          }
          frame True {
            n637 = One Button Dialog(message="MC run finished successfully") -> ()  [unwired: 1 in, 1 out]
          }
        }
        n638 = Index Array(array=w1126) -> (element=w1125:T25)  [unwired: 2 in]
        n639 = Index Array(array=w1121) -> (element=w1120:T25)  [unwired: 2 in]
        n640 = call-poly <vilib>:"Matrix To Array.vi"("Real Matrix"=w1125) -> ("Real 2D Array"=w1124:dbl[][])
        n641 = call-poly <vilib>:"Matrix To Array.vi"("Real Matrix"=w1120) -> ("Real 2D Array"=w1119:dbl[][])
        n642 = Index Array(array=w1124, index (col)=0 ("disabled index (col)")) -> (element=w1122:dbl[])  [unwired: 1 in]
        n643 = Index Array(array=w1119, index (col)=0 ("disabled index (col)")) -> (element=w1117:dbl[])  [unwired: 1 in]
        n644 = Bundle(w1103, "mean vector"=w1102) -> (w1115:cluster{dbl[], "mean vector":dbl[]})  [unwired: 1 in]
        n645 = Square Root(x=w1122) -> (sqrt(x)=w1104:dbl[])
        n646 = Bundle(w1103, "mean vector"=w1106) -> (w1113:cluster{dbl[], "mean vector":dbl[]})  [unwired: 1 in]
        n647 = Square Root(x=w1117) -> (sqrt(x)=w1105:dbl[])
        n648 = call "XY error bars.vi"("XY plot"=w1115, "Yerror"=w1104) -> ("Y error bars"=w1114:cluster{dbl[], dbl[]})  [unwired: 6 in, 2 out]
        n649 = call "XY error bars.vi"("XY plot"=w1113, "Yerror"=w1105) -> ("Y error bars"=w1112:cluster{dbl[], dbl[]})  [unwired: 6 in, 2 out]
        n650 = Bundle By Name(cluster=w1110, "Real RI"=w1102, "Imaginary RI"=w1106, "Std Imaginary RI"=w1105, "Std Real RI"=w1104, "Wavelength"=w1103) -> (w1107:T16)
        n651 = Build Array(w1115, w1114) -> (w1094:cluster{dbl[], "mean vector":dbl[]}[])
        n652 = Build Array(w1113, w1112) -> (w1093:cluster{dbl[], "mean vector":dbl[]}[])
        n653 = local write "Real Part MC"(w1094) -> ()
        n654 = local write "Imaginary Part MC"(w1093) -> ()
        n655 = Bundle By Name(cluster=w1109, "RI MC results"=w1107) -> (w1108:T17)
      }
      frame "Update Window after Load Files" {
        n656 = Unbundle By Name(w1283) -> ("Extinction ExtinctionUncertainity Size parameter and Number ofS sizes.WaveLength"=w1282:dbl[])
        n657 = call <vilib>:"Add State(s) to Queue__jki_lib_state_machine.vi"("State(s) in (\"\")"=w1286) -> ("States Out"=w1285:string)  [unwired: 14 in]
        n658 = for {
          tunnel: w1282 -> [w1298] mode=indexing
          tunnel: [w1299] -> w1281 mode=indexing
          tunnel: [w1297] -> w1280 mode=indexing
          i -> [w1297]
          n659 = Number To Decimal String(number=w1297) -> (decimal integer string=w1296:string)  [unwired: 1 in]
          n660 = Number To Fractional String(number=w1298, precision (6)=i16 3) -> (F-format string=w1295:string)  [unwired: 2 in]
          n661 = Bundle(w1295, w1296) -> (w1299:cluster{string, string})  [unwired: 1 in]
        }
        n662 = flat-sequence {
          tunnel: w1281 -> [w1288]
          tunnel: w1281 -> [w1287]
          tunnel: w1280 -> [w1293]
          frame #0 {
            n663 = property on="Max Wavelength" class="CmbBox"("Strings And Values[]"=w1288) -> ()  [unwired: 2 in, 2 out]
            n664 = property on="Min Wavelength" class="CmbBox"("Strings And Values[]"=w1287) -> ()  [unwired: 2 in, 2 out]
          }
          frame #1 {
            n665 = Array Max & Min(array=w1293) -> (max value=w1289:i32, min value=w1292:i32)  [unwired: 2 out]
            n666 = Number To Decimal String(number=w1289) -> (decimal integer string=w1291:string)  [unwired: 1 in]
            n667 = Number To Decimal String(number=w1292) -> (decimal integer string=w1290:string)  [unwired: 1 in]
            n668 = property on="Max Wavelength" class="CmbBox"("Value"=w1291) -> ()  [unwired: 2 in, 2 out]
            n669 = property on="Min Wavelength" class="CmbBox"("Value"=w1290) -> ()  [unwired: 2 in, 2 out]
          }
        }
      }
      frame "Update Corrected multiple charge extinction graph" {
        w1303 = i16 3 ("precision (6)")
        n670 = call <vilib>:"Add State(s) to Queue__jki_lib_state_machine.vi"("State(s) in (\"\")"=w1364) -> ("States Out"=w1363:string)  [unwired: 14 in]
        n671 = control-ref of="Imaginary Part vs wavelength"() -> (w1359:refnum<vi>)
        n672 = Unbundle By Name(w1322) -> ("Baes data type definition"=w1344:T10, "Extinction ExtinctionUncertainity Size parameter and Number ofS sizes.WaveLength"=w1358:dbl[], "Extinction ExtinctionUncertainity Size parameter and Number ofS sizes.Extinction"=w1347:dbl[][], "Extinction ExtinctionUncertainity Size parameter and Number ofS sizes.Extinction Uncertainty"=w1348:dbl[][], "Extinction ExtinctionUncertainity Size parameter and Number ofS sizes.Size parameters"=w1350:dbl[][], "Extinction ExtinctionUncertainity Size parameter and Number ofS sizes.Number ofSizes"=w1351:dbl, "Extinction ExtinctionUncertainity Size parameter and Number ofS sizes.GeometricCrossSection"=w1352:dbl[], "Extinction ExtinctionUncertainity Size parameter and Number ofS sizes.WaveLength"=w1354:dbl[], "Particle Distribution Data.SMPS Sizes"=w1355:dbl[], "Particle Distribution Data.Concentration"=w1356:dbl[][], "Particle Distribution Data.Double Charge Correction Flag"=w1357:bool, "RI results.Extinction Factor"=w1340:dbl[], "RI results.Diameter Factor"=w1336:dbl[], "RI results.Diameter Offset"=w1335:dbl[], "RI results.Residue"=w1338:dbl[], "RI results.Real RI"=w1331:dbl[], "RI results.Std Real RI"=w1330:dbl[], "RI results.Imaginary RI"=w1329:dbl[], "RI results.Std Imaginary RI"=w1328:dbl[], "RI results.Best fit result"=w1327:dbl[][], "RI results.Normalized Residuals"=w1326:dbl[][])  [unwired: 1 out]
        n673 = property on="Property Node" class="XYGraph (strict)"(reference=w1359) -> ("Cursor.Cursor X"=w1302:dbl)  [unwired: 1 in, 2 out]
        "Wavelength" <- w1302
        n674 = Search 1D Array(1D array=w1358, element=w1302) -> (index of element=w1325:i32)  [unwired: 1 in]
        "index of element" <- w1325
        n675 = Index Array(array=w1354, index=w1325) -> (element=w1353:dbl)
        n676 = Index Array(array=w1338, index=w1325) -> (element=→"Residue (MDBF)":dbl)
        n677 = Index Array(array=w1347, index (row)=w1325) -> (element=w1346:dbl[])  [unwired: 1 in]
        n678 = Index Array(array=w1348, index (row)=w1325) -> (element=w1345:dbl[])  [unwired: 1 in]
        n679 = Index Array(array=w1350, index (row)=w1325) -> (element=w1349:dbl[])  [unwired: 1 in]
        n680 = Index Array(array=w1340, index=w1325) -> (element=w1337:dbl)
        "Extinction Factor" <- w1337
        n681 = Index Array(array=w1336, index=w1325) -> (element=w1333:dbl)
        "Diameter Factor" <- w1333
        n682 = Index Array(array=w1335, index=w1325) -> (element=w1332:dbl)
        "Diameter Offset" <- w1332
        n683 = Index Array(array=w1331, index=w1325) -> (element=w1319:dbl)
        "Real part" <- w1319
        n684 = Index Array(array=w1330, index=w1325) -> (element=w1318:dbl)
        "Real Uncertainty" <- w1318
        n685 = Index Array(array=w1328, index=w1325) -> (element=w1306:dbl)
        "Imaginary Uncertainty" <- w1306
        n686 = Index Array(array=w1329, index=w1325) -> (element=w1307:dbl)
        "Imaginary Part" <- w1307
        n687 = Index Array(array=w1327, index (row)=w1325) -> (element=w1324:dbl[])  [unwired: 1 in]
        n688 = Index Array(array=w1326, index (row)=w1325) -> (element=w1323:dbl[])  [unwired: 1 in]
        n689 = Less Than 0?(x=w1325) -> (x < 0?=w1341:bool)
        n690 = Number To Fractional String(number=w1319, precision (6)=w1303) -> (F-format string=w1317:string)  [unwired: 2 in]
        n691 = Number To Fractional String(number=w1302, precision (6)=w1303) -> (F-format string=w1301:string)  [unwired: 2 in]
        n692 = Number To Fractional String(number=w1318, precision (6)=w1303) -> (F-format string=w1315:string)  [unwired: 2 in]
        n693 = Number To Fractional String(number=w1307, precision (6)=w1303) -> (F-format string=w1312:string)  [unwired: 2 in]
        n694 = Number To Fractional String(number=w1306, precision (6)=w1303) -> (F-format string=w1310:string)  [unwired: 2 in]
        n695 = Concatenate Strings("WL=" ("string"), w1301, "nm" ("string")) -> (→"Wavelength":string)
        n696 = Concatenate Strings("n=" ("string"), w1317, "±" ("element"), w1315) -> (→"Real Part":string)
        n697 = Concatenate Strings("k=" ("string"), w1312, "±" ("element"), w1310) -> (→"Imaginary Part":string)
        n698 = Bundle By Name(cluster=w1344, "PAS amplitude"=w1346, "PAS amp Uncertainty"=w1345, "Size parameters"=w1349, "Number ofSizes"=w1351, "GeometricCrossSection"=w1352, "Wave Length"=w1353, "SMPS Sizes"=w1355, "Concentration"=w1356, "Double Charge Correction"=w1357, "Extincation Factor"=w1337) -> (w1320:T10)
        n699 = in-place {
          in-place-border: w1333 -> [w1372]
          in-place-border: w1332 -> [w1370]
          n700 = in-place-cluster #2(w1320) -> ("Size parameters"=w1376:dbl[], "Wave Length"=w1366:dbl)
          n701 = Multiply(x=w1376, y=w1366) -> (x*y=w1375:dbl[])
          n702 = Divide(x=w1375, y=3.141592653589793) -> (x/y=w1373:dbl[])
          n703 = Multiply(x=w1373, y=w1372) -> (x*y=w1371:dbl[])
          n704 = Add(x=w1371, y=w1370) -> (x+y=w1369:dbl[])
          n705 = Multiply(x=w1369, y=3.141592653589793) -> (x*y=w1367:dbl[])
          n706 = Divide(x=w1367, y=w1366) -> (x/y=w1365:dbl[])
          n707 = in-place-cluster #2("Size parameters"=w1365, "Wave Length"=w1366) -> (w1334:T10)
        }
        n708 = Bundle By Name(cluster=w1322, "Baes data type definition"=w1320) -> (w1321:T17)
        n709 = control-ref of="Real Part vs wavelength"() -> (w1361:refnum<vi>)
        n710 = control-ref of="Imaginary Part vs wavelength"() -> (w1360:refnum<vi>)
        n711 = property on="Property Node" class="XYGraph (strict)"(reference=w1361) -> ("Cursor.Cursor Y"=w1343:dbl)  [unwired: 1 in, 2 out]
        n712 = property on="Property Node" class="XYGraph (strict)"(reference=w1360) -> ("Cursor.Cursor Y"=w1342:dbl)  [unwired: 1 in, 2 out]
        n713 = case shown="False" w1341 {
          tunnel: w1334 -> [w1395 _]
          tunnel: w1343 -> [w1382 _]
          tunnel: w1342 -> [w1381 _]
          tunnel: w1320 -> [w1380 _]
          tunnel: w1324 -> [w1404 _]
          tunnel: w1323 -> [w1400 _]
          frame False {
            # "Calculate Residue (CDMRI)"
            # "Update Measured graph as well"
            n714 = call "CalculateExtinctionCorrectionsToDoublyChargeParticleContribution.vi"("refractive index, imaginary"=w1381, "refractive index, real"=w1382, "Extinction ExtinctionUncertainity Size parameter and Number ofS sizes"=w1380) -> ("Expected Extinction graph"=→"Multiple charge correction term":cluster{"Size parameters":dbl[], dbl[]}, "Expected Extinction Cross Section"=w1392:sgl[])
            n715 = call "GetAbsorptionCrossSectionsFromLinearLineRegression.vi"("Extinction ExtinctionUncertainity Size parameter and Number ofS sizes 2"=w1380, "refractive index, imaginary"=w1381, "refractive index, real"=w1382) -> ("Predicted Extinction/Absorption Cross Section"=w1377:dbl[], "Expected Extinction/Absorption Cross Section Uncer"=w1378:dbl[], "Expected Extinction/Absorption Cross Section"=w1379:dbl[])
            n716 = Subtract(x=w1377, y=w1392) -> (x-y=w1389:dbl[])
            n717 = Unbundle By Name(w1395) -> ("Size parameters"=w1391:dbl[], "Number ofSizes"=w1384:dbl)
            n718 = Subtract(x=w1379, y=w1392) -> (x-y=w1394:dbl[])
            n719 = call "CalculateAreaOfFirstPeakofSizeDistribution.vi"("Extinction ExtinctionUncertainity Size parameter and Number ofS sizes"=w1395) -> ("Area of First peak"=w1388:dbl[])
            n720 = Bundle("Size parameters"=w1391, "Expected Extinction/Absorption Cross Section"=w1379) -> (w1414:T26)  [unwired: 1 in]
            n721 = Bundle("Size parameters"=w1391, "Expected Extinction/Absorption Cross Section"=w1379) -> (w1406:T26)  [unwired: 1 in]
            n722 = Bundle("Size parameters"=w1391, "Normalized Residuals"=w1400) -> (w1402:T27)  [unwired: 1 in]
            n723 = Divide(x=w1389, y=w1388) -> (x/y=w1387:dbl[])
            n724 = Divide(x=w1394, y=w1388) -> (x/y=w1393:dbl[])
            n725 = call "PlotMieCurve.vi"("refractive index, imaginary"=w1381, "refractive index, real"=w1382, "Use Extinction Factor"=TRUE, "Extinction ExtinctionUncertainity Size parameter and Number ofS sizes"=w1395) -> ("Mie Results In Size Parameters"=w1399:sgl[], "Size parameters"=w1411:dbl[], "Extinction Crosssections"=w1412:dbl[])
            n726 = Bundle("Size parameters"=w1391, "Best fit result"=w1404) -> (w1403:T28)  [unwired: 1 in]
            n727 = Build Array(w1402) -> (w1401:T4)
            n728 = call "XY error bars.vi"("XY plot"=w1406, "Yerror"=w1378) -> ("Y error bars"=w1405:cluster{dbl[], dbl[]})  [unwired: 6 in, 2 out]
            n729 = Subtract(x=w1399, y=w1393) -> (x-y=w1398:dbl[])
            n730 = Bundle("Size parameters"=w1391, w1393) -> (w1409:cluster{"Size parameters":dbl[], dbl[]})  [unwired: 1 in]
            n731 = Build Array(w1406, w1405, w1403) -> (w1407:T29)
            n732 = property on="Normalized Residuals vs Size parameter" class="XYGraph (strict)"("Value"=w1401) -> ()  [unwired: 2 in, 2 out]
            n733 = Bundle("Size parameters"=w1391, w1387) -> (w1390:cluster{"Size parameters":dbl[], dbl[]})  [unwired: 1 in]
            n734 = Bundle("Size parameters"=w1411, "Extinction Crosssections"=w1412) -> (w1410:T22)  [unwired: 1 in]
            n735 = property on="Not Corrected for Multiple charge Best fit result" class="XYGraph (strict)"("Value"=w1407) -> ()  [unwired: 2 in, 2 out]
            n736 = call "XY error bars.vi"("XY plot"=w1409, "Yerror"=w1378) -> ("Y error bars"=w1408:cluster{dbl[], dbl[]})  [unwired: 6 in, 2 out]
            n737 = Build Array(w1409, w1414, w1410, w1408, w1390) -> (→"Corrected for multiple charge particles":T23)
            n738 = Divide(x=w1398, y=w1378) -> (x/y=w1397:dbl[])
            n739 = Square(x=w1397) -> (x^2=w1386:dbl[])
            n740 = Add Array Elements(numeric array=w1386) -> (sum=w1385:dbl)
            n741 = Divide(x=w1385, y=w1384) -> (x/y=→"Residue (CDMRI)":dbl)
          }
          frame True {
          }
        }
      }
    }
  }
